vi "UI Main.vi"() -> ()   [LabVIEW 2018]
uses:
  controls/Raw Values.ctl
  controls/VENT SYSTEM.ctl
  controls/DECOUPLERS.ctl
  controls/LNG PUGE.ctl
  controls/Control 2.ctl
  controls/LNG PURGE INDICATORS.ctl
  controls/LOX PURGE.ctl
  controls/LOX PURGE INDICATORS.ctl
  controls/DECOUPLERS INDICATORS.ctl
  Shared Variables/Control 1.ctl
  controls/In Tank Raw Voltage Measure.ctl
  Labview Training/Project/FPGA Bitfiles/Control 3.ctl
  controls/SYSTEM MEASUREMENTS.ctl
  Shared Variables/He Flow indicator.ctl
  controls/FM Indicators.ctl
  controls/Pipeline T&P.ctl
  controls/In Tank T&P.ctl
  controls/UI Data.ctl
  controls/UI Data WVFM.ctl
  controls/All FPGA Configuration Values.ctl
  controls/FPGA State.ctl
  controls/Fill Valves.ctl
  support/Logging Configuration.ctl
  support/Message Queue/Message Cluster.ctl
  controls/PID Inputs.ctl
  Globals/Global - All UI Loop Stop.vi
  Globals/Global - UI Stream and Variable Connections.vi
  COMET  Extra Programs/Globals/Global - Configuration Options WVFM.vi
  Globals/Global - Configuration Options.vi
  support/User Event - Stop/User Event - Stop.lvlib
  support/Message Queue/Message Queue.lvlib
  support/Logging.lvlib
panel:
  in  "Expansion Chassis?":bool
  out "System Measurements":T1 {"LN2 [GPM]" scale=0.004..0.02; "LN2_Temp_Coil" scale=0.0..1.6; "LN2_Temp_HEX" scale=0.0..1.6; "LNG_DST 2" scale=0.0..1.6; "LOX_DST 2" scale=0.0..1.6; "LOX_MSP" scale=0.0..0.03; "LOX_MST" scale=0.0..1.6; "LNG_MSP" scale=0.0..0.03; "LNG_MST" scale=0.0..1.6; "LOX_UST" scale=0.0..1.6; "LNG_UST" scale=0.0..1.6; "LOX_USP" scale=0.004..0.02; "LNG_USP" scale=0.004..0.02; "N2_PURGE [CFM]" scale=0.004..0.02; "LOX_DSP" scale=0.0..0.03; "LOX_DST" scale=0.0..1.6; "LNG_DSP" scale=0.0..0.03; "LNG_DST" scale=0.0..1.6}
  in  "ARM":bool
  in  "Fire Mode":T2
  out "data out":dbl
  out "System Status 9049":string="\n"
  out "Connected 9049?":bool
  in  "Connect to Controller 9049":bool
  in  "Controller Address 9049":string="169.254.85.111"
  out "LOX USP1 hide":bool
  out "LOX DSP1 hide":bool
  out "LNG DSP1 hide":bool
  out "LNG USP1 hide":bool
  out "LOX VCV Fill Close":bool=TRUE
  out "LNG VCV Fill Close":bool=TRUE
  out "LOX BV Fill Open":bool
  out "LNG BV Fill Open":bool
  in  "Exit":bool
  in  "Switch to Safe State":bool
  out "System Status":string="\n2/13/2019 8:44:05 AM: UI Error -1950679035 - Read Variable in UI Main.vi\n7/27/2018 6:11:27 PM: UI Error -1950678941 - Read Single Element from Stream in UI - Read Stream from RT 9049.vi->UI Main.vi\n12/4/2017 2:15:53 PM: UI Error -314004 - Create Network Stream Writer Endpoint in UI - Initiate Connection.vi->UI Main.vi\n12/4/2017 2:15:31 PM: UI Error -314004 - Create Network Stream Writer Endpoint in UI - Initiate Connection.vi->UI Main.vi"
  out "Current FPGA Control Mode":u16(ring) items=["Safe State", "Manual", "Control (PID)"]
  in  "Settings Tab":T3(tab)=enum."Raw Values"
  in  "Pressure\nControl":bool=TRUE
  in  "ABORT DCs":bool
  in  "MANUAL PURGE":bool
  out "LNG LOWER VOL":dbl
  out "LNG UPPER VOL":dbl
  out "LOX LOWER VOL":dbl
  out "LOX UPPER VOL":dbl
  in  "Save As Button":bool
  in  "Record Button":bool
  out "DECOUPLERS INDICATORS":T4
  out "LOX PURGE INDICATORS":T5
  in  "LOX PURGE":T6
  out "LNG PURGE INDICATORS":T7
  out "VENT SYSTEM INDICATORS":T8
  out "Boolean":bool
  in  "VENT SYSTEM":T9
  in  "Run Control":bool
  in  "Stop Control":bool
  out "9039 Time":timestamp
  in  "LNG PURGE":T10
  in  "DECOUPLERS":T11
  in  "FILL VALVES":T12 {"LOX_VCV_CTL" min=0 max=100 scale=0.0..100.0 scale format="%#_3g"; "LNG_VCV_CTL" min=0 max=100 scale=0.0..100.0 scale format="%#_3g"}
  out "Fill Valves INDICATORS":T13 {"LOX_VCV_POS" format="%.1f"; "LNG_VCV_POS" format="%.1f"}
  out "IN TANK MEASUREMENTS":T14={"LOX_ULEGE [psi]"=-0.625, "LOX_TANK"=0.0, "LOX 90%"=FALSE, "LOX 105%"=FALSE, "Depth [in] LOX "=0.0, "LNG_TANK"=217.78724947643977, "LNG 90%"=TRUE, "LNG 105%"=TRUE, "Depth [in] LNG"=41.59736465, "LNG_ULEGE [psi]"=-0.625} {"LNG_ULEGE [psi]" scale=0.0..100.0; "LNG_TANK" scale=0.0..110.0; "LOX_TANK" scale=0.0..110.0; "LOX_ULEGE [psi]" scale=0.0..100.0}
  out "9049 Time":timestamp
  in  "Reset  4":bool
  out "Total LNG DSN2 [sec]":dbl
  out "LNG DSN2 [sec]":dbl
  out "Total LOX DSN2 [sec]":dbl
  in  "Reset  6":bool
  out "LOX USN2 [sec]":dbl
  in  "Reset  5":bool
  out "Total LOX USN2 [sec]":dbl
  out "LOX DSN2 [sec]":dbl
  out "Total LNG USN2 [sec]":dbl
  out "LNG USN2 [sec]":dbl
  in  "Reset  3":bool
  out "Fill height in manual?":bool
  out "LNG Mole Unbalanced?":bool
  out "Actual Mass Ratio":dbl
  out "LNG Mass [lbs]":dbl
  out "LOX Mass [lbs]":dbl
  out "Target Mass Ratio":dbl
  out "Tank Size":T15(ring)=enum."20000lbs"
  out "Target LNG Depth [in]":dbl
  out "Target LOX Depth [in]":dbl
  out "He Flow Indicator":T16 {"LNG_HE_MFC" scale=0.0..10.0; "LOX_HE_MFC" scale=0.0..10.0}
  out "FM Meausrements":T17 {"LNG_FMF [GPM]" scale=0.0..200.0; "LOX_FMF [GPM]" scale=0.0..200.0; "LNG_FMP [psi]" scale=0.0..100.0; "LOX_FMP [psi]" scale=0.0..100.0; "LOX_FMT [F]" scale=-300.0..100.0; "LNG_FMT [F]" scale=-300.0..100.0}
  out "Pipeline T&P":T18 {"LOX UST" scale=0.0..100.0; "LOX MST" scale=0.0..100.0; "LOX DST" scale=0.0..100.0; "LNG UST" scale=0.0..100.0; "LNG MST" scale=0.0..100.0; "LNG DST" scale=0.0..100.0; "LOX USP" scale=0.0..10.0; "LOX MSP" scale=0.0..10.0; "LOX DST" scale=0.0..10.0; "LNG USP" scale=0.0..10.0; "LNG MSP" scale=0.0..10.0; "LNG DSP" scale=0.0..10.0}
  out "In Tank T&P":T19 {"LOX Tank Temp.[F]" scale=0.0..100.0; "LOX Tank Press. [psi]" scale=0.0..10.0; "LNG Tank Temp. [F]" scale=0.0..100.0; "LNG Tank Press. [psi]" scale=0.0..10.0}
  in  "NGV_N2":bool
  in  "Pessure PID":T20
  out "9237 Live Data 9049":waveform(dbl)(graph)
  in  "9237 Live Data Channel 9049":u32 max=7 step=1
  in  "9222 Live Data Channel 9049":u32 max=27 step=1
  in  "Acquire Live Data 9222 9049":bool
  in  "Acquire Live Data 9237 9049":bool
  out "9222 Live Data 9049":waveform(dbl)(graph)
  out "Most recent manually-triggered log file 9222 9049":path
  in  "Acquire Live Data 9222":bool
  in  "Force Trigger":bool
  out "Most recent manually-triggered log file 9237":path
  in  "Stop Live Data 9039":bool
  in  "Acquire Live Data 9237":bool
  in  "9237 Live Data Channel 9039":u32 max=7 step=1
  out "9237 Live Data 9039":waveform(dbl)(graph)
  out "Current Logging State 9039":u16(ring) items=["Logging", "Idle (Safe State)"]
  out "9039 Time":timestamp
  out "9222 Live Data 9039":waveform(dbl)(graph)
  in  "9222 Live Data Channel 9039":u32 max=27 step=1
  out "Most recent manually-triggered log file 9222":path
  out "9049 Time":timestamp
  out "Most recent manually-triggered log file 9237 9049":path
  in  "Stop Live Data 9049":bool
  out "Current Logging State 9049":u16(ring) items=["Logging", "Idle (Safe State)"]
  out "Actual Loop Period (ticks)":u32
  out "Largest Contiguous Memory (bytes) 9039":dbl(graph)
  out "Resource Utilization (%) 9039":cluster{dbl, "Double":dbl, "Double":dbl}(graph)
  out "Number of FIles 9039":i16
  out "Resource Utilization (%) 9049":cluster{dbl, "Double":dbl, "Double":dbl}(graph)
  out "Largest Contiguous Memory (bytes) 9049":dbl(graph)
  out "Number of FIles 9049":i16
  out "LOX":T21(graph)
  out "LNG":T22(graph)
  in  "LOX DSP Voltage Offset":dbl
  in  "LNG DSP Voltage Offset":dbl=-0.0002
  in  "N2 Voltage Offset":dbl=-0.06
  out "IN TANK MEASUREMENTS DEPTH INCHES":T23={"LNG_TANK"=41.59736465, "LOX_TANK"=0.0, "LNG_TANK 2"=10.366875, "LOX_TANK 2"=0.0} {"LOX_TANK 2" format="%_6f"; "LNG_TANK 2" format="%_6f"; "LOX_TANK" format="%_6f"; "LNG_TANK" format="%_6f"}
  in  "TTL Signals":T24
  in  "Raw Values":T25 {"LOX_VCV_POS" scale=0.0..10.0; "LNG_VCV_POS" scale=0.0..10.0}
  in  "Run Manual":bool
  in  "Stop Manual":bool
  out "SYSTEM MEASUREMENTS RAW VOLTAGE and CURRENT":T26 {"LOX_MST" format="%.4f"; "LOX_UST" format="%.4f"; "LOX_DST 2" format="%.4f"; "LOX_MSP" format="%.6f"; "LOX_USP" format="%.6f"; "LNG_MSP" format="%.6f"; "LNG_DST 2" format="%.4f"; "LNG_USP" format="%.4f"; "LNG_MST" format="%.4f"; "LNG_UST" format="%.4f"; "N2_fLOW" format="%.4f"; "LOX_FLOW" format="%.4f"; "LNG_FLOW" format="%.4f"; "LOX_DSP" format="%.6f"; "LOX_DST" format="%.4f"; "LNG_DSP" format="%.6f"; "LNG_DST" format="%.4f"; "LOX_FMP" format="%.4f"; "LNG_FMP" format="%.4f"; "LOX_FMT" format="%.4f"; "LNG_FMT" format="%.4f"}
  out "IN TANK MEASUREMENTS RAW VOLTAGE 2":T27 {"LNG_TANK_ULEGE 2" format="%_6f"; "LNG_TANK_ULEGE" format="%_6f"; "LOX_TANK_ULEGE 2" format="%_6f"; "LNG_TANK 2" format="%_6f"; "LOX_TANK 2" format="%_6f"; "LOX_DIFF" format="%_6f"; "LNG_DIFF" format="%_6f"; "LOX_TANK_ULEGE" format="%_6f"}
  in  "Manual Temp Input?":bool
  in  "Backup Sensors":T28
  in  "Tank Type":T29(ring)
  in  "Tank Size 2":T15(ring)=enum."20000lbs"
  in  "LNG Fraction":T30
  in  "Tank Sensor Adjustment":T31={"LNG THP Slope"=1.1743, "LNG THP int"=-6262.0, "LOX THP Slope"=1.1733, "LOX THP int"=-0.609, "LOX UP Slope"=1.18, "LOX UP int"=-0.6428, "LOX THP int 2"=-1.2215, "LOX THP Slope 2"=1.2498, "LNG THP int 2"=-1.2262, "LNG THP Slope 2"=1.2456, "LOX UP int 2"=-1.2057, "LOX UP Slope 2"=1.2434, "LNG UP Slope"=1.1733, "LNG UP int"=-0.6223, "LNG UP int 2"=-1.2295, "LNG UP Slope 2"=1.2441} {"LNG UP Slope 2" format="%#_13g"; "LNG UP int 2" format="%#_13g"; "LNG UP int" format="%#_13g"; "LNG UP Slope" format="%#_13g"; "LOX UP Slope 2" format="%#_13g"; "LOX UP int 2" format="%#_13g"; "LNG THP Slope 2" format="%#_13g"; "LNG THP int 2" format="%#_13g"; "LOX THP Slope 2" format="%#_13g"; "LOX THP int 2" format="%#_13g"; "LOX UP int" format="%#_13g"; "LOX UP Slope" format="%#_13g"; "LOX THP int" format="%#_13g"; "LOX THP Slope" format="%#_13g"; "LNG THP int" format="%#_13g"; "LNG THP Slope" format="%#_13g"}
  out "Connected 9039?":bool
  in  "Connect to Controller 9039":bool
  in  "Controller Address 9039":string="169.254.16.244"
  # "Not rellevant, keep hidden"
  # "COMET CONTROLS AND DAQ"
  # "Connection Settings"
  # "Offset typ 2.1V"
  # "Offset typ .0001V"
  # "Offset typ 0V"
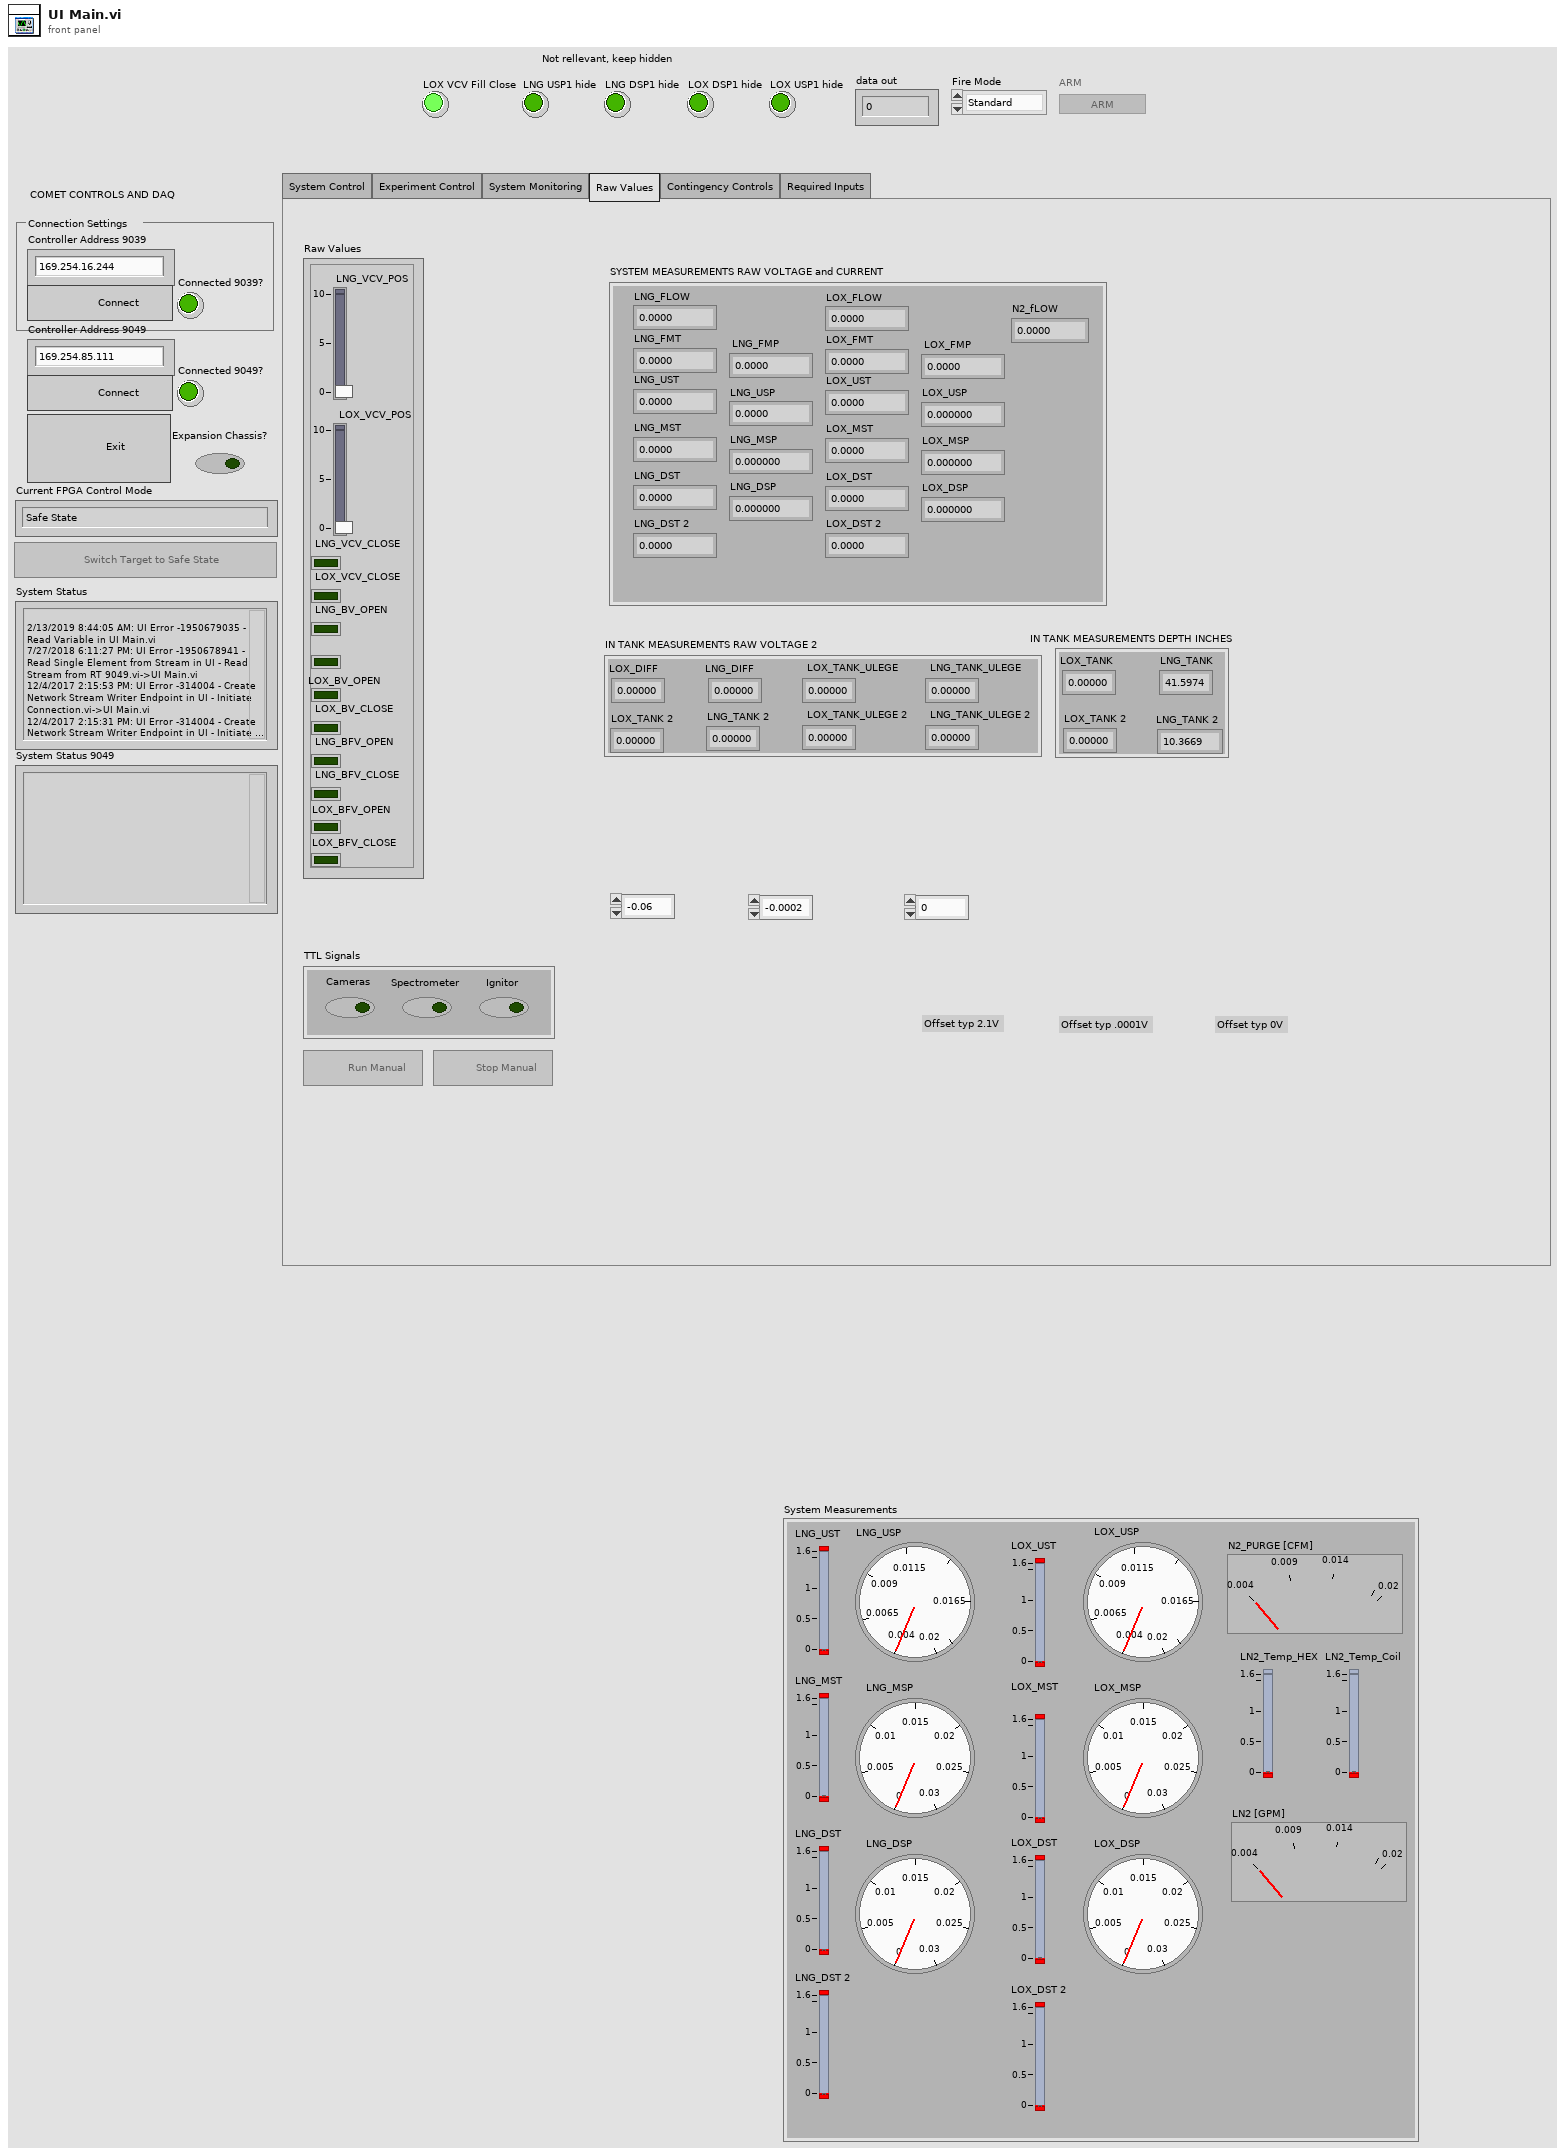
[diagram p1: front panel]
types:
  T1 = typedef "SYSTEM MEASUREMENTS.ctl" = cluster{"LNG_DST":sgl, "LNG_DSP":sgl, "LOX_DST":sgl, "LOX_DSP":sgl, "N2_PURGE [CFM]":sgl, "LNG_USP":sgl, "LOX_USP ":sgl, "LNG_UST":sgl, "LOX_UST":sgl, "LNG_MST":sgl, "LNG_MSP":sgl, "LOX_MST\n":sgl, "LOX_MSP":sgl, "LOX_DST 2":sgl, "LNG_DST 2":sgl, "LN2_Temp_HEX":sgl, "LN2_Temp_Coil":sgl, "LN2 [GPM]":sgl}
  T2 = typedef "Control 2.ctl" = enum16{"Standard", "Grill", "ROFI"}
  T3 = enum32{"System Control", "Experiment Control", "System Monitoring", "Raw Values", "Contingency Controls", "Required Inputs"}
  T4 = typedef "DECOUPLERS INDICATORS.ctl" = cluster{"LNG_DC_ENGAGED":bool, "LOX_DC_ENGAGED":bool, "LNG_DC_PROX":bool, "LOX_DC_PROX":bool}
  T5 = typedef "LOX PURGE INDICATORS.ctl" = cluster{"LOX_USP1":bool, "LOX_DSP1":bool}
  T6 = typedef "LOX PURGE.ctl" = cluster{"LOX_USP":bool, "LOX_DSP":bool}
  T7 = typedef "LNG PURGE INDICATORS.ctl" = cluster{"LNG_USP1":bool, "LNG_DSP1":bool}
  T8 = cluster{"LNG_BFV_CLOSE":bool, "LOX_BFV_CLOSE":bool, "LNG_BFV_OPEN":bool, "LOX_BFV_OPEN":bool}
  T9 = typedef "VENT SYSTEM.ctl" = cluster{"LNG_BFV":bool, "LOX_BFV":bool, "NGV_GV":bool}
  T10 = typedef "LNG PUGE.ctl" = cluster{"LNG_USP":bool, "LNG_DSP":bool}
  T11 = typedef "DECOUPLERS.ctl" = cluster{"LNG_DC":bool, "LOX_DC":bool, "NGV_DC":bool}
  T12 = cluster{"LOX_BV":bool, "LNG_BV":bool, "LNG_VCV_CTL":sgl, "LOX_VCV_CTL":sgl}
  T13 = cluster{"LNG_BV_CLOSE":bool, "LOX_BV_CLOSE":bool, "LNG_VCV_CLOSE":bool, "LNG_VCV_POS":sgl, "LOX_VCV_POS":sgl, "LNG_BV_OPEN":bool, "LOX_BV_OPEN":bool, "LOX_VCV_CLOSE":bool}
  T14 = typedef "Control 1.ctl" = cluster{"LOX_ULEGE [psi]":dbl, "LOX_TANK":dbl, "LOX 90%":bool, "LOX 105%":bool, "Depth [in] LOX ":dbl, "LNG_TANK":dbl, "LNG 90%":bool, "LNG 105%":bool, "Depth [in] LNG":dbl, "LNG_ULEGE [psi]":dbl}
  T15 = enum16{"", "150000lbs", "500lbs", "20000lbs", "9000lbs", "8000lbs", "4000lbs", "3000lbs", "2000lbs", "1000lbs"}
  T16 = typedef "He Flow indicator.ctl" = cluster{"LOX_HE_MFC":i16, "LNG_HE_MFC":i16}
  T17 = typedef "FM Indicators.ctl" = cluster{"LNG_FMT [F]":sgl, "LOX_FMT [F]":sgl, "LOX_FMP [psi]":sgl, "LNG_FMP [psi]":sgl, "LOX_FMF [GPM]":sgl, "LNG_FMF [GPM]":sgl}
  T18 = typedef "Pipeline T&P.ctl" = cluster{"LOX UST":sgl, "LOX MST":sgl, "LOX DST":sgl, "LNG UST":sgl, "LNG MST":sgl, "LNG DST":sgl, "LOX USP":sgl, "LOX MSP":sgl, "LOX DST":sgl, "LNG USP":sgl, "LNG MSP":sgl, "LNG DSP":sgl}
  T19 = typedef "In Tank T&P.ctl" = cluster{"LOX Tank Temp.[F]":sgl, "LOX Tank Press. [psi]":sgl, "LNG Tank Temp. [F]":sgl, "LNG Tank Press. [psi]":sgl}
  T20 = typedef "Control 3.ctl" = cluster{"Set Point [psi]":dbl, "Proportional (K)":dbl, "Integral (I)":dbl, "Derivative (D)":dbl}
  T21 = cluster{"LOX_VCV_POS":sgl, "LOX_FMF [GPM]":sgl, "LOX_FMT [F]":sgl, "LOX_FMP [psi]":sgl, "LOX_DST 2":sgl, "LOX_DSP":sgl, "LOX_UST":sgl, "LOX_USP ":sgl, "LOX_MST\n":sgl, "LOX_MSP":sgl}
  T22 = cluster{"LNG_VCV_POS":sgl, "LNG_FMF [GPM]":sgl, "LNG_FMT [F]":sgl, "LNG_FMP [psi]":sgl, "LNG_DST 2":sgl, "LNG_DSP":sgl, "LNG_UST":sgl, "LNG_USP":sgl, "LNG_MST":sgl, "LNG_MSP":sgl}
  T23 = cluster{"LNG_TANK":dbl, "LOX_TANK":dbl, "LNG_TANK 2":dbl, "LOX_TANK 2":dbl}
  T24 = cluster{"Cameras":bool, "Spectrometer":bool, "Ignitor":bool}
  T25 = typedef "Raw Values.ctl" = cluster{"LNG_VCV_POS":i16, " LOX_VCV_POS":i16, "LNG_VCV_CLOSE":bool, "LOX_VCV_CLOSE":bool, "LNG_BV_OPEN":bool, "LNG_BV_CLOSE":bool, "LOX_BV_OPEN":bool, "LOX_BV_CLOSE":bool, "LNG_BFV_OPEN":bool, "LNG_BFV_CLOSE":bool, "LOX_BFV_OPEN":bool, "LOX_BFV_CLOSE":bool}
  T26 = cluster{"LNG_FMT":sgl, "LOX_FMT":sgl, "LNG_FMP":sgl, "LOX_FMP":sgl, "LNG_DST":sgl, "LNG_DSP":sgl, "LOX_DST":sgl, "LOX_DSP":sgl, "LNG_FLOW [GPM]":sgl, "LOX_FLOW [GPM]":sgl, "N2_PURGE [CFM]":sgl, "LNG_UST":sgl, "LNG_MST":sgl, "LNG_USP":sgl, "LNG_DST 2":sgl, "LNG_MSP":sgl, "LOX_USP":sgl, "LOX_MSP":sgl, "LOX_DST 2":sgl, "LOX_UST":sgl, "LOX_MST":sgl}
  T27 = typedef "In Tank Raw Voltage Measure.ctl" = cluster{"LOX_TANK_ULEGE":sgl, "LNG_DIFF":sgl, "LOX_DIFF":sgl, "LOX_TANK 2":sgl, "LNG_TANK 2":sgl, "LOX_TANK_ULEGE 2":sgl, "LNG_TANK_ULEGE":sgl, "LNG_TANK_ULEGE 2":sgl}
  T28 = cluster{"LOX Tank Backup":bool, "LNG Tank Backup":bool, "LOX Ullage Backup":bool, "LNG Ullage Backup":bool}
  T29 = enum16{"Drop", "MOX", "CBM", "CBGS-New", "CBGS-Old"}
  T30 = cluster{"Methane":dbl, "Ethane":dbl, "Nitrogen":dbl, "Propane":dbl, "Isobutane":dbl}
  T31 = cluster{"LNG THP Slope":dbl, "LNG THP int":dbl, "LOX THP Slope":dbl, "LOX THP int":dbl, "LOX UP Slope":dbl, "LOX UP int":dbl, "LOX THP int 2":dbl, "LOX THP Slope 2":dbl, "LNG THP int 2":dbl, "LNG THP Slope 2":dbl, "LOX UP int 2":dbl, "LOX UP Slope 2":dbl, "LNG UP Slope":dbl, "LNG UP int":dbl, "LNG UP int 2":dbl, "LNG UP Slope 2":dbl}
  T32 = typedef "UI Data WVFM.ctl" = cluster{"Acquire Live Data 9237 9039":refnum<vi>, "Stop Live Data 9039":refnum<vi>, "Force Trigger":refnum<vi>, "Acquire Live Data 9222 9039":refnum<vi>, "Acquire Live Data 9237 9049":refnum<vi>, "Stop Live Data 9049":refnum<vi>, "Acquire Live Data 9222 9049":refnum<vi>}
  T33 = typedef "UI Data.ctl" = cluster{"Switch to Safe State Ref":refnum<vi>, "Run Manual Ref":refnum<vi>, "Stop Manual Ref":refnum<vi>, "Run Control Ref":refnum<vi>, "Stop Control Ref":refnum<vi>, "Update Control Configurations Ref":refnum<vi>, "Control Configurations Ref":refnum<vi>, "LNG_BV":refnum<vi>, "LOX_BV":refnum<vi>, "LOX DC":refnum<vi>, "LNG DC":refnum<vi>, "Record Button":refnum<vi>, "NGV DC":refnum<vi>, "LNG BFV":refnum<vi>, "LOX BFV":refnum<vi>, "Fill Valves":refnum<vi>, "VENT SYSTEM":refnum<vi>, "DECOUPLERS":refnum<vi>, "LNG Purge System":refnum<vi>, "LOX Purge System":refnum<vi>, "LOX_VCV":refnum<vi>, "LNG_VCV":refnum<vi>, "NGV N2":refnum<vi>, "MANUAL PURGE":refnum<vi>, "Turn on Pressure Control":refnum<vi>, "Pressure PID":refnum<vi>}
  T34 = typedef "Message Queue.lvlib/All Message Queues.ctl" = cluster{"UI":refnum<queue>, "UI System Record":refnum<queue>}
  T35 = cluster{"Message":string, "Message Data":variant}
  T36 = typedef "All FPGA Configuration Values.ctl" = cluster{"FPGA State":T37, "Manual Values":T25, "Fill Valves":T38, "LNG Purge System":T10, "LOX Purge System":T6, "DECOUPLERS":T11, "VENT SYSTEM":T9}
  T37 = typedef "FPGA State.ctl" = enum16{"Safe State", "Manual", "Control"}
  T38 = typedef "Fill Valves.ctl" = cluster{"LOX_BV":bool, "LNG_BV":bool, "LNG_VCV_CTL":sgl, "LOX_VCV_CTL":sgl}
  T39 = typedef "Message Queue.lvlib/Message Cluster.ctl" = cluster{"Message":string, "Message Data":variant}
  T40 = typedef "PID Inputs.ctl" = cluster{"Setpoint":dbl, "proportional gain (Kc)":dbl, "integral time (Ti, min)":dbl, "derivative time (Td, min)":dbl, "output high":dbl, "output low":dbl}
  T41 = enum8{"Enabled", "Disabled", "Disabled and Grayed Out"}
  T42 = typedef "Variable References.ctl" = cluster{"CPU Usage":refnum<k21>, "Contiguous Memory":refnum<k21>, " VALVE POSITIONS":refnum<k21>, "FPGA Mode":refnum<k21>, "Actual Loop Period":refnum<k21>, "FILL VALVES IND":refnum<k21>, "VENT SYSTEM IND":refnum<k21>, "LNG PURGE IND":refnum<k21>, "Drive Space":refnum<k21>, "Buffer Backlog":refnum<k21>, "System Time":refnum<k21>, "Number of Data Files":refnum<k21>, "LOX PURGE IND":refnum<k21>, "SYSTEM MEASURMENTS":refnum<k21>, "TEST TANK MEASURMENTS":refnum<k21>, "DECOUPLERS IND":refnum<k21>, "CPU Usage 9049":refnum<k21>, "Contiguous Memory 9049":refnum<k21>, "Drive Space 9049":refnum<k21>, "Buffer Backlog 9049":refnum<k21>, "Actual Loop Period 9049":refnum<k21>, "System Time 9049":refnum<k21>, "Number of Data Files 9049":refnum<k21>, "Number of Data Files 9050":refnum<k21>, "FM indicators":refnum<k21>, "He Flow indicator":refnum<k21>, "Pipeline T&P":refnum<k21>, "In tank T&P":refnum<k21>}
  T43 = cluster{"CPU Usage 9049":refnum<k21>, "Contiguous Memory 9049":refnum<k21>, "Drive Space 9049":refnum<k21>, "Buffer Backlog 9049":refnum<k21>, "Actual Loop Period 9049":refnum<k21>, "System Time 9049":refnum<k21>, "Number of Data Files 9049":refnum<k21>}
  T44 = typedef "Logging.lvlib/Logging Configuration.ctl" = cluster{"Log File Base Path":path, "TDMS File Reference":refnum<k34>, "Log File Path SYSTEM":path}
  T45 = enum16{"Left Button", "Center Button", "Right Button", "Window Close"}
  T46 = typedef "FILL VALVES INDICATORS.ctl" = cluster{"LNG_BV_CLOSE":bool, "LOX_BV_CLOSE":bool, "LNG_VCV_CLOSE":bool, "LNG_VCV_POS":sgl, "LOX_VCV_POS":sgl, "LNG_BV_OPEN":bool, "LOX_BV_OPEN":bool, "LOX_VCV_CLOSE":bool}
  T47 = typedef "VENT SYSTEM INDICATORS.ctl" = cluster{"LNG_BFV_CLOSE":bool, "LOX_BFV_CLOSE":bool, "LNG_BFV_OPEN":bool, "LOX_BFV_OPEN":bool}
  T48 = typedef "IN TANK MEASUREMENTS.ctl" = cluster{"LOX_TANK_ULEGE":sgl, "LNG_DIFF":sgl, "LOX_DIFF":sgl, "LOX_TANK 2":sgl, "LNG_TANK 2":sgl, "LOX_TANK_ULEGE 2":sgl, "LNG_TANK_ULEGE":sgl, "LNG_TANK_ULEGE 2":sgl}
  T49 = cluster{"Timestamp":timestamp, "Setpoint [psi]":dbl, "LOX Pressure [psi]":dbl, "LNG Pressure[psi]":dbl, "Diff. Pressure-Window [psi]":dbl, "LOX_HE_MFC":dbl, "LNG_HE_MFC":dbl}
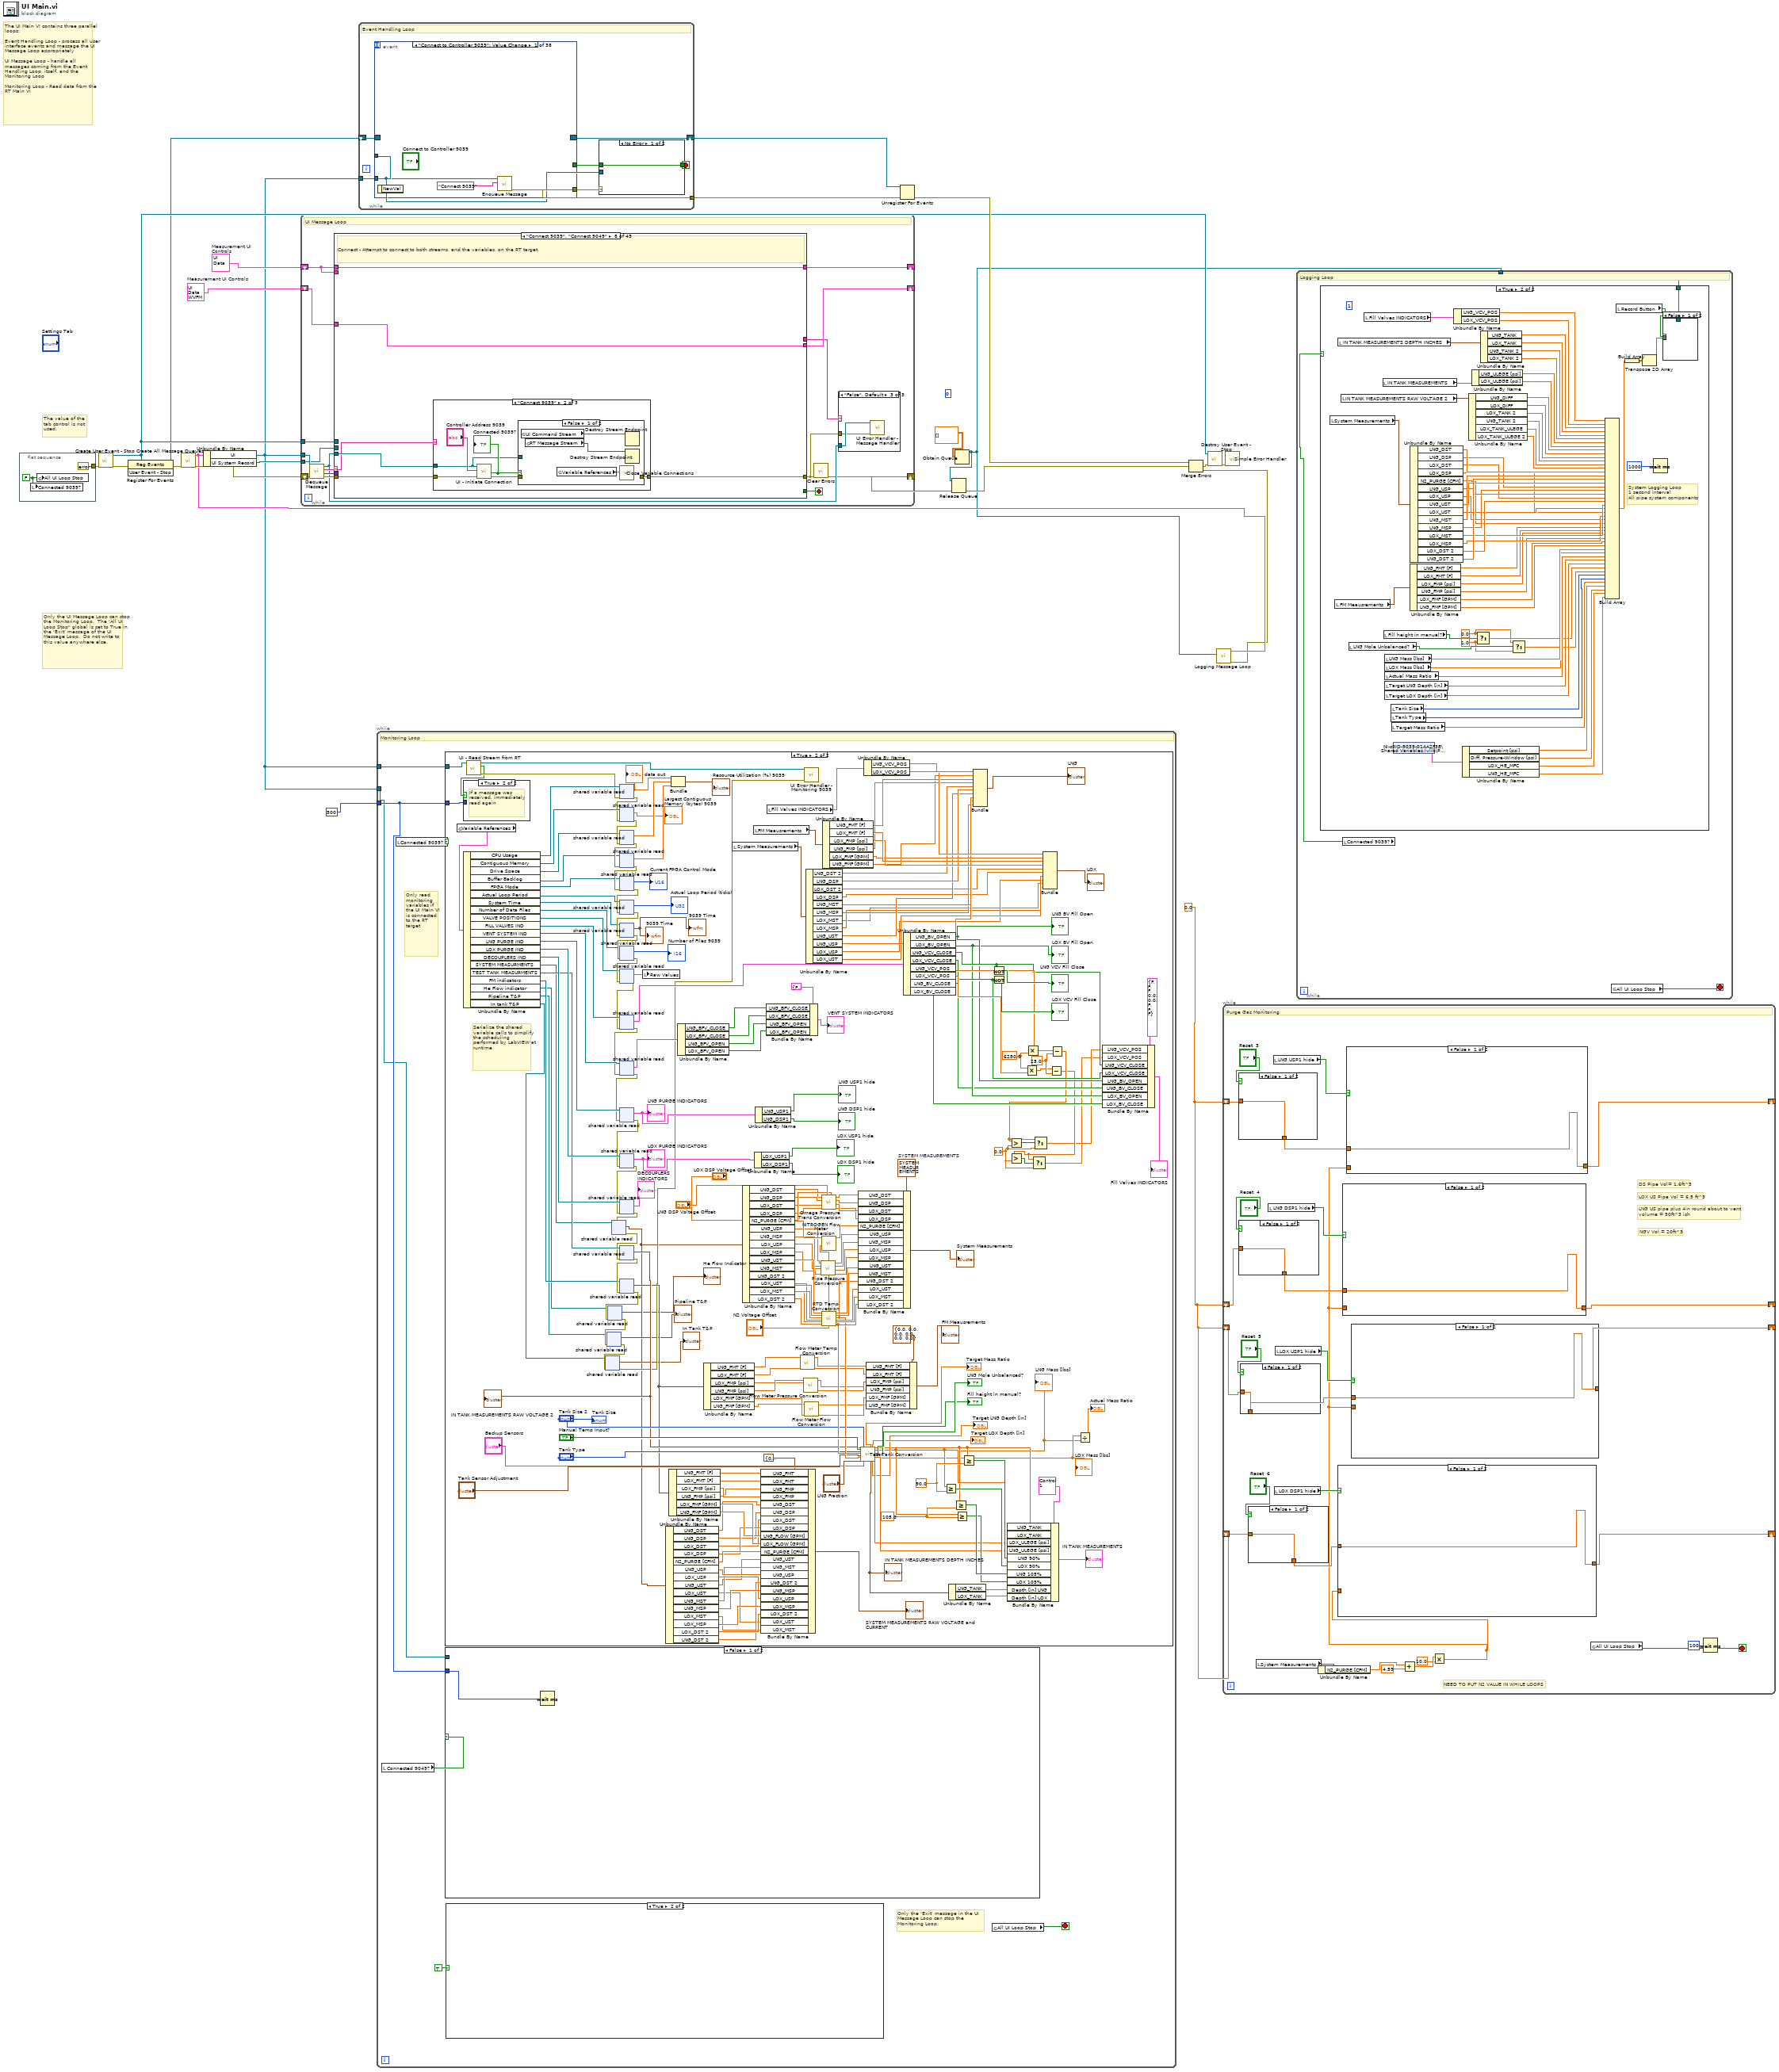
[diagram p0: block diagram]
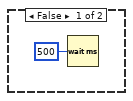
[diagram p2: hidden frame]
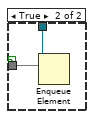
[diagram p3: hidden frame]
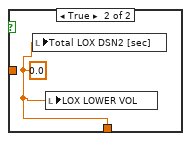
[diagram p4: hidden frame]
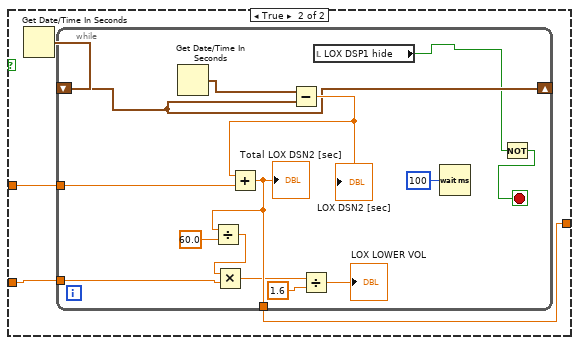
[diagram p5: hidden frame]
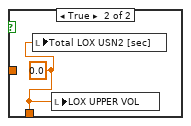
[diagram p6: hidden frame]
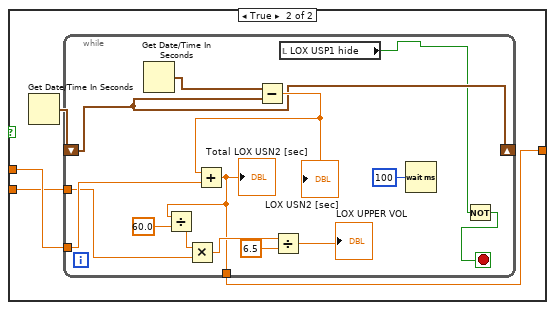
[diagram p7: hidden frame]
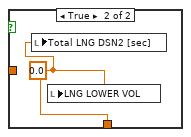
[diagram p8: hidden frame]
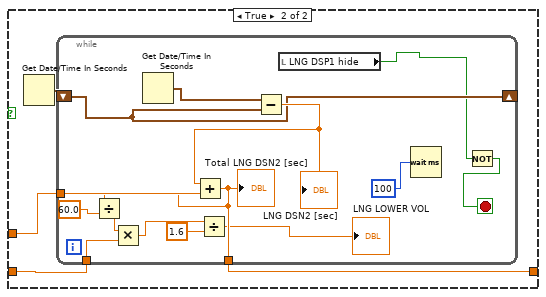
[diagram p9: hidden frame]
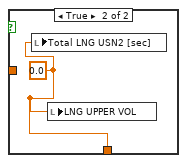
[diagram p10: hidden frame]
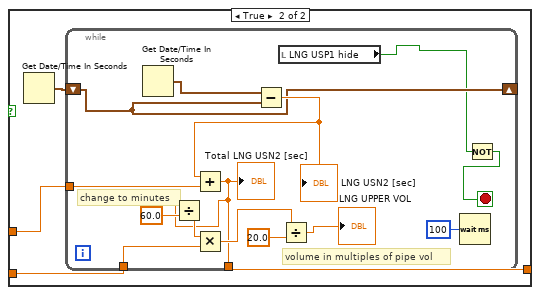
[diagram p11: hidden frame]
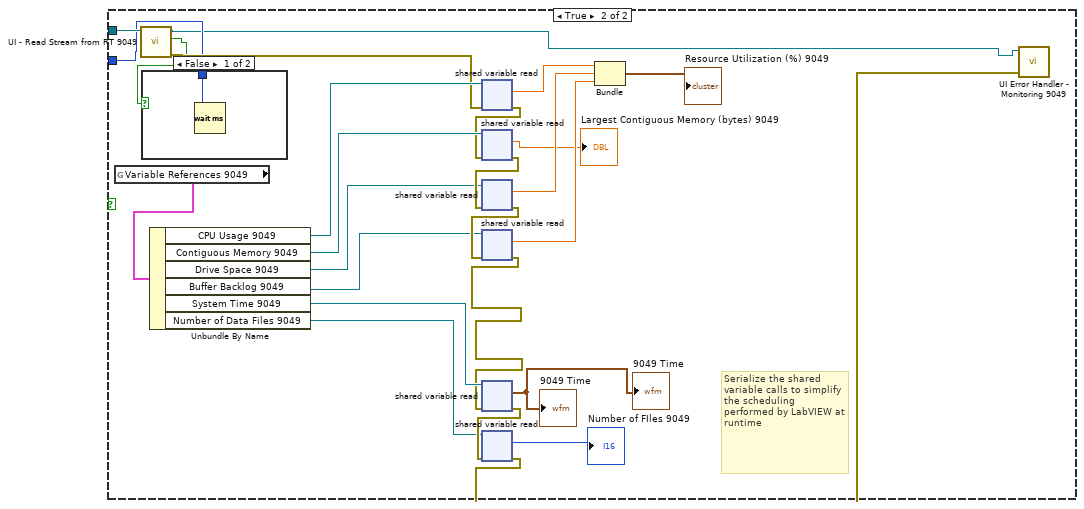
[diagram p13: hidden frame]
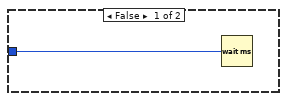
[diagram p15: hidden frame]
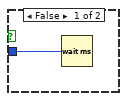
[diagram p16: hidden frame]
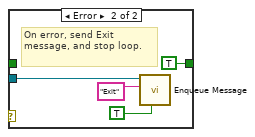
[diagram p17: hidden frame]
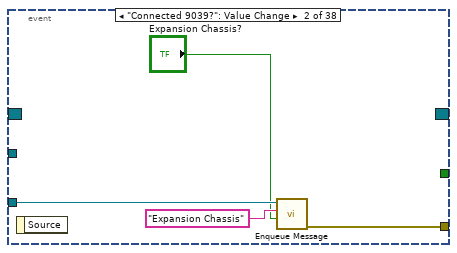
[diagram p18: hidden frame]
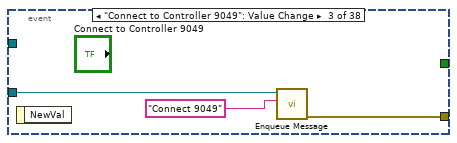
[diagram p19: hidden frame]
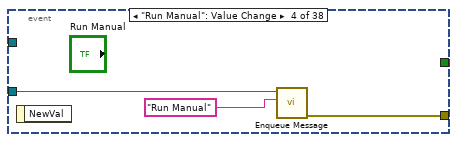
[diagram p20: hidden frame]
diagram:
  (unwired) i16 0 ("LOX_DST")
  w1 = 0.0
  w10 = T32 {"Acquire Live Data 9237 9039"=refnum, "Stop Live Data 9039"=refnum, "Force Trigger"=refnum, "Acquire Live Data 9222 9039"=refnum, "Acquire Live Data 9237 9049"=refnum, "Stop Live Data 9049"=refnum, "Acquire Live Data 9222 9049"=refnum}  # Measurement UI Controls
  w18 = T33 {"Switch to Safe State Ref"=refnum, "Run Manual Ref"=refnum, "Stop Manual Ref"=refnum, "Run Control Ref"=refnum, "Stop Control Ref"=refnum, "Update Control Configurations Ref"=refnum, "Control Configurations Ref"=refnum, "LNG_BV"=refnum, "LOX_BV"=refnum, "LOX DC"=refnum, "LNG DC"=refnum, "Record Button"=refnum, "NGV DC"=refnum, "LNG BFV"=refnum, "LOX BFV"=refnum, "Fill Valves"=refnum, "VENT SYSTEM"=refnum, "DECOUPLERS"=refnum, "LNG Purge System"=refnum, "LOX Purge System"=refnum, "LOX_VCV"=refnum, "LNG_VCV"=refnum, "NGV N2"=refnum, "MANUAL PURGE"=refnum, "Turn on Pressure Control"=refnum, "Pressure PID"=refnum}  # Measurement UI Controls
  # "The UI Main VI contains three parallel loops:\n\nEvent Handling Loop - process all user interface events and message the UI Message Loop appropriately\n\nUI Message Loop - handle all messages coming from the Event Handling Loop, itself, and the Monitoring Loop\n\nMonitoring Loop - Read data from the RT Main VI"
  # "The value of the tab control is not used."
  # "Only the UI Message Loop can stop the Monitoring Loop.  The 'All UI Loop Stop\" global is set to True in the 'Exit' message of the UI Message Loop.  Do not write to this value anywhere else."
  n1 = flat-sequence {
    tunnel: [errorcluster {"status"=FALSE, "code"=0, "source"=""} ("error in (no error)")] -> w16
    frame #0 {
      w24 = FALSE
      n2 = local write "Connected 9039?"(w24) -> ()
      n3 = global write "Global - All UI Loop Stop.vi" "All UI Loop Stop"(w24) -> ()
    }
  }
  n4 = call "Create User Event - Stop.vi"("error in (no error)"=w16) -> ("error out"=w14:errorcluster, "User Event - Stop"=w12:refnum<user-event>)  [unwired: 9 in]
  n5 = register-events(error in=w14, w12) -> (reference out=w11:refnum<event-registration>, error out=w13:errorcluster)  [unwired: 1 in]
  n6 = call "Create All Message Queues.vi"("error in (no error)"=w13) -> ("error out"=w21:errorcluster, "Message Queues out"=w8:T34)  [unwired: 9 in]
  n7 = Unbundle By Name(w8) -> ("UI"=w3:refnum<queue>, "UI System Record"=w9:refnum<queue>)
  n8 = while {
    tunnel: w3 -> [w35]
    tunnel: w12 -> [w40]
    shift-right: [w31] -> w5
    shift-left: w21 -> [w39]
    shift-right: [w34] -> _
    shift-left: w18 -> [w26]
    shift-right: [w29] -> _
    shift-left: w10 -> [w30]
    tunnel: w9 -> [w28]
    stop <- w41 stop-if-true
    # "UI Message Loop"
    n9 = call "Dequeue Message.vi"("error in (no error)"=w39, "Message Queue"=w35) -> ("error out"=w38:errorcluster, "Message Data"=w36:variant, "Message"=w37:string, "dup Message Queue"=w33:refnum<queue>)  [unwired: 6 in]
    n10 = case "Message Cases" shown="\"Connect 9039\", \"Connect 9049\"" w37 {
      selector: w37 -> [_ _ _ w101 _ _ w218 w231 w264 w284 _ _ w334 w355 w373 _ w405 w425 w450 w487 w525 w561 w588 w616 w638 w667 w681 w695 w705 w736 w747 _ _ _ _ w921 _ _ _ _ w1005 w1039 w1067]
      tunnel: w33 -> [w51 w75 w91 _ w204 w211 _ w234 _ w286 _ w322 w335 w356 _ _ _ _ _ _ _ _ _ _ _ _ _ _ _ _ _ _ _ _ w909 w925 _ _ w992 _ w1004 w1038 _]
      tunnel: w38 -> [w53 w84 w100 w104 w205 w215 w220 w236 w267 w288 w309 w331 w337 w358 w374 w388 w402 w423 w452 w489 w526 w562 w589 w617 w640 w668 w682 w696 w709 w741 w750 w769 w799 w863 w917 w934 w956 w975 w997 w1003 w1009 w1043 _]
      tunnel: [w52 w76 w92 w104 w205 w215 w217 w233 w267 w287 w308 w325 w336 w357 w375 w389 w404 w427 w447 w484 w527 w563 w590 w618 w639 w669 w683 w697 w709 w741 w750 w769 w798 w862 w911 w935 w954 w973 w998 w1002 w1008 w1042 w1065] -> w32
      tunnel: [_ _ _ _ _ _ _ _ _ _ _ _ _ _ _ _ _ _ _ _ _ _ _ _ _ _ _ _ _ _ _ _ _ _ _ _ _ _ TRUE _ _ _ _] -> w41
      tunnel: w36 -> [_ _ _ _ _ _ w219 _ _ _ _ w329 _ _ w372 w387 _ w424 w451 w488 w524 w558 w585 w613 _ w666 w680 w694 w708 w740 w749 _ w797 w861 w916 w932 w953 w972 _ _ _ _ _]
      tunnel: w40 -> [_ _ _ _ _ _ _ _ _ _ _ _ _ _ _ _ _ _ _ _ _ _ _ _ _ _ _ _ _ _ _ _ _ _ _ _ _ _ w996 _ _ _ _]
      tunnel: w26 -> [w54 w83 w99 w103 w206 w216 w223 w235 w266 w289 w310 w326 w338 w359 w376 w391 w407 w432 w453 w490 w521 w538 w583 w611 w643 w663 w677 w691 w711 w742 w751 w770 w778 w865 w915 w936 w955 w974 w994 w1001 w1007 w1041 w1063]
      tunnel: [w54 w82 w98 w103 w206 w216 w223 w235 w266 w289 w310 w326 w338 w359 w376 w391 w407 w432 w453 w490 w521 w538 w583 w611 w643 w663 w677 w691 w711 w742 w751 w770 w778 w865 w915 w936 w955 w974 w994 w1001 w1007 w1041 w1063] -> w34
      tunnel: w30 -> [w49 w73 w87 w102 w203 w213 w222 w232 w265 w285 w306 w321 w332 w353 w370 w384 w400 w430 w448 w485 w522 w559 w586 w614 w644 w664 w678 w692 w706 w739 w748 w768 w789 w864 w913 w919 w944 w964 w988 w1000 w1006 w1040 w1062]
      tunnel: [w49 w72 w87 w102 w203 w213 w222 w232 w265 w285 w306 w321 w332 w353 w370 w384 w400 w430 w448 w485 w522 w559 w586 w614 w644 w664 w678 w692 w706 w739 w748 w768 w789 w864 w913 w919 w944 w964 w988 w1000 w1006 w1040 w1062] -> w29
      tunnel: w28 -> [_ _ _ _ _ _ _ _ _ _ _ _ _ _ _ w390 w406 _ _ _ _ _ _ _ _ _ _ _ _ _ _ _ _ _ _ _ _ _ w985 _ _ _ _]
      tunnel: [_ _ _ _ _ _ _ _ _ _ _ _ _ _ _ _ _ _ _ _ _ _ _ _ _ _ _ _ _ _ _ _ _ _ _ w918 _ _ _ _ _ _ _] -> w27
      tunnel: w26 -> [_ _ _ _ _ _ _ _ _ _ _ _ _ _ _ _ _ _ _ _ _ _ _ _ _ _ _ _ _ _ _ _ _ w858 _ _ _ _ _ _ _ _ _]
      frame "Initialize" {
        # "Initialize - Send 'Initialize UI Refs' message to get the UI references bundled and initialized appropriately."
        n11 = local write "Pressure\nControl"(FALSE ("Pressurization Control")) -> ()
        n12 = call "Enqueue Message.vi"("error in (no error)"=w53, "Message"="Initialize UI Refs", "Message Queue"=w51) -> ("error out"=w52:errorcluster)  [unwired: 7 in, 1 out]
      }
      frame "Initialize UI Refs" {
        # "Send a message to disable them all, since there is no connection at the start."
        # "Initialize UI Refs - Bundle up a cluster of references of all UI elements that are programmatically manipulated."
        n13 = control-ref of="Record Button"() -> (w62:refnum<vi>)
        n14 = control-ref of="LOX PURGE"() -> (w63:refnum<vi>)
        n15 = control-ref of="FILL VALVES"() -> (w67:refnum<vi>)
        n16 = control-ref of="VENT SYSTEM"() -> (w66:refnum<vi>)
        n17 = control-ref of="DECOUPLERS"() -> (w64:refnum<vi>)
        n18 = control-ref of="PURGE SYSTEM"() -> (w65:refnum<vi>)
        n19 = control-ref of="LNG_VCV_CTL"() -> (w58:refnum<vi>)
        n20 = control-ref of="LOX_VCV_CTL"() -> (w57:refnum<vi>)
        n21 = control-ref of="Stop Live Data 9049"() -> (w60:refnum<vi>)
        n22 = control-ref of="Acquire Live Data 9222"() -> (w68:refnum<vi>)
        n23 = control-ref of="Acquire Live Data 9237 9049"() -> (w61:refnum<vi>)
        n24 = control-ref of="Force Trigger"() -> (w69:refnum<vi>)
        n25 = control-ref of="Stop Live Data 9039"() -> (w70:refnum<vi>)
        n26 = control-ref of="Acquire Live Data 9237"() -> (w71:refnum<vi>)
        n27 = control-ref of="Acquire Live Data 9222 9049"() -> (w59:refnum<vi>)
        n28 = control-ref of="Pressure\nControl"() -> (w55:refnum<vi>)
        n29 = control-ref of="Switch to Safe State"() -> (w81:refnum<vi>)
        n30 = control-ref of="Run Manual"() -> (w80:refnum<vi>)
        n31 = control-ref of="Stop Manual"() -> (w79:refnum<vi>)
        n32 = control-ref of="Run Control"() -> (w78:refnum<vi>)
        n33 = control-ref of="Stop Control"() -> (w77:refnum<vi>)
        n34 = control-ref of="Pessure PID"() -> (w56:refnum<vi>)
        n35 = call "Enqueue Message.vi"("error in (no error)"=w84, "Message"="Initialize UI Refs 2", "Message Queue"=w75) -> ("error out"=w76:errorcluster)  [unwired: 7 in, 1 out]
        n36 = Bundle By Name(cluster=w73, "Acquire Live Data 9237 9039"=w71, "Stop Live Data 9039"=w70, "Force Trigger"=w69, "Acquire Live Data 9222 9039"=w68, "Acquire Live Data 9237 9049"=w61, "Stop Live Data 9049"=w60, "Acquire Live Data 9222 9049"=w59) -> (w72:T32)
        n37 = Bundle By Name(cluster=w83, "Switch to Safe State Ref"=w81, "Run Manual Ref"=w80, "Stop Manual Ref"=w79, "Run Control Ref"=w78, "Stop Control Ref"=w77, "LOX Purge System"=w63, "Fill Valves"=w67, "VENT SYSTEM"=w66, "DECOUPLERS"=w64, "LNG Purge System"=w65, "Record Button"=w62, "LNG_VCV"=w58, "LOX_VCV"=w57, "Turn on Pressure Control"=w55, "Pressure PID"=w56) -> (w82:T33)
      }
      frame "Initialize UI Refs 2" {
        # "Send a message to disable them all, since there is no connection at the start."
        # "Initialize UI Refs - Bundle up a cluster of references of all UI elements that are programmatically manipulated."
        n38 = control-ref of="LNG_BV"() -> (w88:refnum<vi>)
        n39 = control-ref of="LOX_BV"() -> (w89:refnum<vi>)
        n40 = control-ref of="NGV_N2"() -> (w86:refnum<vi>)
        n41 = control-ref of="MANUAL PURGE"() -> (w85:refnum<vi>)
        n42 = control-ref of="LNG_DC"() -> (w97:refnum<vi>)
        n43 = control-ref of="LOX_DC"() -> (w96:refnum<vi>)
        n44 = control-ref of="NGV_DC"() -> (w95:refnum<vi>)
        n45 = control-ref of="LNG_BFV"() -> (w94:refnum<vi>)
        n46 = control-ref of="LOX_BFV"() -> (w93:refnum<vi>)
        n47 = call "Enqueue Message.vi"("error in (no error)"=w100, "Message"="Disable Controls", "Message Queue"=w91) -> ("error out"=w92:errorcluster)  [unwired: 7 in, 1 out]
        n48 = Bundle By Name(cluster=w99, "LNG DC"=w97, "LOX DC"=w96, "NGV DC"=w95, "LNG BFV"=w94, "LOX BFV"=w93, "LNG_BV"=w88, "LOX_BV"=w89, "NGV N2"=w86, "MANUAL PURGE"=w85) -> (w98:T33)
      }
      frame "Disable Controls", "Disable Controls 9039", "Disable Controls 9049" {
        # "Disable All Controls - Set all controls in the UI Refs cluster to \"Disabled and Grayed Out\"."
        n49 = case shown="\"Disable Controls\"" w101 {
          tunnel: w103 -> [_ w149 w190 _]
          tunnel: w102 -> [_ w126 w160 w195]
          frame "False", Default {
          }
          frame "Disable Controls" {
            w112 = 0
            # "Changed 1/7  LOX purge and below were not connected"
            # "With the control options disabled, the only thing the user can do is Connect. Make sure the IP address string and connect button are enabled."
            n50 = Unbundle(w149) -> ("Switch to Safe State Ref"=w148:refnum<vi>, "Run Manual Ref"=w147:refnum<vi>, "Stop Manual Ref"=w146:refnum<vi>, "Run Control Ref"=w145:refnum<vi>, "Stop Control Ref"=w144:refnum<vi>, "Update Control Configurations Ref"=w143:refnum<vi>, "Control Configurations Ref"=w142:refnum<vi>, "LNG_BV"=w141:refnum<vi>, "LOX_BV"=w140:refnum<vi>, "LOX DC"=w139:refnum<vi>, "LNG DC"=w138:refnum<vi>, "Record Button"=w137:refnum<vi>, "NGV DC"=w136:refnum<vi>, "LNG BFV"=w135:refnum<vi>, "LOX BFV"=w134:refnum<vi>, "Fill Valves"=w124:refnum<vi>, "VENT SYSTEM"=w123:refnum<vi>, "DECOUPLERS"=w122:refnum<vi>, "LNG Purge System"=w121:refnum<vi>, "LOX Purge System"=w108:refnum<vi>, "LOX_VCV"=w109:refnum<vi>, "LNG_VCV"=w110:refnum<vi>, "NGV N2"=w111:refnum<vi>, "MANUAL PURGE"=w107:refnum<vi>, "Turn on Pressure Control"=w106:refnum<vi>, "Pressure PID"=w105:refnum<vi>)
            n51 = Unbundle(w126) -> ("Acquire Live Data 9237 9039"=w130:refnum<vi>, "Stop Live Data 9039"=w129:refnum<vi>, "Force Trigger"=w128:refnum<vi>, "Acquire Live Data 9222 9039"=w125:refnum<vi>, "Acquire Live Data 9237 9049"=w115:refnum<vi>, "Stop Live Data 9049"=w114:refnum<vi>, "Acquire Live Data 9222 9049"=w113:refnum<vi>)
            n52 = control-ref of="Cameras"() -> (w120:refnum<vi>)
            n53 = control-ref of="Ignitor"() -> (w119:refnum<vi>)
            n54 = control-ref of="Spectrometer"() -> (w118:refnum<vi>)
            n55 = Build Array(w148, w147, w146, w145, w144, w143, w142, w141, w140, w139, w138, w137, w136, w135, w134, w124, w123, w122, w121, w108, w109, w110, w111, w107, w106, w105) -> (w133:refnum<vi>[])
            n56 = Build Array(w130, w129, w128, w125, w115, w114, w113) -> (w127:refnum<vi>[])
            n57 = Build Array(w120, w119, w118) -> (w116:refnum<vi>[])
            n58 = call "Set Enable State on Multiple Controls.vi"("Enable?"=FALSE, "Controls"=w127) -> ()  [unwired: 10 in]
            n59 = call "Set Enable State on Multiple Controls.vi"("Enable?"=FALSE, "Controls"=w133) -> ()  [unwired: 10 in]
            n60 = call "Set Enable State on Multiple Controls.vi"("Enable?"=TRUE, "Controls"=w116) -> ()  [unwired: 10 in]
            n61 = property on="Controller Address 9049" class="Str"("DisabledEnum"=w112) -> ()  [unwired: 2 in, 2 out]
            n62 = property on="Connect to Controller 9049" class="Bool"("DisabledEnum"=w112) -> ()  [unwired: 2 in, 2 out]
            n63 = property on="Controller Address 9039" class="Str"("DisabledEnum"=w112) -> ()  [unwired: 2 in, 2 out]
            n64 = property on="Connect to Controller 9039" class="Bool"("DisabledEnum"=w112) -> ()  [unwired: 2 in, 2 out]
          }
          frame "Disable Controls 9039" {
            w161 = 0
            # "With the control options disabled, the only thing the user can do is Connect. Make sure the IP address string and connect button are enabled."
            n65 = Unbundle By Name(w160) -> ("Acquire Live Data 9237 9039"=w159:refnum<vi>, "Stop Live Data 9039"=w158:refnum<vi>, "Acquire Live Data 9222 9039"=w157:refnum<vi>)
            n66 = Unbundle(w190) -> ("Switch to Safe State Ref"=w189:refnum<vi>, "Run Manual Ref"=w188:refnum<vi>, "Stop Manual Ref"=w187:refnum<vi>, "Run Control Ref"=w186:refnum<vi>, "Stop Control Ref"=w185:refnum<vi>, "Update Control Configurations Ref"=w184:refnum<vi>, "Control Configurations Ref"=w183:refnum<vi>, "LNG_BV"=w182:refnum<vi>, "LOX_BV"=w181:refnum<vi>, "LOX DC"=w180:refnum<vi>, "LNG DC"=w179:refnum<vi>, "Record Button"=w178:refnum<vi>, "NGV DC"=w177:refnum<vi>, "LNG BFV"=w176:refnum<vi>, "LOX BFV"=w175:refnum<vi>, "Fill Valves"=w171:refnum<vi>, "VENT SYSTEM"=w170:refnum<vi>, "DECOUPLERS"=w169:refnum<vi>, "LNG Purge System"=w168:refnum<vi>, "LOX Purge System"=w162:refnum<vi>, "LOX_VCV"=w155:refnum<vi>, "LNG_VCV"=w154:refnum<vi>, "NGV N2"=w153:refnum<vi>, "MANUAL PURGE"=w152:refnum<vi>, "Turn on Pressure Control"=w151:refnum<vi>, "Pressure PID"=w150:refnum<vi>)
            n67 = control-ref of="Cameras"() -> (w167:refnum<vi>)
            n68 = control-ref of="Ignitor"() -> (w166:refnum<vi>)
            n69 = control-ref of="Spectrometer"() -> (w165:refnum<vi>)
            n70 = Build Array(w189, w188, w187, w186, w185, w184, w183, w182, w181, w180, w179, w178, w177, w176, w175, w171, w170, w169, w168, w162, w155, w154, w153, w152, w151, w150) -> (w174:refnum<vi>[])
            n71 = Build Array(w167, w166, w165) -> (w163:refnum<vi>[])
            n72 = Build Array(w159, w158, w157) -> (w156:refnum<vi>[])
            n73 = call "Set Enable State on Multiple Controls.vi"("Enable?"=FALSE, "Controls"=w174) -> ()  [unwired: 10 in]
            n74 = call "Set Enable State on Multiple Controls.vi"("Enable?"=TRUE, "Controls"=w163) -> ()  [unwired: 10 in]
            n75 = call "Set Enable State on Multiple Controls.vi"("Enable?"=FALSE, "Controls"=w156) -> ()  [unwired: 10 in]
            n76 = property on="Controller Address 9039" class="Str"("DisabledEnum"=w161) -> ()  [unwired: 2 in, 2 out]
            n77 = property on="Connect to Controller 9039" class="Bool"("DisabledEnum"=w161) -> ()  [unwired: 2 in, 2 out]
          }
          frame "Disable Controls 9049" {
            w196 = 0
            # "With the control options disabled, the only thing the user can do is Connect. Make sure the IP address string and connect button are enabled."
            n78 = Unbundle By Name(w195) -> ("Acquire Live Data 9237 9049"=w194:refnum<vi>, "Stop Live Data 9049"=w193:refnum<vi>, "Acquire Live Data 9222 9049"=w192:refnum<vi>)
            n79 = Build Array(w194, w193, w192) -> (w191:refnum<vi>[])
            n80 = call "Set Enable State on Multiple Controls.vi"("Enable?"=FALSE, "Controls"=w191) -> ()  [unwired: 10 in]
            n81 = property on="Controller Address 9049" class="Str"("DisabledEnum"=w196) -> ()  [unwired: 2 in, 2 out]
            n82 = property on="Connect to Controller 9049" class="Bool"("DisabledEnum"=w196) -> ()  [unwired: 2 in, 2 out]
          }
        }
      }
      frame "Enable Configuration Controls" {
        w199 = 2
        # "Once connected, the user shouldn't be able to change the connection settings unless he gets disconnected."
        # "Enable Configuration Controls - After successful connection, ensure appropriate controls are enabled."
        n83 = case shown="False" TRUE {
          tunnel: w204 -> [w210 _]
          frame False {
            n84 = call "Enqueue Message.vi"("Message"="Get Status 9149", "Message Queue"=w210) -> ()  [unwired: 8 in, 2 out]
          }
          frame True {
          }
        }
        n85 = Unbundle By Name(w206) -> ("Update Control Configurations Ref"=w200:refnum<vi>, "LOX BFV"=w202:refnum<vi>, "LNG BFV"=w201:refnum<vi>)
        n86 = Build Array(w200, w202, w201) -> (w208:refnum<vi>[])
        n87 = call "Set Enable State on Multiple Controls.vi"("Enable?"=TRUE, "Controls"=w208) -> ()  [unwired: 10 in]
        n88 = property on="Controller Address 9039" class="Str"("DisabledEnum"=w199) -> ()  [unwired: 2 in, 2 out]
        n89 = property on="Connect to Controller 9039" class="Bool"("DisabledEnum"=w199) -> ()  [unwired: 2 in, 2 out]
      }
      frame "Enable Configuration Controls 9049" {
        w212 = 2
        # "Once connected, the user shouldn't be able to change the connection settings unless he gets disconnected."
        # "Enable Configuration Controls - After successful connection, ensure appropriate controls are enabled."
        n90 = call "Enqueue Message.vi"("Message"="Get Logging Status 9049", "Message Queue"=w211) -> ()  [unwired: 8 in, 2 out]
        n91 = property on="Controller Address 9049" class="Str"("DisabledEnum"=w212) -> ()  [unwired: 2 in, 2 out]
        n92 = property on="Connect to Controller 9049" class="Bool"("DisabledEnum"=w212) -> ()  [unwired: 2 in, 2 out]
      }
      frame "Manual Camera TTL", "Manual Ignitor TTL", "Manual Spectrometer TTL" {
        # "Enable Configuration Controls - After successful connection, ensure appropriate controls are enabled."
        n93 = local read "Connected 9039?"() -> (w221:bool)
        n94 = case shown="True" w221 {
          tunnel: [w224 w230] -> w217
          tunnel: w220 -> [w224 w228]
          tunnel: w218 -> [_ w227]
          tunnel: w219 -> [_ w226]
          frame False {
            # "Don't bother trying to send a message to the RT system if UI Main VI isn't even connected"
          }
          frame True {
            n95 = global read "Global - UI Stream and Variable Connections.vi" "UI Command Stream"() -> (w225:refnum<k21>)
            n96 = Bundle(w227, "Message Data"=w226) -> (w229:cluster{string, "Message Data":variant})  [unwired: 1 in]
            n97 = shared-variable-write(w225, w228, w229) -> (w230:errorcluster)  [unwired: 1 in, 2 out]
          }
        }
      }
      frame "Connect 9039", "Connect 9049" {
        # "Connect - Attempt to connect to both streams, and the variables, on the RT target."
        n98 = case shown="\"Connect 9039\"" w231 {
          tunnel: w236 -> [w237 w243 w256]
          tunnel: w234 -> [_ w239 w254]
          tunnel: [w237 w238 w257] -> w233
          frame "False", Default {
          }
          frame "Connect 9039" {
            n99 = call "UI - Initiate Connection.vi"("error in (no error)"=w243, "Controller Address"="Controller Address 9039", "Message Queue"=w239) -> ("error out"=w241:errorcluster, "Connected?"=w240:bool)  [unwired: 7 in]
            "Connected 9039?" <- w240
            n100 = case shown="False" w240 {
              tunnel: w241 -> [_ w251]
              tunnel: w239 -> [_ w250]
              tunnel: [_ w249] -> w238
              frame False {
                n101 = global read "Global - UI Stream and Variable Connections.vi" "UI Command Stream"() -> (w245:refnum<k21>)
                n102 = global read "Global - UI Stream and Variable Connections.vi" "RT Message Stream"() -> (w244:refnum<k21>)
                n103 = global read "Global - UI Stream and Variable Connections.vi" "Variable References"() -> (w246:T42)
                n104 = call "Close Variable Connections.vi"("Variable References"=w246) -> ()  [unwired: 11 in]
                n105 = Destroy Stream Endpoint(11:w245) -> ()  [unwired: 1 in, 1 out]
                n106 = Destroy Stream Endpoint(11:w244) -> ()  [unwired: 1 in, 1 out]
              }
              frame True {
                n107 = call "Enqueue Message.vi"("Priority Message? (F)"=TRUE, "error in (no error)"=w251, "Message"="Safe Start", "Message Queue"=w250) -> ("error out"=w249:errorcluster)  [unwired: 6 in, 1 out]
              }
            }
          }
          frame "Connect 9049" {
            n108 = call "UI - Initiate Connection 9049.vi"("error in (no error)"=w256, "Controller Address"="Controller Address 9049", "Message Queue"=w254) -> ("error out"=w253:errorcluster, "Connected?"=w252:bool)  [unwired: 7 in]
            "Connected 9049?" <- w252
            n109 = case shown="False" w252 {
              tunnel: w253 -> [_ w263]
              tunnel: w254 -> [_ w261]
              tunnel: [_ w263] -> w257
              frame False {
                n110 = global read "Global - UI Stream and Variable Connections.vi" "UI Command Stream 9049"() -> (w260:refnum<k21>)
                n111 = global read "Global - UI Stream and Variable Connections.vi" "RT Message Stream 9049"() -> (w259:refnum<k21>)
                n112 = global read "Global - UI Stream and Variable Connections.vi" "Variable References 9049"() -> (w258:T43)
                n113 = call "Close Variable Connections 9049.vi"("Variable References 9049"=w258) -> ()  [unwired: 11 in]
                n114 = Destroy Stream Endpoint(11:w260) -> ()  [unwired: 1 in, 1 out]
                n115 = Destroy Stream Endpoint(11:w259) -> ()  [unwired: 1 in, 1 out]
              }
              frame True {
                (unwired) TRUE ("Priority Message? (F)")
                n116 = call "Enqueue Message.vi"("Message"="Enable Configuration Controls 9049", "Message Queue"=w261) -> ()  [unwired: 8 in, 2 out]
              }
            }
          }
        }
      }
      frame "Close Connections", "Close Connections 9039", "Close Connections 9049" {
        # "Close Connections - Close the connections shared with the Monitoring Loop."
        n117 = case shown="\"Close Connections 9039\"" w264 {
          frame "False", Default {
          }
          frame "Close Connections" {
            n118 = global read "Global - UI Stream and Variable Connections.vi" "UI Command Stream"() -> (w275:refnum<k21>)
            n119 = global read "Global - UI Stream and Variable Connections.vi" "RT Message Stream"() -> (w274:refnum<k21>)
            n120 = global read "Global - UI Stream and Variable Connections.vi" "Variable References"() -> (w273:T42)
            n121 = local write "Connected 9039?"(FALSE ("Connected?")) -> ()
            n122 = Destroy Stream Endpoint(11:w275) -> ()  [unwired: 1 in, 1 out]
            n123 = Destroy Stream Endpoint(11:w274) -> ()  [unwired: 1 in, 1 out]
            n124 = call "Close Variable Connections.vi"("Variable References"=w273) -> ()  [unwired: 11 in]
            n125 = global read "Global - UI Stream and Variable Connections.vi" "Variable References 9049"() -> (w269:T43)
            n126 = global read "Global - UI Stream and Variable Connections.vi" "UI Command Stream 9049"() -> (w272:refnum<k21>)
            n127 = global read "Global - UI Stream and Variable Connections.vi" "RT Message Stream 9049"() -> (w271:refnum<k21>)
            n128 = local write "Connected 9049?"(FALSE ("Connected?")) -> ()
            n129 = Destroy Stream Endpoint(11:w272) -> ()  [unwired: 1 in, 1 out]
            n130 = Destroy Stream Endpoint(11:w271) -> ()  [unwired: 1 in, 1 out]
            n131 = call "Close Variable Connections 9049.vi"("Variable References 9049"=w269) -> ()  [unwired: 11 in]
          }
          frame "Close Connections 9039" {
            n132 = global read "Global - UI Stream and Variable Connections.vi" "UI Command Stream"() -> (w279:refnum<k21>)
            n133 = global read "Global - UI Stream and Variable Connections.vi" "RT Message Stream"() -> (w278:refnum<k21>)
            n134 = global read "Global - UI Stream and Variable Connections.vi" "Variable References"() -> (w277:T42)
            n135 = local write "Connected 9039?"(FALSE ("Connected?")) -> ()
            n136 = Destroy Stream Endpoint(11:w279) -> ()  [unwired: 1 in, 1 out]
            n137 = Destroy Stream Endpoint(11:w278) -> ()  [unwired: 1 in, 1 out]
            n138 = call "Close Variable Connections.vi"("Variable References"=w277) -> ()  [unwired: 11 in]
          }
          frame "Close Connections 9049" {
            n139 = global read "Global - UI Stream and Variable Connections.vi" "Variable References 9049"() -> (w281:T43)
            n140 = global read "Global - UI Stream and Variable Connections.vi" "UI Command Stream 9049"() -> (w283:refnum<k21>)
            n141 = global read "Global - UI Stream and Variable Connections.vi" "RT Message Stream 9049"() -> (w282:refnum<k21>)
            n142 = local write "Connected 9049?"(FALSE ("Connected?")) -> ()
            n143 = Destroy Stream Endpoint(11:w283) -> ()  [unwired: 1 in, 1 out]
            n144 = Destroy Stream Endpoint(11:w282) -> ()  [unwired: 1 in, 1 out]
            n145 = call "Close Variable Connections 9049.vi"("Variable References 9049"=w281) -> ()  [unwired: 11 in]
          }
        }
      }
      frame "Disconnect UI", "Disconnect UI 9039", "Disconnect UI 9049" {
        # "Disconnect UI - Something has gone wrong with the connection. Reinitialize the UI to its disconnected state."
        n146 = case shown="\"Disconnect UI 9049\"" w284 {
          tunnel: w288 -> [w290 w294 w299 w304]
          tunnel: [w290 w293 w298 w303] -> w287
          tunnel: w286 -> [_ w292 w297 w302]
          frame "False", Default {
          }
          frame "Disconnect UI" {
            w291 = FALSE ("Connected?")
            n147 = call "Enqueue Message.vi"("error in (no error)"=w294, "Message"="Disable Controls", "Message Queue"=w292) -> ("error out"=w293:errorcluster)  [unwired: 7 in, 1 out]
            n148 = local write "Connected 9039?"(w291) -> ()
            n149 = local write "Connected 9049?"(w291) -> ()
          }
          frame "Disconnect UI 9039" {
            n150 = call "Enqueue Message.vi"("error in (no error)"=w299, "Message"="Disable Controls 9039", "Message Queue"=w297) -> ("error out"=w298:errorcluster)  [unwired: 7 in, 1 out]
            n151 = local write "Connected 9039?"(FALSE ("Connected?")) -> ()
          }
          frame "Disconnect UI 9049" {
            n152 = local write "Connected 9049?"(FALSE ("Connected?")) -> ()
            n153 = call "Enqueue Message.vi"("error in (no error)"=w304, "Message"="Disable Controls 9049", "Message Queue"=w302) -> ("error out"=w303:errorcluster)  [unwired: 7 in, 1 out]
          }
        }
      }
      frame "Get Settings from FPGA" {
        # "Get Settings from FPGA - Send a command to the RT to retrieve all current FPGA Main VI parameter values and send them back to the UI."
        n154 = local read "Connected 9039?"() -> (w307:bool)
        n155 = case shown="True" w307 {
          tunnel: w309 -> [w311 w315]
          tunnel: [w311 w314] -> w308
          frame False {
            # "Don't bother trying to send a message to the RT system if UI Main VI isn't even connected"
          }
          frame True {
            n156 = global read "Global - UI Stream and Variable Connections.vi" "UI Command Stream"() -> (w312:refnum<k21>)
            n157 = shared-variable-write(w312, w315, T35 {"Message"="Send FPGA Configuration to UI", "Message Data"=variant} ("data in")) -> (w314:errorcluster)  [unwired: 1 in, 2 out]
          }
        }
      }
      frame "Initial UI Values" {
        # "Initial UI Values - These are the current values of the FPGA Main VI's R/W controls. They are used to initialize the panel of UI Main VI upon successful connection to the RT target."
        n158 = Variant To Data(error in=w331, type=T36 {"FPGA State"=enum."Safe State", "Manual Values"={"LNG_VCV_POS"=0, " LOX_VCV_POS"=0, "LNG_VCV_CLOSE"=FALSE, "LOX_VCV_CLOSE"=FALSE, "LNG_BV_OPEN"=FALSE, "LNG_BV_CLOSE"=FALSE, "LOX_BV_OPEN"=FALSE, "LOX_BV_CLOSE"=FALSE, "LNG_BFV_OPEN"=FALSE, "LNG_BFV_CLOSE"=FALSE, "LOX_BFV_OPEN"=FALSE, "LOX_BFV_CLOSE"=FALSE}, "Fill Valves"={"LOX_BV"=FALSE, "LNG_BV"=FALSE, "LNG_VCV_CTL"=0.0, "LOX_VCV_CTL"=0.0}, "LNG Purge System"={"LNG_USP"=FALSE, "LNG_DSP"=FALSE}, "LOX Purge System"={"LOX_USP"=FALSE, "LOX_DSP"=FALSE}, "DECOUPLERS"={"LNG_DC"=FALSE, "LOX_DC"=FALSE, "NGV_DC"=FALSE}, "VENT SYSTEM"={"LNG_BFV"=FALSE, "LOX_BFV"=FALSE, "NGV_GV"=FALSE}} ("All FPGA Configuration Values"), Variant=w329) -> (data=w327:T36, error out=w330:errorcluster)
        n159 = Unbundle By Name(w327) -> ("DECOUPLERS"=w320:T11, "Fill Valves"=w319:T38, "LNG Purge System"=w318:T10, "LOX Purge System"=w317:T6, "VENT SYSTEM"=w316:T9, "FPGA State"=w323:T37)
        n160 = local write "Current FPGA Control Mode"(w323) -> ()
        n161 = local write "VENT SYSTEM"(w316) -> ()
        n162 = local write "FILL VALVES"(w319) -> ()
        n163 = local write "DECOUPLERS"(w320) -> ()
        n164 = local write "LNG PURGE"(w318) -> ()
        n165 = local write "LOX PURGE"(w317) -> ()
        n166 = call "Enqueue Message.vi"("error in (no error)"=w330, "Message Data"=w323, "Message"="Update Display Mode", "Message Queue"=w322) -> ("error out"=w325:errorcluster)  [unwired: 6 in, 1 out]
      }
      frame "Run Control", "Run Manual", "Run Safe State", "Stop Control", "Stop Manual" {
        # "Run/Stop buttons - Send a command to switch the FPGA into the appropriate state. Send a message to update this UI to reflect the new state."
        n167 = local read "Connected 9039?"() -> (w333:bool)
        n168 = case shown="True" w333 {
          tunnel: w337 -> [w339 w349]
          tunnel: [w339 w345] -> w336
          tunnel: w335 -> [_ w344]
          tunnel: w334 -> [_ w343]
          frame False {
            # "Don't bother trying to send a message to the RT system if UI Main VI isn't even connected"
          }
          frame True {
            # "Run Manual and Run Control switch into their respective states. Anything else switches to Safe State."
            n169 = case shown="\"Run Control\"" w343 {
              tunnel: [FPGA_State."Safe State" ("FPGA State") FPGA_State."Control" ("FPGA State") FPGA_State."Manual" ("FPGA State")] -> w340
              frame "Safe State", "Stop Control", "Stop Manual", Default {
              }
              frame "Run Control" {
              }
              frame "Run Manual" {
              }
            }
            n170 = global read "Global - UI Stream and Variable Connections.vi" "UI Command Stream"() -> (w341:refnum<k21>)
            n171 = Bundle("Update FPGA State", "FPGA State"=w340) -> (w346:cluster{string, "FPGA State":T37})  [unwired: 1 in]
            n172 = shared-variable-write(w341, w349, w346) -> (w348:errorcluster)  [unwired: 1 in, 2 out]
            n173 = call "Enqueue Message.vi"("error in (no error)"=w348, "Message Data"=w340, "Message"="Update Display Mode", "Message Queue"=w344) -> ("error out"=w345:errorcluster)  [unwired: 6 in, 1 out]
          }
        }
      }
      frame "Safe Start" {
        # "Run/Stop buttons - Send a command to switch the FPGA into the appropriate state. Send a message to update this UI to reflect the new state."
        n174 = local read "Connected 9039?"() -> (w354:bool)
        n175 = case shown="True" w354 {
          tunnel: w358 -> [w360 w369]
          tunnel: [w360 w365] -> w357
          tunnel: w356 -> [_ w364]
          tunnel: w355 -> [_ _]
          frame False {
            # "Don't bother trying to send a message to the RT system if UI Main VI isn't even connected"
          }
          frame True {
            w361 = FPGA_State."Safe State" ("FPGA State")
            # "Run Manual and Run Control switch into their respective states. Anything else switches to Safe State."
            n176 = global read "Global - UI Stream and Variable Connections.vi" "UI Command Stream"() -> (w362:refnum<k21>)
            n177 = Bundle("Update FPGA State", "FPGA State"=w361) -> (w366:cluster{string, "FPGA State":T37})  [unwired: 1 in]
            n178 = shared-variable-write(w362, w369, w366) -> (w368:errorcluster)  [unwired: 1 in, 2 out]
            n179 = call "Enqueue Message.vi"("error in (no error)"=w368, "Message Data"=w361, "Message"="Update Display Mode Start", "Message Queue"=w364) -> ("error out"=w365:errorcluster)  [unwired: 6 in, 1 out]
          }
        }
      }
      frame "Update Manual Values", "Update Setpoints" {
        # "Update Manual Values/Setpoints - Send all manual values/setpoints to RT to be sent down to the FPGA."
        n180 = local read "Connected 9039?"() -> (w371:bool)
        n181 = case shown="True" w371 {
          tunnel: [w377 w383] -> w375
          tunnel: w374 -> [w377 w381]
          tunnel: w373 -> [_ w380]
          tunnel: w372 -> [_ w379]
          frame False {
            # "Don't bother trying to send a message to the RT system if UI Main VI isn't even connected"
          }
          frame True {
            n182 = global read "Global - UI Stream and Variable Connections.vi" "UI Command Stream"() -> (w378:refnum<k21>)
            n183 = Bundle(w380, "Message Data"=w379) -> (w382:cluster{string, "Message Data":variant})  [unwired: 1 in]
            n184 = shared-variable-write(w378, w381, w382) -> (w383:errorcluster)  [unwired: 1 in, 2 out]
          }
        }
      }
      frame "Record System" {
        # "Record Command for UI Monitoring"
        n185 = Variant To Data(type=TRUE, Variant=w387) -> (data=w385:bool)  [unwired: 1 in, 1 out]
        n186 = case shown="False" w385 {
          tunnel: w390 -> [w394 w399]
          tunnel: [w392 w398] -> w389
          tunnel: w388 -> [w393 w397]
          frame False {
            n187 = call "Enqueue Message.vi"("error in (no error)"=w393, "Message"="Stop", "Message Queue"=w394) -> ("error out"=w392:errorcluster)  [unwired: 7 in, 1 out]
          }
          frame True {
            n188 = call "Enqueue Message.vi"("error in (no error)"=w397, "Message"="Start", "Message Queue"=w399) -> ("error out"=w398:errorcluster)  [unwired: 7 in, 1 out]
          }
        }
      }
      frame "Set FIle Path" {
        # "Set file path for UI system monitoring log file"
        n189 = flat-sequence {
          tunnel: [w410] -> w403
          tunnel: w402 -> [w409]
          tunnel: [w408] -> w401
          tunnel: w406 -> [w422]
          tunnel: w405 -> [w421]
          tunnel: [w418] -> w404
          tunnel: w403 -> [w417]
          tunnel: w401 -> [w416]
          frame #0 {
            w411 = "*.tdms"  # pattern (all files)
            w413 = "Specify filepath to log TDMS data"  # prompt
            # "File Dialog:\nLimit selection to single item\nNew or Existing File"
            n190 = call <vilib>:"Application Directory.vi"() -> ("Application Directory"=w412:path)
            n191 = call "File Dialog2"("start path"=w412, "prompt"=w413, "error in"=w409, "pattern (all files)"=w411) -> ("selected path"=w408:path, "error out"=w410:errorcluster)  [unwired: 8 in, 2 out]
          }
          frame #1 {
            w414 = T44 {"Log File Base Path"=path "", "TDMS File Reference"=refnum, "Log File Path SYSTEM"=path "C:/Users/J.Schwartz/Documents/COMET LabVIEW/COMET Control and Acquisition VI/System Log Data/System Monitoring.tdms"} ("Logging Configuration")
            n192 = Bundle By Name(cluster=w414, "Log File Path SYSTEM"=w416) -> (w415:T44)
            n193 = Variant To Data(error in=w417, type=w414, Variant=w415) -> (data=w420:T44, error out=w419:errorcluster)
            n194 = call "Enqueue Message.vi"("error in (no error)"=w419, "Message Data"=w420, "Message"=w421, "Message Queue"=w422) -> ("error out"=w418:errorcluster)  [unwired: 6 in, 1 out]
          }
        }
      }
      frame "Force Trigger" {
        # "Update Manual Values/Setpoints - Send all manual values/setpoints to RT to be sent down to the FPGA."
        n195 = local read "Connected 9049?"() -> (w426:bool)
        n196 = local read "Connected 9039?"() -> (w431:bool)
        n197 = case shown="True" w431 {
          tunnel: [w440 w446] -> w428
          tunnel: w423 -> [w440 w444]
          tunnel: w425 -> [_ w443]
          tunnel: w424 -> [_ w442]
          frame False {
            # "Don't bother trying to send a message to the RT system if UI Main VI isn't even connected"
          }
          frame True {
            n198 = global read "Global - UI Stream and Variable Connections.vi" "UI Command Stream"() -> (w441:refnum<k21>)
            n199 = Bundle(w443, "Message Data"=w442) -> (w445:cluster{string, "Message Data":variant})  [unwired: 1 in]
            n200 = shared-variable-write(w441, w444, w445) -> (w446:errorcluster)  [unwired: 1 in, 2 out]
          }
        }
        n201 = case shown="True" w426 {
          tunnel: [w433 w439] -> w429
          tunnel: w423 -> [w433 w437]
          tunnel: w425 -> [_ w436]
          tunnel: w424 -> [_ w435]
          frame False {
            # "Don't bother trying to send a message to the RT system if UI Main VI isn't even connected"
          }
          frame True {
            n202 = global read "Global - UI Stream and Variable Connections.vi" "UI Command Stream 9049"() -> (w434:refnum<k21>)
            n203 = Bundle(w436, "Message Data"=w435) -> (w438:cluster{string, "Message Data":variant})  [unwired: 1 in]
            n204 = shared-variable-write(w434, w437, w438) -> (w439:errorcluster)  [unwired: 1 in, 2 out]
          }
        }
        n205 = Merge Errors(w429, w428) -> (w427:errorcluster)
      }
      frame "Acquire Live Data 9222 9039", "Acquire Live Data 9237 9039", "Get Logging Status 9039", "Live Channel Change 9222", "Live Channel Change 9237", "Stop Live Data 9039", "Time Domain" {
        # "Update Manual Values/Setpoints - Send all manual values/setpoints to RT to be sent down to the FPGA."
        n206 = local read "Connected 9039?"() -> (w449:bool)
        n207 = case shown="True" w449 {
          tunnel: w452 -> [w454 w463]
          tunnel: [w454 w462] -> w447
          tunnel: w451 -> [_ w457]
          tunnel: w450 -> [_ w455]
          tunnel: w448 -> [_ w456]
          frame False {
            # "Don't bother trying to send a message to the RT system if UI Main VI isn't even connected"
          }
          frame True {
            # "For live data commands, enable/disable buttons on UI appropriately."
            n208 = Bundle By Name(cluster=T39 {"Message"="", "Message Data"=variant} ("Message Cluster"), "Message"=w455, "Message Data"=w457) -> (w458:T39)
            n209 = case shown="Default" w455 {
              tunnel: w456 -> [_ w470 w477 w483]
              frame Default {
              }
              frame "Acquire Live Data 9237 9039" {
                n210 = Unbundle By Name(w470) -> ("Acquire Live Data 9237 9039"=w469:refnum<vi>, "Stop Live Data 9039"=w468:refnum<vi>, "Acquire Live Data 9222 9039"=w465:refnum<vi>)
                n211 = property class="Bool"(reference=w469, "DisabledEnum"=u8 2) -> ()  [unwired: 1 in, 2 out]
                n212 = property class="Bool"(reference=w468, "DisabledEnum"=u8 0) -> ()  [unwired: 1 in, 2 out]
                n213 = property class="Bool"(reference=w465, "DisabledEnum"=u8 2) -> ()  [unwired: 1 in, 2 out]
              }
              frame "Acquire Live Data 9222 9039" {
                n214 = Unbundle By Name(w477) -> ("Acquire Live Data 9222 9039"=w476:refnum<vi>, "Stop Live Data 9039"=w475:refnum<vi>, "Acquire Live Data 9237 9039"=w471:refnum<vi>)
                n215 = property class="Bool"(reference=w471, "DisabledEnum"=u8 2) -> ()  [unwired: 1 in, 2 out]
                n216 = property class="Bool"(reference=w476, "DisabledEnum"=u8 2) -> ()  [unwired: 1 in, 2 out]
                n217 = property class="Bool"(reference=w475, "DisabledEnum"=u8 0) -> ()  [unwired: 1 in, 2 out]
              }
              frame "Stop Live Data 9039" {
                w478 = u8 0
                n218 = Unbundle By Name(w483) -> ("Acquire Live Data 9237 9039"=w482:refnum<vi>, "Stop Live Data 9039"=w481:refnum<vi>, "Acquire Live Data 9222 9039"=w479:refnum<vi>)
                n219 = property class="Bool"(reference=w482, "DisabledEnum"=w478) -> ()  [unwired: 1 in, 2 out]
                n220 = property class="Bool"(reference=w481, "DisabledEnum"=u8 2) -> ()  [unwired: 1 in, 2 out]
                n221 = property class="Bool"(reference=w479, "DisabledEnum"=w478) -> ()  [unwired: 1 in, 2 out]
              }
            }
            n222 = global read "Global - Configuration Options WVFM.vi" "Network Stream Polling Timeout (ms)"() -> (w460:i32)
            n223 = global read "Global - UI Stream and Variable Connections.vi" "UI Command Stream"() -> (w461:refnum<k21>)
            n224 = shared-variable-write(w461, w463, w458, w460) -> (w462:errorcluster)  [unwired: 2 out]
          }
        }
      }
      frame "Acquire Live Data 9222 9049", "Acquire Live Data 9237 9049", "Get Logging Status 9049", "Live Channel Change 9222 9049", "Live Channel Change 9237 9049", "Stop Live Data 9049" {
        # "Update Manual Values/Setpoints - Send all manual values/setpoints to RT to be sent down to the FPGA."
        n225 = local read "Connected 9049?"() -> (w486:bool)
        n226 = case shown="True" w486 {
          tunnel: w489 -> [w491 w500]
          tunnel: [w491 w499] -> w484
          tunnel: w488 -> [_ w494]
          tunnel: w487 -> [_ w492]
          tunnel: w485 -> [_ w493]
          frame False {
            # "Don't bother trying to send a message to the RT system if UI Main VI isn't even connected"
          }
          frame True {
            # "For live data commands, enable/disable buttons on UI appropriately."
            n227 = Bundle By Name(cluster=T39 {"Message"="", "Message Data"=variant} ("Message Cluster"), "Message"=w492, "Message Data"=w494) -> (w495:T39)
            n228 = case shown="\"Stop Live Data 9049\"" w492 {
              tunnel: w493 -> [_ w507 w514 w520]
              frame Default {
              }
              frame "Acquire Live Data 9237 9049" {
                n229 = Unbundle By Name(w507) -> ("Acquire Live Data 9237 9049"=w506:refnum<vi>, "Stop Live Data 9049"=w505:refnum<vi>, "Acquire Live Data 9222 9049"=w502:refnum<vi>)
                n230 = property class="Bool"(reference=w506, "DisabledEnum"=u8 2) -> ()  [unwired: 1 in, 2 out]
                n231 = property class="Bool"(reference=w505, "DisabledEnum"=u8 0) -> ()  [unwired: 1 in, 2 out]
                n232 = property class="Bool"(reference=w502, "DisabledEnum"=u8 2) -> ()  [unwired: 1 in, 2 out]
              }
              frame "Acquire Live Data 9222 9049" {
                n233 = Unbundle By Name(w514) -> ("Acquire Live Data 9222 9049"=w513:refnum<vi>, "Stop Live Data 9049"=w512:refnum<vi>, "Acquire Live Data 9237 9049"=w508:refnum<vi>)
                n234 = property class="Bool"(reference=w508, "DisabledEnum"=u8 2) -> ()  [unwired: 1 in, 2 out]
                n235 = property class="Bool"(reference=w513, "DisabledEnum"=u8 2) -> ()  [unwired: 1 in, 2 out]
                n236 = property class="Bool"(reference=w512, "DisabledEnum"=u8 0) -> ()  [unwired: 1 in, 2 out]
              }
              frame "Stop Live Data 9049" {
                w515 = u8 0
                n237 = Unbundle By Name(w520) -> ("Acquire Live Data 9237 9049"=w519:refnum<vi>, "Stop Live Data 9049"=w518:refnum<vi>, "Acquire Live Data 9222 9049"=w516:refnum<vi>)
                n238 = property class="Bool"(reference=w519, "DisabledEnum"=w515) -> ()  [unwired: 1 in, 2 out]
                n239 = property class="Bool"(reference=w518, "DisabledEnum"=u8 2) -> ()  [unwired: 1 in, 2 out]
                n240 = property class="Bool"(reference=w516, "DisabledEnum"=w515) -> ()  [unwired: 1 in, 2 out]
              }
            }
            n241 = global read "Global - Configuration Options WVFM.vi" "Network Stream Polling Timeout (ms)"() -> (w497:i32)
            n242 = global read "Global - UI Stream and Variable Connections.vi" "UI Command Stream 9049"() -> (w498:refnum<k21>)
            n243 = shared-variable-write(w498, w500, w495, w497) -> (w499:errorcluster)  [unwired: 2 out]
          }
        }
      }
      frame "Abort", "Arm", "Update LNG Purge System", "Update LOX Purge System", "Update NG_PVC_BV", "Update Recirc System", "Update Vent System" {
        # "Update Manual Values/Setpoints - Send all manual values/setpoints to RT to be sent down to the FPGA."
        n244 = local read "Connected 9039?"() -> (w523:bool)
        n245 = case shown="True" w523 {
          tunnel: [w528 w534] -> w527
          tunnel: w526 -> [w528 w532]
          tunnel: w525 -> [_ w531]
          tunnel: w524 -> [_ w530]
          frame False {
            # "Don't bother trying to send a message to the RT system if UI Main VI isn't even connected"
          }
          frame True {
            n246 = global read "Global - UI Stream and Variable Connections.vi" "UI Command Stream"() -> (w529:refnum<k21>)
            n247 = Bundle(w531, "Message Data"=w530) -> (w533:cluster{string, "Message Data":variant})  [unwired: 1 in]
            n248 = shared-variable-write(w529, w532, w533) -> (w534:errorcluster)  [unwired: 1 in, 2 out]
          }
        }
      }
      frame "Update Fill Valves" {
        w553 = 0
        w554 = 2
        # "Update Manual Values/Setpoints - Send all manual values/setpoints to RT to be sent down to the FPGA."
        n249 = Variant To Data(type=T12 {"LOX_BV"=FALSE, "LNG_BV"=FALSE, "LNG_VCV_CTL"=32.0, "LOX_VCV_CTL"=25.0} ("FILL VALVES"), Variant=w558) -> (data=w552:T12)  [unwired: 1 in, 1 out]
        n250 = local read "Connected 9039?"() -> (w560:bool)
        n251 = Unbundle By Name(w552) -> ("LOX_VCV_CTL"=w550:sgl, "LOX_BV"=w536:bool, "LNG_BV"=w535:bool, "LNG_VCV_CTL"=w542:sgl)
        n252 = case shown="False" FALSE {
          tunnel: w538 -> [_ w570]
          tunnel: w536 -> [_ w565]
          tunnel: w535 -> [_ w564]
          frame False {
          }
          frame True {
            n253 = Unbundle By Name(w570) -> ("LOX_VCV"=w569:refnum<vi>, "LNG_VCV"=w567:refnum<vi>)
            n254 = Build Array(w567) -> (w566:refnum<vi>[])
            n255 = Build Array(w569) -> (w568:refnum<vi>[])
            n256 = call "Set Enable State on Multiple Controls.vi"("Enable?"=w564, "Controls"=w566) -> ()  [unwired: 10 in]
            n257 = call "Set Enable State on Multiple Controls.vi"("Enable?"=w565, "Controls"=w568) -> ()  [unwired: 10 in]
          }
        }
        n258 = Multiply(x=sgl 0.00016, y=w550) -> (x*y=w548:sgl)
        n259 = Select(t=w553, s=w536, f=w554) -> (s? t:f=w556:i32)
        n260 = Select(t=w553, s=w535, f=w554) -> (s? t:f=w555:i32)
        n261 = Multiply(x=sgl 0.00016, y=w542) -> (x*y=w544:sgl)
        n262 = Add(x=sgl 0.004 ("LNG_VCV_CTL"), y=w548) -> (x+y=w546:sgl)
        n263 = property on="LOX_VCV_CTL" class="Slide (strict)"("DisabledEnum"=w556) -> ()  [unwired: 2 in, 2 out]
        n264 = property on="LNG_VCV_CTL" class="Slide (strict)"("DisabledEnum"=w555) -> ()  [unwired: 2 in, 2 out]
        n265 = Add(x=sgl 0.004 ("LNG_VCV_CTL"), y=w544) -> (x+y=w541:sgl)
        n266 = Bundle By Name(cluster=T38 {"LOX_BV"=FALSE, "LNG_BV"=FALSE, "LNG_VCV_CTL"=0.0, "LOX_VCV_CTL"=0.0} ("Fill Valves"), "LOX_VCV_CTL"=w546, "LOX_BV"=w536, "LNG_BV"=w535, "LNG_VCV_CTL"=w541) -> (w540:T38)
        n267 = To Variant(anything=w540) -> (Variant=w539:variant)
        n268 = case shown="True" w560 {
          tunnel: [w571 w577] -> w563
          tunnel: w562 -> [w571 w575]
          tunnel: w561 -> [_ w574]
          tunnel: w539 -> [_ w573]
          frame False {
            # "Don't bother trying to send a message to the RT system if UI Main VI isn't even connected"
          }
          frame True {
            n269 = global read "Global - UI Stream and Variable Connections.vi" "UI Command Stream"() -> (w572:refnum<k21>)
            n270 = Bundle(w574, "Variant"=w573) -> (w576:cluster{string, "Variant":variant})  [unwired: 1 in]
            n271 = shared-variable-write(w572, w575, w576) -> (w577:errorcluster)  [unwired: 1 in, 2 out]
          }
        }
      }
      frame "Update Tank Pressure" {
        # "Update Manual Values/Setpoints - Send all manual values/setpoints to RT to be sent down to the FPGA."
        n272 = case shown="False" FALSE {
          tunnel: w583 -> [_ w600]
          frame False {
          }
          frame True {
            n273 = Unbundle By Name(w600) -> ("Pressure PID"=w599:refnum<vi>)
            n274 = Build Array(w599) -> (w598:refnum<vi>[])
            n275 = call "Set Enable State on Multiple Controls.vi"("Enable?"=TRUE, "Controls"=w598) -> ()  [unwired: 10 in]
          }
        }
        n276 = Variant To Data(type=T40 {"Setpoint"=0.0, "proportional gain (Kc)"=0.0, "integral time (Ti, min)"=0.0, "derivative time (Td, min)"=0.0, "output high"=0.0, "output low"=0.0} ("input cluster"), Variant=w585) -> (data=w580:T40)  [unwired: 1 in, 1 out]
        n277 = local read "Connected 9039?"() -> (w587:bool)
        n278 = local read "Pressure\nControl"() -> (w581:bool)
        n279 = case shown="True" w581 {
          tunnel: w580 -> [_ w596]
          tunnel: [w592 w596] -> w578
          frame False {
            w591 = 0.0
            n280 = Bundle(0.0, 0.0, 0.0, w591, w591, w591) -> (w592:cluster{dbl, dbl, dbl, dbl, dbl, dbl})  [unwired: 1 in]
          }
          frame True {
          }
        }
        n281 = shared-variable "NI-cRIO-9039-01AA2F3E\\Shared Variables.lvlib\\PID Control"(w578) -> ()  [unwired: 1 in, 1 out]
        n282 = To Variant(anything=w578) -> (Variant=w584:variant)
        n283 = case shown="True" w587 {
          tunnel: [w601 w607] -> w590
          tunnel: w589 -> [w601 w605]
          tunnel: w588 -> [_ w604]
          tunnel: w584 -> [_ w603]
          frame False {
            # "Don't bother trying to send a message to the RT system if UI Main VI isn't even connected"
          }
          frame True {
            n284 = global read "Global - UI Stream and Variable Connections.vi" "UI Command Stream"() -> (w602:refnum<k21>)
            n285 = Bundle(w604, "Variant"=w603) -> (w606:cluster{string, "Variant":variant})  [unwired: 1 in]
            n286 = shared-variable-write(w602, w605, w606) -> (w607:errorcluster)  [unwired: 1 in, 2 out]
          }
        }
      }
      frame "Expansion Chassis" {
        # "Update Manual Values/Setpoints - Send all manual values/setpoints to RT to be sent down to the FPGA."
        n287 = case shown="False" FALSE {
          tunnel: w611 -> [_ w622]
          frame False {
          }
          frame True {
            n288 = Unbundle By Name(w622) -> ("Pressure PID"=w621:refnum<vi>)
            n289 = Build Array(w621) -> (w620:refnum<vi>[])
            n290 = call "Set Enable State on Multiple Controls.vi"("Enable?"=TRUE, "Controls"=w620) -> ()  [unwired: 10 in]
          }
        }
        n291 = local read "Expansion Chassis?"() -> (w609:bool)
        n292 = Variant To Data(type=w609, Variant=w613) -> (data=w608:bool)  [unwired: 1 in, 1 out]
        n293 = local read "Connected 9039?"() -> (w615:bool)
        n294 = To Variant(anything=w608) -> (Variant=w612:variant)
        n295 = case shown="True" w615 {
          tunnel: [w623 w629] -> w618
          tunnel: w617 -> [w623 w627]
          tunnel: w616 -> [_ w626]
          tunnel: w612 -> [_ w625]
          frame False {
            # "Don't bother trying to send a message to the RT system if UI Main VI isn't even connected"
          }
          frame True {
            n296 = global read "Global - UI Stream and Variable Connections.vi" "UI Command Stream"() -> (w624:refnum<k21>)
            n297 = Bundle(w626, "Variant"=w625) -> (w628:cluster{string, "Variant":variant})  [unwired: 1 in]
            n298 = shared-variable-write(w624, w627, w628) -> (w629:errorcluster)  [unwired: 1 in, 2 out]
          }
        }
      }
      frame "Enable Tank Pressure" {
        # "Update Manual Values/Setpoints - Send all manual values/setpoints to RT to be sent down to the FPGA."
        n299 = case shown="True" FALSE {
          tunnel: w643 -> [_ w655]
          frame False {
          }
          frame True {
            n300 = Unbundle By Name(w655) -> ("Pressure PID"=w654:refnum<vi>)
            n301 = Build Array(w654) -> (w653:refnum<vi>[])
            n302 = call "Set Enable State on Multiple Controls.vi"("Enable?"=TRUE, "Controls"=w653) -> ()  [unwired: 10 in]
          }
        }
        n303 = property on="Pessure PID" class="Clust (strict)"("DisabledEnum"=T41."Enabled" ("Disabled")) -> ()  [unwired: 2 in, 2 out]
        n304 = local read "Connected 9039?"() -> (w641:bool)
        n305 = Bundle By Name(cluster=T20 {"Set Point [psi]"=0.0, "Proportional (K)"=0.0, "Integral (I)"=0.0, "Derivative (D)"=0.0} ("Pessure PID"), "Set Point [psi]"=0.0, "Proportional (K)"=0.0, "Integral (I)"=0.0, "Derivative (D)"=0.0) -> (w632:T20)
        n306 = To Variant(anything=w632) -> (Variant=w631:variant)
        n307 = case shown="True" w641 {
          tunnel: w640 -> [w645 w648]
          tunnel: [w645 w647] -> w639
          tunnel: w638 -> [_ w651]
          tunnel: w631 -> [_ w650]
          frame False {
          }
          frame True {
            n308 = global read "Global - UI Stream and Variable Connections.vi" "UI Command Stream"() -> (w646:refnum<k21>)
            n309 = Bundle(w651, "Variant"=w650) -> (w649:cluster{string, "Variant":variant})  [unwired: 1 in]
            n310 = shared-variable-write(w646, w648, w649) -> (w647:errorcluster)  [unwired: 1 in, 2 out]
          }
        }
      }
      frame "Start Auto P&D" {
        # "Update Manual Values/Setpoints - Send all manual values/setpoints to RT ."
        n311 = Unbundle By Name(w663) -> ("Fill Valves"=w662:refnum<vi>, "VENT SYSTEM"=w661:refnum<vi>, "LNG Purge System"=w660:refnum<vi>, "LNG Purge System"=w659:refnum<vi>, "DECOUPLERS"=w658:refnum<vi>)
        n312 = local read "Connected 9039?"() -> (w665:bool)
        n313 = case shown="True" w665 {
          tunnel: [w670 w676] -> w669
          tunnel: w668 -> [w670 w674]
          tunnel: w667 -> [_ w673]
          tunnel: w666 -> [_ w672]
          frame False {
            # "Don't bother trying to send a message to the RT system if UI Main VI isn't even connected"
          }
          frame True {
            n314 = global read "Global - UI Stream and Variable Connections.vi" "UI Command Stream"() -> (w671:refnum<k21>)
            n315 = Bundle(w673, "Message Data"=w672) -> (w675:cluster{string, "Message Data":variant})  [unwired: 1 in]
            n316 = shared-variable-write(w671, w674, w675) -> (w676:errorcluster)  [unwired: 1 in, 2 out]
          }
        }
        n317 = Build Array(w662, w661, w660, w659, w658) -> (w657:refnum<vi>[])
        n318 = call "Set Enable State on Multiple Controls.vi"("Enable?"=FALSE, "Controls"=w657) -> ()  [unwired: 10 in]
      }
      frame "Auto Disconnect LNG", "Auto Disconnect LOX", "Auto Disconnect NGV", "Disconnect LNG", "Disconnect LOX", "Disconnect NGV" {
        # "Update Manual Values/Setpoints - Send all manual values/setpoints to RT to be sent down to the FPGA."
        n319 = local read "Connected 9039?"() -> (w679:bool)
        n320 = case shown="True" w679 {
          tunnel: [w684 w690] -> w683
          tunnel: w682 -> [w684 w688]
          tunnel: w681 -> [_ w687]
          tunnel: w680 -> [_ w686]
          frame False {
            # "Don't bother trying to send a message to the RT system if UI Main VI isn't even connected"
          }
          frame True {
            n321 = global read "Global - UI Stream and Variable Connections.vi" "UI Command Stream"() -> (w685:refnum<k21>)
            n322 = Bundle(w687, "Message Data"=w686) -> (w689:cluster{string, "Message Data":variant})  [unwired: 1 in]
            n323 = shared-variable-write(w685, w688, w689) -> (w690:errorcluster)  [unwired: 1 in, 2 out]
          }
        }
      }
      frame "LNG Partial Purge", "LOX Partial Purge", "Upstream Purge" {
        # "Update Manual Values/Setpoints - Send all manual values/setpoints to RT to be sent down to the FPGA."
        n324 = local read "Connected 9039?"() -> (w693:bool)
        n325 = case shown="True" w693 {
          tunnel: [w698 w704] -> w697
          tunnel: w696 -> [w698 w702]
          tunnel: w695 -> [_ w701]
          tunnel: w694 -> [_ w700]
          frame False {
            # "Don't bother trying to send a message to the RT system if UI Main VI isn't even connected"
          }
          frame True {
            n326 = global read "Global - UI Stream and Variable Connections.vi" "UI Command Stream"() -> (w699:refnum<k21>)
            n327 = Bundle(w701, "Message Data"=w700) -> (w703:cluster{string, "Message Data":variant})  [unwired: 1 in]
            n328 = shared-variable-write(w699, w702, w703) -> (w704:errorcluster)  [unwired: 1 in, 2 out]
          }
        }
      }
      frame "Send Logging Status 9222 9039", "Send Logging Status 9222 9049", "Send Logging Status 9237 9039", "Send Logging Status 9237 9049" {
        # "TRUE: Logging Normally\nFALSE: Idle (Safe State)"
        n329 = Variant To Data(error in=w709, type=FALSE, Variant=w708) -> (data=w707:bool)  [unwired: 1 out]
        n330 = case shown="\"Send Logging Status 9222 9039\", \"Send Logging Status 9237 9039\"" w705 {
          tunnel: w707 -> [_ w715 w727]
          tunnel: w706 -> [_ w714 w726]
          frame "False", Default {
          }
          frame "Send Logging Status 9222 9039", "Send Logging Status 9237 9039" {
            n331 = Unbundle By Name(w714) -> ("Acquire Live Data 9237 9039"=w718:refnum<vi>, "Force Trigger"=w719:refnum<vi>, "Stop Live Data 9039"=w722:refnum<vi>, "Acquire Live Data 9222 9039"=w713:refnum<vi>)
            n332 = Build Array(w718, w719, w713) -> (w720:refnum<vi>[])
            n333 = Build Array(w722) -> (w721:refnum<vi>[])
            n334 = call "Set Enable State on Multiple Controls.vi"("Enable?"=w715, "Controls"=w720) -> ()  [unwired: 10 in]
            n335 = call "Set Enable State on Multiple Controls.vi"("Enable?"=FALSE, "Controls"=w721) -> ()  [unwired: 10 in]
            n336 = Select(t=u16 0, s=w715, f=u16 1) -> (s? t:f=→"Current Logging State 9039":u16)
          }
          frame "Send Logging Status 9222 9049", "Send Logging Status 9237 9049" {
            n337 = Unbundle By Name(w726) -> ("Acquire Live Data 9237 9049"=w730:refnum<vi>, "Force Trigger"=w731:refnum<vi>, "Stop Live Data 9049"=w734:refnum<vi>, "Acquire Live Data 9222 9049"=w725:refnum<vi>)
            n338 = Build Array(w730, w731, w725) -> (w732:refnum<vi>[])
            n339 = Build Array(w734) -> (w733:refnum<vi>[])
            n340 = call "Set Enable State on Multiple Controls.vi"("Enable?"=w727, "Controls"=w732) -> ()  [unwired: 10 in]
            n341 = call "Set Enable State on Multiple Controls.vi"("Enable?"=FALSE, "Controls"=w733) -> ()  [unwired: 10 in]
            n342 = Select(t=u16 0, s=w727, f=u16 1) -> (s? t:f=→"Current Logging State 9049":u16)
          }
        }
      }
      frame "Send Path to UI 9222 9039", "Send Path to UI 9222 9049", "Send Path to UI 9237 9039", "Send Path to UI 9237 9049" {
        n343 = Variant To Data(error in=w741, type=path "", Variant=w740) -> (data=w737:path)  [unwired: 1 out]
        n344 = case shown="\"Send Path to UI 9237 9049\"" w736 {
          tunnel: w737 -> [_ w743 w744 w745 w746]
          frame Default {
          }
          frame "Send Path to UI 9237 9039" {
            "Most recent manually-triggered log file 9237" <- w743
          }
          frame "Send Path to UI 9222 9039" {
            "Most recent manually-triggered log file 9222" <- w744
          }
          frame "Send Path to UI 9222 9049" {
            "Most recent manually-triggered log file 9222 9049" <- w745
          }
          frame "Send Path to UI 9237 9049" {
            "Most recent manually-triggered log file 9237 9049" <- w746
          }
        }
      }
      frame "Send Live Data to UI 9222 9039", "Send Live Data to UI 9222 9049", "Send Live Data to UI 9237 9039", "Send Live Data to UI 9237 9049" {
        n345 = case shown="\"Send Live Data to UI 9222 9049\"" w747 {
          tunnel: w750 -> [_ w755 w759 w763 w767]
          tunnel: w749 -> [_ w754 w758 w762 w766]
          frame "False", Default {
          }
          frame "Send Live Data to UI 9237 9039" {
            n346 = Variant To Data(error in=w755, type=waveform(dbl) {"t0"=timestamp(0 s since 1904-01-01), "dt"=1.0, "Y"=[]}, Variant=w754) -> (data=→"9237 Live Data 9039":waveform(dbl))  [unwired: 1 out]
          }
          frame "Send Live Data to UI 9237 9049" {
            n347 = Variant To Data(error in=w759, type=waveform(dbl) {"t0"=timestamp(0 s since 1904-01-01), "dt"=1.0, "Y"=[]}, Variant=w758) -> (data=→"9237 Live Data 9049":waveform(dbl))  [unwired: 1 out]
          }
          frame "Send Live Data to UI 9222 9039" {
            n348 = Variant To Data(error in=w763, type=waveform(dbl) {"t0"=timestamp(0 s since 1904-01-01), "dt"=1.0, "Y"=[]}, Variant=w762) -> (data=→"9222 Live Data 9039":waveform(dbl))  [unwired: 1 out]
          }
          frame "Send Live Data to UI 9222 9049" {
            n349 = Variant To Data(error in=w767, type=waveform(dbl) {"t0"=timestamp(0 s since 1904-01-01), "dt"=1.0, "Y"=[]}, Variant=w766) -> (data=→"9222 Live Data 9049":waveform(dbl))  [unwired: 1 out]
          }
        }
      }
      frame "9049" {
      }
      frame "Update Display Mode" {
        # "Update Display Mode - Enable/Disable Controls appropriately for the new display mode."
        n350 = control-ref of="LOX_DC"() -> (w780:refnum<vi>)
        n351 = Variant To Data(error in=w799, type=FPGA_State."Safe State" ("FPGA State"), Variant=w797) -> (data=w796:T37, error out=w798:errorcluster)
        n352 = Unbundle By Name(w778) -> ("Switch to Safe State Ref"=w795:refnum<vi>, "Run Manual Ref"=w794:refnum<vi>, "Stop Manual Ref"=w793:refnum<vi>, "Run Control Ref"=w792:refnum<vi>, "Stop Control Ref"=w791:refnum<vi>, "LNG_BV"=w788:refnum<vi>, "LOX_BV"=w787:refnum<vi>, "LOX DC"=w786:refnum<vi>, "LNG DC"=w785:refnum<vi>, "Record Button"=w784:refnum<vi>, "NGV DC"=w783:refnum<vi>, "LNG BFV"=w782:refnum<vi>, "LOX Purge System"=w777:refnum<vi>, "Fill Valves"=w781:refnum<vi>, "LNG Purge System"=w776:refnum<vi>, "VENT SYSTEM"=w779:refnum<vi>, "DECOUPLERS"=w775:refnum<vi>, "NGV N2"=w772:refnum<vi>, "Turn on Pressure Control"=w771:refnum<vi>)
        n353 = control-ref of="MANUAL PURGE"() -> (w774:refnum<vi>)
        n354 = control-ref of="ABORT DCs"() -> (w773:refnum<vi>)
        n355 = case shown="\"Safe State\"" w796 {
          tunnel: w795 -> [w817 w826 w851]
          tunnel: w794 -> [w813 w825 w853]
          tunnel: w793 -> [w816 w824 w850]
          tunnel: w792 -> [w815 w822 w852]
          tunnel: w791 -> [w814 w823 w849]
          tunnel: w788 -> [w808 _ w848]
          tunnel: w787 -> [w812 _ w847]
          tunnel: w786 -> [w811 _ w846]
          tunnel: w785 -> [w807 _ w845]
          tunnel: w784 -> [w810 _ w844]
          tunnel: w783 -> [w809 _ w843]
          tunnel: w782 -> [w806 _ w842]
          tunnel: w781 -> [w805 _ w841]
          tunnel: w780 -> [w804 _ w839]
          tunnel: w779 -> [w803 _ w840]
          tunnel: w777 -> [_ _ w838]
          tunnel: w776 -> [_ _ w837]
          tunnel: w775 -> [_ _ w836]
          tunnel: w774 -> [w802 _ w834]
          tunnel: w773 -> [w801 _ w835]
          tunnel: w772 -> [_ _ w833]
          tunnel: w771 -> [w800 _ w831]
          frame "Control" {
            n356 = Build Array "Controls to Enable"(w817, w814, w813, w812, w811, w810, w809, w808, w807, w806, w805, w804, w803, w802, w801, w800) -> (w821:refnum<vi>[])
            n357 = Build Array "Controls to Disable"(w816, w815) -> (w819:refnum<vi>[])
            n358 = call "Set Enable State on Multiple Controls.vi"("Enable?"=TRUE, "Controls"=w821) -> ()  [unwired: 10 in]
            n359 = call "Set Enable State on Multiple Controls.vi"("Enable?"=FALSE, "Controls"=w819) -> ()  [unwired: 10 in]
          }
          frame "Manual" {
            n360 = Build Array "Controls to Enable"(w826, w824, w822) -> (w830:refnum<vi>[])
            n361 = Build Array "Controls to Disable"(w825, w823) -> (w828:refnum<vi>[])
            n362 = call "Set Enable State on Multiple Controls.vi"("Enable?"=FALSE, "Controls"=w828) -> ()  [unwired: 10 in]
            n363 = call "Set Enable State on Multiple Controls.vi"("Enable?"=TRUE, "Controls"=w830) -> ()  [unwired: 10 in]
          }
          frame "Safe State" {
            # "This frame runs when FPGA is in Safe State. Only enable the two run buttons."
            n364 = Build Array "Controls to Enable"(w853, w852) -> (w857:refnum<vi>[])
            n365 = Build Array "Controls to Disable"(w851, w850, w849, w848, w847, w846, w845, w844, w843, w842, w838, w841, w840, w837, w836, w839, w834, w835, w833, w831) -> (w855:refnum<vi>[])
            n366 = property on="MANUAL PURGE" class="Bool (strict)"("Value"=FALSE ("MANUAL PURGE")) -> ()  [unwired: 2 in, 2 out]
            n367 = call "Set Enable State on Multiple Controls.vi"("Enable?"=FALSE, "Controls"=w855) -> ()  [unwired: 10 in]
            n368 = call "Set Enable State on Multiple Controls.vi"("Enable?"=TRUE, "Controls"=w857) -> ()  [unwired: 10 in]
          }
        }
      }
      frame "MANUAL PURGE" {
        # "Update Display Mode - Enable/Disable Controls appropriately for the new display mode."
        n369 = Variant To Data(error in=w863, type=TRUE, Variant=w861) -> (data=w859:bool, error out=w862:errorcluster)
        n370 = case shown="False" w859 {
          tunnel: w858 -> [w867 w875]
          frame False {
            n371 = Unbundle By Name(w867) -> ("LNG Purge System"=w870:refnum<vi>, "LOX Purge System"=w871:refnum<vi>, "DECOUPLERS"=w872:refnum<vi>, "NGV N2"=w866:refnum<vi>)
            n372 = Build Array "Controls to Enable"(w870, w871, w872, w866) -> (w869:refnum<vi>[])
            n373 = call "Set Enable State on Multiple Controls.vi"("Enable?"=FALSE, "Controls"=w869) -> ()  [unwired: 10 in]
          }
          frame True {
            n374 = Unbundle By Name(w875) -> ("LNG Purge System"=w877:refnum<vi>, "LOX Purge System"=w878:refnum<vi>, "DECOUPLERS"=w879:refnum<vi>, "NGV N2"=w873:refnum<vi>)
            n375 = Build Array "Controls to Enable"(w877, w878, w879, w873) -> (w876:refnum<vi>[])
            n376 = call "Set Enable State on Multiple Controls.vi"("Enable?"=TRUE, "Controls"=w876) -> ()  [unwired: 10 in]
          }
        }
      }
      frame "Update Display Mode Start" {
        # "This frame runs when FPGA is in Safe State. Only enable the two run buttons."
        # "Update Display Mode - Enable/Disable Controls appropriately for the new display mode."
        n377 = Unbundle By Name(w915) -> ("Switch to Safe State Ref"=w908:refnum<vi>, "Run Manual Ref"=w907:refnum<vi>, "Stop Manual Ref"=w906:refnum<vi>, "Run Control Ref"=w905:refnum<vi>, "Stop Control Ref"=w904:refnum<vi>, "LNG_BV"=w903:refnum<vi>, "LOX_BV"=w902:refnum<vi>, "LOX DC"=w901:refnum<vi>, "LNG DC"=w900:refnum<vi>, "Record Button"=w899:refnum<vi>, "NGV DC"=w898:refnum<vi>, "LNG BFV"=w897:refnum<vi>, "LOX BFV"=w896:refnum<vi>, "Fill Valves"=w895:refnum<vi>, "VENT SYSTEM"=w894:refnum<vi>, "DECOUPLERS"=w893:refnum<vi>, "LNG Purge System"=w892:refnum<vi>, "Turn on Pressure Control"=w881:refnum<vi>, "Pressure PID"=w880:refnum<vi>)
        n378 = control-ref of="Stop Live Data 9039"() -> (w886:refnum<vi>)
        n379 = Variant To Data(error in=w917, type=FPGA_State."Safe State" ("FPGA State"), Variant=w916) -> (error out=w912:errorcluster)  [unwired: 1 out]
        n380 = control-ref of="Force Trigger"() -> (w887:refnum<vi>)
        n381 = control-ref of="Acquire Live Data 9237"() -> (w885:refnum<vi>)
        n382 = control-ref of="Acquire Live Data 9222"() -> (w884:refnum<vi>)
        n383 = Build Array "Controls to Enable"(w907, w905, w887, w885, w884) -> (w891:refnum<vi>[])
        n384 = call "Set Enable State on Multiple Controls.vi"("Enable?"=TRUE, "Controls"=w891) -> ()  [unwired: 10 in]
        n385 = control-ref of="ABORT DCs"() -> (w883:refnum<vi>)
        n386 = control-ref of="MANUAL PURGE"() -> (w882:refnum<vi>)
        n387 = Build Array "Controls to Disable"(w908, w906, w904, w903, w902, w901, w900, w899, w898, w897, w896, w895, w894, w893, w892, w886, w883, w882, w881, w880) -> (w889:refnum<vi>[])
        n388 = call "Set Enable State on Multiple Controls.vi"("Enable?"=FALSE, "Controls"=w889) -> ()  [unwired: 10 in]
        n389 = call "Enqueue Message.vi"("error in (no error)"=w912, "Message"="Enable Configuration Controls", "Message Queue"=w909) -> ("error out"=w911:errorcluster)  [unwired: 7 in, 1 out]
      }
      frame "Critical Error", "Log-Only Error", "Non-Critical Error", "RT Error", "Send Error to UI" {
        # "Error - Display message in status indicator on panel.  If it's a critical error, shut down this VI with an 'Exit' message."
        n390 = case shown="Default" w921 {
          selector: w921 -> [_ w938]
          tunnel: ["UI Error" w938] -> w920
          frame Default {
          }
          frame "RT Error" {
          }
        }
        n391 = Variant To Data(error in=w934, type=errorcluster {"status"=FALSE, "code"=0, "source"=""} ("error constant"), Variant=w932) -> (data=w928:errorcluster, error out=w933:errorcluster)
        n392 = Unbundle By Name(w928) -> ("code"=w927:i32, "source"=w918:string)
        n393 = Format Date/Time String() -> (date/time string=w930:string)  [unwired: 3 in]
        n394 = Format Into String(format string="\n%s: %s %d - %s", w930, w920, w927, w918) -> (resulting string=w922:string)  [unwired: 2 in, 1 out]
        n395 = call "Enqueue Message.vi"("error in (no error)"=w933, "Message Data"=w922, "Message"="Update System Status", "Message Queue"=w925) -> ("error out"=w926:errorcluster, "dup Message Queue"=w924:refnum<queue>)  [unwired: 6 in]
        n396 = case shown="Default" w921 {
          tunnel: w926 -> [w939 w943]
          tunnel: w924 -> [_ w941]
          tunnel: [w939 w942] -> w935
          frame Default {
          }
          frame "Critical Error" {
            n397 = call "Enqueue Message.vi"("error in (no error)"=w943, "Message"="Exit", "Message Queue"=w941) -> ("error out"=w942:errorcluster)  [unwired: 7 in, 1 out]
          }
        }
      }
      frame "Update System Status" {
        # "#CodeRecommended - The code below ensures that the System Status string value does not become too large.  It uses the same maximum size as the RT error log to determine whether or not to remove the last half of the log string. Change this logic if you wish to maintain more/less of the information in the System Status string."
        # "Update System Status - Add a new string to the beginning of the System Status string on the UI."
        n398 = Variant To Data(error in=w956, type="", Variant=w953) -> (data=w950:string, error out=w954:errorcluster)
        n399 = local read "System Status"() -> (w948:string)
        n400 = global read "Global - Configuration Options.vi" "Error Log Max Size (bytes)"() -> (w946:i64)
        n401 = String Length(string=w948) -> (length=w949:i32)
        n402 = Greater?(x=w949, y=w946) -> (0:w947:bool)
        n403 = case shown="True" w947 {
          tunnel: w948 -> [w957 w961]
          tunnel: w946 -> [_ w960]
          tunnel: [w957 w962] -> w945
          frame False {
          }
          frame True {
            n404 = Divide(x=w960, y=i64 2) -> (x/y=w959:dbl)
            n405 = String Subset(string=w961, length (rest)=w959) -> (substring=w962:string)  [unwired: 1 in]
          }
        }
        n406 = Concatenate Strings(w950, w945) -> (→"System Status":string)
      }
      frame "Update System Status 9049" {
        # "#CodeRecommended - The code below ensures that the System Status string value does not become too large.  It uses the same maximum size as the RT error log to determine whether or not to remove the last half of the log string. Change this logic if you wish to maintain more/less of the information in the System Status string."
        # "Update System Status - Add a new string to the beginning of the System Status string on the UI."
        n407 = Variant To Data(error in=w975, type="", Variant=w972) -> (data=w970:string, error out=w973:errorcluster)
        n408 = local read "System Status 9049"() -> (w968:string)
        n409 = global read "Global - Configuration Options.vi" "Error Log Max Size (bytes)"() -> (w966:i64)
        n410 = String Length(string=w968) -> (length=w969:i32)
        n411 = Greater?(x=w969, y=w966) -> (0:w967:bool)
        n412 = case shown="True" w967 {
          tunnel: w968 -> [w976 w980]
          tunnel: w966 -> [_ w979]
          tunnel: [w976 w981] -> w965
          frame False {
          }
          frame True {
            n413 = Divide(x=w979, y=i64 2) -> (x/y=w978:dbl)
            n414 = String Subset(string=w980, length (rest)=w978) -> (substring=w981:string)  [unwired: 1 in]
          }
        }
        n415 = Concatenate Strings(w970, w965) -> (→"System Status 9049":string)
      }
      frame "Exit" {
        w987 = TRUE ("Stop Monitoring Loop")
        # "Close all connections"
        # "Close all connections"
        # "Stop Monitoring Loop"
        # "Stop Event Handling Loop"
        # "Release the UI Message queue reference"
        # "Stop UI Message Loop"
        # "Exit - Fire the User Event to stop the Event Handling Loop, and toggle the local variable to stop the Monitoring Loop.  This message alone causes all three loops to stop."
        n416 = global write "Global - All UI Loop Stop.vi" "All UI Loop Stop"(w987) -> ()
        n417 = call "Fire User Event - Stop.vi"("User Event - Stop"=w996) -> ("error out"=w995:errorcluster)  [unwired: 10 in]
        n418 = Release Queue(queue=w992, error in (no error)=w997) -> (error out=w993:errorcluster)  [unwired: 1 in, 2 out]
        n419 = global read "Global - UI Stream and Variable Connections.vi" "UI Command Stream"() -> (w991:refnum<k21>)
        n420 = global read "Global - UI Stream and Variable Connections.vi" "RT Message Stream"() -> (w990:refnum<k21>)
        n421 = global read "Global - UI Stream and Variable Connections.vi" "Variable References"() -> (w989:T42)
        n422 = call "Enqueue Message.vi"("Priority Message? (F)"=w987, "Message"="Exit", "Message Queue"=w985) -> ()  [unwired: 7 in, 2 out]
        n423 = Destroy Stream Endpoint(11:w991) -> ()  [unwired: 1 in, 1 out]
        n424 = Destroy Stream Endpoint(11:w990) -> ()  [unwired: 1 in, 1 out]
        n425 = call "Close Variable Connections.vi"("Variable References"=w989) -> ()  [unwired: 11 in]
        n426 = global read "Global - UI Stream and Variable Connections.vi" "Variable References 9049"() -> (w982:T43)
        n427 = global read "Global - UI Stream and Variable Connections.vi" "UI Command Stream 9049"() -> (w983:refnum<k21>)
        n428 = global read "Global - UI Stream and Variable Connections.vi" "RT Message Stream 9049"() -> (w984:refnum<k21>)
        n429 = call "Close Variable Connections 9049.vi"("Variable References 9049"=w982) -> ()  [unwired: 11 in]
        n430 = Destroy Stream Endpoint(11:w983) -> ()  [unwired: 1 in, 1 out]
        n431 = Destroy Stream Endpoint(11:w984) -> ()  [unwired: 1 in, 1 out]
        n432 = Merge Errors(w995, w993) -> (w998:errorcluster)
      }
      frame "---Copy This Frame---" {
        # "Duplicate this frame when creating new messages.  Change this comment in the duplicated frame to describe this message."
        n433 = Merge Errors(w1003) -> (w1002:errorcluster)
      }
      frame "Auto P&D No Start", "Request UI to DC LNG", "Request UI to DC LOX" {
        # "POP up windows during AUTO P&D"
        n434 = case shown="\"Request UI to DC LOX\"" w1005 {
          tunnel: w1004 -> [_ _ w1012 w1025]
          frame "False", Default {
          }
          frame "Auto P&D No Start" {
            n435 = One Button Dialog(message="Auto P&D did not start. Must have VCVs in CLOSED position and Closed prox must register on. Must Have BVs in OPEN position and open prox must register on. ", button name ("OK")="WHOOPS") -> ()  [unwired: 1 out]
          }
          frame "Request UI to DC LNG" {
            n436 = call <vilib>:"Three Button Dialog.vi"("Window Title (\"\")"="DECOUPLE LNG?" ("Window Title (\"\")"), "Right Button Text (\"Cancel\")"="ABORT PROCESS" ("Right Button Text (\"Cancel\")"), "Center Button Text (\"No\")"="Repeat Purge" ("Center Button Text (\"No\")"), "Left Button Text (\"Yes\")"="Decouple" ("Left Button Text (\"Yes\")"), "message"="LNG downstream purge complete. Decouple LNG fill line?") -> ("Which Button?"=w1013:T45)  [unwired: 6 in]
            n437 = case shown="\"Left Button\", Default" w1013 {
              tunnel: w1012 -> [w1020 w1021 w1023 _]
              frame "Left Button", Default {
                n438 = call "Enqueue Message.vi"("Message"="Auto Disconnect LNG", "Message Queue"=w1020) -> ()  [unwired: 8 in, 2 out]
              }
              frame "Center Button" {
                n439 = call "Enqueue Message.vi"("Message"="LNG DS Purge", "Message Queue"=w1021) -> ()  [unwired: 8 in, 2 out]
              }
              frame "Right Button" {
                n440 = call "Enqueue Message.vi"("Message"="Abort", "Message Queue"=w1023) -> ()  [unwired: 8 in, 2 out]
              }
              frame "Window Close" {
              }
            }
          }
          frame "Request UI to DC LOX" {
            n441 = call <vilib>:"Three Button Dialog.vi"("Window Title (\"\")"="DECOUPLE LOX?" ("Window Title (\"\")"), "Right Button Text (\"Cancel\")"="ABORT PROCESS" ("Right Button Text (\"Cancel\")"), "Center Button Text (\"No\")"="Repeat Purge" ("Center Button Text (\"No\")"), "Left Button Text (\"Yes\")"="Decouple" ("Left Button Text (\"Yes\")"), "message"="LOX downstream purge complete. Decouple LOX fill line?") -> ("Which Button?"=w1026:T45)  [unwired: 6 in]
            n442 = case shown="\"Left Button\", Default" w1026 {
              tunnel: w1025 -> [w1033 w1034 w1036 _]
              frame "Left Button", Default {
                n443 = call "Enqueue Message.vi"("Message"="Auto Disconnect LOX", "Message Queue"=w1033) -> ()  [unwired: 8 in, 2 out]
              }
              frame "Center Button" {
                n444 = call "Enqueue Message.vi"("Message"="LOX DS Purge", "Message Queue"=w1034) -> ()  [unwired: 8 in, 2 out]
              }
              frame "Right Button" {
                n445 = call "Enqueue Message.vi"("Message"="Abort ", "Message Queue"=w1036) -> ()  [unwired: 8 in, 2 out]
              }
              frame "Window Close" {
              }
            }
          }
        }
        n446 = Merge Errors(w1009) -> (w1008:errorcluster)
      }
      frame "LNG DC Complete", "LOX DC Complete", "Manual LNG DC Complete", "Manual LOX DC Complete", "Manual NGV DC Complete", "System Lockup Complete" {
        # "POP up windows during AUTO P&D"
        n447 = case shown="\"Manual NGV DC Complete\"" w1039 {
          tunnel: w1038 -> [_ _ _ _ _ w1050 w1057]
          frame "False", Default {
          }
          frame "System Lockup Complete" {
            n448 = One Button Dialog(message="Auto P&D Complete.\nSystem pressurized and locked up.") -> ()  [unwired: 1 in, 1 out]
          }
          frame "Manual LNG DC Complete" {
            n449 = One Button Dialog(message="Manual LNG Decoupling Complete") -> ()  [unwired: 1 in, 1 out]
          }
          frame "Manual LOX DC Complete" {
            n450 = One Button Dialog(message="Manual LOX Decoupling Complete") -> ()  [unwired: 1 in, 1 out]
          }
          frame "Manual NGV DC Complete" {
            n451 = One Button Dialog(message="Manual NGV Decoupling Complete") -> ()  [unwired: 1 in, 1 out]
          }
          frame "LNG DC Complete" {
            n452 = Two Button Dialog(message="LNG Decouple Complete. Continue to LOX purge and DC?" ("Window Title (\"\")")) -> (T button?=w1049:bool)  [unwired: 2 in]
            n453 = case shown="True" w1049 {
              tunnel: w1050 -> [w1052 w1053]
              frame True {
                n454 = call "Enqueue Message.vi"("Message"="LOX Partial Purge", "Message Queue"=w1052) -> ()  [unwired: 8 in, 2 out]
              }
              frame False {
                n455 = call "Enqueue Message.vi"("Message"="Abort", "Message Queue"=w1053) -> ()  [unwired: 8 in, 2 out]
              }
            }
          }
          frame "LOX DC Complete" {
            n456 = Two Button Dialog(message="LOX Decouple Complete. Purge remaining lines and decouple NGV?" ("Window Title (\"\")")) -> (T button?=w1055:bool)  [unwired: 2 in]
            n457 = case shown="True" w1055 {
              tunnel: w1057 -> [w1058 w1061]
              frame False {
                n458 = call "Enqueue Message.vi"("Message"="Abort ", "Message Queue"=w1058) -> ()  [unwired: 8 in, 2 out]
              }
              frame True {
                n459 = call "Enqueue Message.vi"("Message"="Upstream Purge", "Message Queue"=w1061) -> ()  [unwired: 8 in, 2 out]
              }
            }
          }
        }
        n460 = Merge Errors(w1043) -> (w1042:errorcluster)
      }
      frame Default {
        # "'Default' case only runs if there is a message that isn't defined in any of the other cases.  Output a programming error."
        n461 = Format Into String(format string="The invalid message string \"%s\" was received in the Message Handling Loop." ("Invalid Message Loop Message"), w1067) -> (resulting string=w1064:string)  [unwired: 2 in, 1 out]
        n462 = call <vilib>:"Error Cluster From Error Code.vi"("error message (\"\")"=w1064, "error code (0)"=1) -> ("error out"=w1065:errorcluster)  [unwired: 7 in]
      }
    }
    n463 = call <vilib>:"Clear Errors.vi"("error in (no error)"=w32) -> ("error out"=w31:errorcluster)  [unwired: 5 in, 1 out]
    n464 = case shown="\"False\", Default" w27 {
      tunnel: w33 -> [w43 w45 w47]
      tunnel: w32 -> [w42 w44 w46]
      frame "Read Single Element from Stream in UI - Read Stream from RT 9049.vi->UI Main.vi" {
        n465 = call "UI Error Handler 9049 CC- Message Handler.vi"("error in (no error)"=w42, "Message Queue"=w43) -> ()  [unwired: 9 in, 1 out]
      }
      frame "Read Single Element from Stream in UI - Read Stream from RT.vi->UI Main.vi" {
        n466 = call "UI Error Handler 9039 CC- Message Handler.vi"("error in (no error)"=w44, "Message Queue"=w45) -> ()  [unwired: 9 in, 1 out]
      }
      frame "False", Default {
        n467 = call "UI Error Handler - Message Handler.vi"("error in (no error)"=w46, "Message Queue"=w47) -> ()  [unwired: 9 in, 1 out]
      }
    }
  }
  n468 = while {
    tunnel: w3 -> [w1069]
    tunnel: [w1072] -> w23
    shift-right: [w1070] -> w19
    shift-left: w11 -> [w1071]
    stop <- w1073 stop-if-true
    # "Event Handling Loop"
    n469 = event shown="[0] \"Connect to Controller 9039\": Value Change" {
      selector: w1071 -> [_ _ _ _ _ _ _ _ _ _ _ _ _ _ _ _ _ _ _ _ _ _ _ _ _ _ _ _ _ _ _ _ _ _ _ _ _ _]
      dyn-events: [_ _ _ _ _ _ _ _ _ _ _ _ _ _ _ _ _ _ _ _ _ _ _ _ _ _ _ _ _ _ _ _ _ _ _ _ _ _] -> w1070
      timeout: _ -> [_ _ _ _ _ _ _ _ _ _ _ _ _ _ _ _ _ _ _ _ _ _ _ _ _ _ _ _ _ _ _ _ _ _ _ _ _ _]
      tunnel: [_ _ _ _ _ _ _ _ _ _ _ _ _ _ _ _ _ _ _ _ _ _ _ _ _ _ _ _ _ _ _ _ _ _ _ _ _ TRUE ("Discard?")] -> w1074
      tunnel: w1069 -> [w1080 w1084 w1087 w1090 w1093 w1097 w1102 w1105 w1110 w1114 w1118 w1122 w1126 w1130 _ _ _ w1161 w1165 w1170 w1172 w1193 w1196 w1200 w1204 w1208 w1212 w1216 w1220 w1223 w1227 w1230 w1233 w1236 w1239 w1242 w1248 _]
      tunnel: [w1082 w1086 w1089 w1092 w1095 w1099 w1104 w1107 w1109 w1113 w1117 w1121 w1125 w1129 w1132 w1142 w1151 w1160 w1164 w1169 w1171 w1191 w1194 w1199 w1203 w1207 w1211 w1215 w1219 w1226 w1229 w1232 w1235 w1238 w1241 w1244 w1249 _] -> w1072
      tunnel: w1069 -> [_ _ _ _ _ _ _ _ _ _ _ _ _ _ w1133 w1143 w1152 _ _ _ _ _ _ _ _ _ _ _ _ _ _ _ _ _ _ _ _ _]
      event "Connect to Controller 9039": Value Change {
        n470 = event-data() -> ()  [unwired: 1 in, 1 out]
        n471 = call "Enqueue Message.vi"("Message"="Connect 9039", "Message Queue"=w1080) -> ("error out"=w1082:errorcluster)  [unwired: 8 in, 1 out]
      }
      event "Connected 9039?": Value Change {
        n472 = event-data() -> ()  [unwired: 1 in, 1 out]
        n473 = call "Enqueue Message.vi"("Message Data"="Expansion Chassis?", "Message"="Expansion Chassis", "Message Queue"=w1084) -> ("error out"=w1086:errorcluster)  [unwired: 7 in, 1 out]
      }
      event "Connect to Controller 9049": Value Change {
        n474 = event-data() -> ()  [unwired: 1 in, 1 out]
        n475 = call "Enqueue Message.vi"("Message"="Connect 9049", "Message Queue"=w1087) -> ("error out"=w1089:errorcluster)  [unwired: 8 in, 1 out]
      }
      event "Run Manual": Value Change {
        n476 = event-data() -> ()  [unwired: 1 in, 1 out]
        n477 = call "Enqueue Message.vi"("Message"="Run Manual", "Message Queue"=w1090) -> ("error out"=w1092:errorcluster)  [unwired: 8 in, 1 out]
      }
      event "Stop Manual": Value Change {
        n478 = event-data() -> ()  [unwired: 1 in, 1 out]
        n479 = call "Enqueue Message.vi"("Message"="Stop Manual", "Message Queue"=w1093) -> ("error out"=w1095:errorcluster)  [unwired: 8 in, 1 out]
      }
      event "Run Control": Value Change {
        n480 = event-data() -> ()  [unwired: 1 in, 1 out]
        n481 = call "Enqueue Message.vi"("Message"="Run Control", "Message Queue"=w1097) -> ("error out"=w1099:errorcluster)  [unwired: 8 in, 1 out]
        "Boolean" <- "Run Control"
      }
      event "Stop Control": Value Change {
        n482 = event-data() -> ()  [unwired: 1 in, 1 out]
        n483 = Not(x="Stop Control") -> (.not. x?=w1100:bool)
        n484 = local write "Boolean"(w1100) -> ()
        n485 = call "Enqueue Message.vi"("Message"="Stop Control", "Message Queue"=w1102) -> ("error out"=w1104:errorcluster)  [unwired: 8 in, 1 out]
      }
      event "Switch to Safe State": Value Change {
        n486 = event-data() -> ()  [unwired: 1 in, 1 out]
        n487 = call "Enqueue Message.vi"("Message"="Run Safe State", "Message Queue"=w1105) -> ("error out"=w1107:errorcluster)  [unwired: 8 in, 1 out]
      }
      event "FILL VALVES": Value Change {
        n488 = event-data() -> ()  [unwired: 1 in, 1 out]
        n489 = call "Enqueue Message.vi"("Message Data"="FILL VALVES", "Message"="Update Fill Valves", "Message Queue"=w1110) -> ("error out"=w1109:errorcluster)  [unwired: 7 in, 1 out]
      }
      event "MANUAL PURGE": Value Change {
        n490 = event-data() -> ()  [unwired: 1 in, 1 out]
        n491 = call "Enqueue Message.vi"("Message Data"="MANUAL PURGE", "Message"="MANUAL PURGE", "Message Queue"=w1114) -> ("error out"=w1113:errorcluster)  [unwired: 7 in, 1 out]
      }
      event "ARM": Value Change {
        n492 = event-data() -> ()  [unwired: 1 in, 1 out]
        n493 = call "Enqueue Message.vi"("Message Data"="ARM", "Message"="Arm", "Message Queue"=w1118) -> ("error out"=w1117:errorcluster)  [unwired: 7 in, 1 out]
      }
      event "ABORT DCs": Value Change {
        n494 = event-data() -> ()  [unwired: 1 in, 1 out]
        n495 = call "Enqueue Message.vi"("Message Data"="ABORT DCs", "Message"="abort", "Message Queue"=w1122) -> ("error out"=w1121:errorcluster)  [unwired: 7 in, 1 out]
      }
      event Value Change {
        n496 = event-data() -> ()  [unwired: 1 in, 1 out]
        n497 = call "Enqueue Message.vi"("Message Data"="VENT SYSTEM", "Message"="Update Vent System", "Message Queue"=w1126) -> ("error out"=w1125:errorcluster)  [unwired: 7 in, 1 out]
      }
      event "NGV_N2": Value Change {
        n498 = event-data() -> ()  [unwired: 1 in, 1 out]
        n499 = call "Enqueue Message.vi"("Message Data"="NGV_N2", "Message"="Update NG_PVC_BV", "Message Queue"=w1130) -> ("error out"=w1129:errorcluster)  [unwired: 7 in, 1 out]
      }
      event Value Change {
        n500 = event-data() -> ()  [unwired: 1 in, 1 out]
        n501 = Unbundle By Name("DECOUPLERS") -> ("LNG_DC"=w1136:bool)
        n502 = case shown="True" w1136 {
          tunnel: "DECOUPLERS" -> [_ w1140]
          tunnel: "Disconnect LNG" ("Message") -> [_ w1139]
          tunnel: w1133 -> [_ w1138]
          tunnel: [_ w1137] -> w1132
          frame False {
          }
          frame True {
            n503 = call "Enqueue Message.vi"("Message Data"=w1140, "Message"=w1139, "Message Queue"=w1138) -> ("error out"=w1137:errorcluster)  [unwired: 7 in, 1 out]
          }
        }
      }
      event Value Change {
        n504 = event-data() -> ()  [unwired: 1 in, 1 out]
        n505 = local read "DECOUPLERS"() -> (w1141:T11)
        n506 = Unbundle By Name(w1141) -> ("LOX_DC"=w1145:bool)
        n507 = case shown="True" w1145 {
          tunnel: w1141 -> [_ w1149]
          tunnel: "Disconnect LOX" ("Message") -> [_ w1148]
          tunnel: w1143 -> [_ w1147]
          tunnel: [_ w1146] -> w1142
          frame False {
          }
          frame True {
            n508 = call "Enqueue Message.vi"("Message Data"=w1149, "Message"=w1148, "Message Queue"=w1147) -> ("error out"=w1146:errorcluster)  [unwired: 7 in, 1 out]
          }
        }
      }
      event Value Change {
        n509 = event-data() -> ()  [unwired: 1 in, 1 out]
        n510 = local read "DECOUPLERS"() -> (w1150:T11)
        n511 = Unbundle By Name(w1150) -> ("NGV_DC"=w1154:bool)
        n512 = case shown="True" w1154 {
          tunnel: w1150 -> [_ w1158]
          tunnel: "Disconnect NGV" ("Message") -> [_ w1157]
          tunnel: w1152 -> [_ w1156]
          tunnel: [_ w1155] -> w1151
          frame False {
          }
          frame True {
            n513 = call "Enqueue Message.vi"("Message Data"=w1158, "Message"=w1157, "Message Queue"=w1156) -> ("error out"=w1155:errorcluster)  [unwired: 7 in, 1 out]
          }
        }
      }
      event Value Change {
        n514 = event-data() -> ()  [unwired: 1 in, 1 out]
        n515 = call "Enqueue Message.vi"("Message Data"="LNG PURGE", "Message"="Update LNG Purge System", "Message Queue"=w1161) -> ("error out"=w1160:errorcluster)  [unwired: 7 in, 1 out]
      }
      event Value Change {
        n516 = event-data() -> ()  [unwired: 1 in, 1 out]
        n517 = call "Enqueue Message.vi"("Message Data"="LOX PURGE", "Message"="Update LOX Purge System", "Message Queue"=w1165) -> ("error out"=w1164:errorcluster)  [unwired: 7 in, 1 out]
      }
      event Value Change {
        n518 = event-data() -> ()  [unwired: 1 in, 1 out]
        n519 = call "Enqueue Message.vi"("Message Data"="Raw Values", "Message"="Update Manual Values", "Message Queue"=w1170) -> ("error out"=w1169:errorcluster)  [unwired: 7 in, 1 out]
      }
      event "TTL Signals": Value Change {
        n520 = event-data() -> ()  [unwired: 1 in, 1 out]
        n521 = Unbundle By Name("TTL Signals") -> ("Cameras"=w1175:bool, "Spectrometer"=w1174:bool, "Ignitor"=w1173:bool)
        n522 = case shown="True" w1174 {
          tunnel: w1172 -> [_ w1182]
          frame False {
          }
          frame True {
            n523 = call "Enqueue Message.vi"("Message"="Manual Spectrometer TTL", "Message Queue"=w1182) -> ()  [unwired: 8 in, 2 out]
          }
        }
        n524 = case shown="True" w1173 {
          tunnel: w1172 -> [_ w1180]
          frame False {
          }
          frame True {
            n525 = call "Enqueue Message.vi"("Message"="Manual Ignitor TTL", "Message Queue"=w1180) -> ()  [unwired: 8 in, 2 out]
          }
        }
        n526 = case shown="True" w1175 {
          tunnel: w1172 -> [_ w1179]
          tunnel: [_ w1177] -> w1171
          frame False {
          }
          frame True {
            n527 = call "Enqueue Message.vi"("Message"="Manual Camera TTL", "Message Queue"=w1179) -> ("error out"=w1177:errorcluster)  [unwired: 8 in, 1 out]
          }
        }
      }
      event Value Change {
        n528 = event-data() -> ()  [unwired: 1 in, 1 out]
        n529 = Unbundle By Name("Pessure PID") -> ("Set Point [psi]"=w1188:dbl, "Proportional (K)"=w1187:dbl, "Integral (I)"=w1186:dbl, "Derivative (D)"=w1185:dbl)
        n530 = Bundle By Name(cluster=T20 {"Set Point [psi]"=0.0, "Proportional (K)"=0.0, "Integral (I)"=0.0, "Derivative (D)"=0.0} ("Pessure PID"), "Set Point [psi]"=w1188, "Proportional (K)"=w1187, "Integral (I)"=w1186, "Derivative (D)"=w1185) -> (w1189:T20)
        n531 = call "Enqueue Message.vi"("Message Data"=w1189, "Message"="Update Tank Pressure", "Message Queue"=w1193) -> ("error out"=w1191:errorcluster)  [unwired: 7 in, 1 out]
      }
      event "Pressure\nControl": Value Change {
        n532 = event-data() -> ()  [unwired: 1 in, 1 out]
        n533 = call "Enqueue Message.vi"("Message"="Enable Tank Pressure", "Message Queue"=w1196) -> ("error out"=w1194:errorcluster)  [unwired: 8 in, 1 out]
      }
      event "Record Button": Value Change {
        n534 = event-data() -> ()  [unwired: 1 in, 1 out]
        n535 = call "Enqueue Message.vi"("Message Data"="Record Button", "Message"="Record System", "Message Queue"=w1200) -> ("error out"=w1199:errorcluster)  [unwired: 7 in, 1 out]
      }
      event "Save As Button": Value Change {
        n536 = event-data() -> ()  [unwired: 1 in, 1 out]
        n537 = call "Enqueue Message.vi"("Message Data"="Save As Button", "Message"="Set File Path", "Message Queue"=w1204) -> ("error out"=w1203:errorcluster)  [unwired: 7 in, 1 out]
      }
      event "9237 Live Data Channel 9039": Value Change {
        n538 = event-data() -> ()  [unwired: 1 in, 1 out]
        n539 = call "Enqueue Message.vi"("Message Data"="9237 Live Data Channel 9039", "Message"="Live Channel Change 9237", "Message Queue"=w1208) -> ("error out"=w1207:errorcluster)  [unwired: 7 in, 1 out]
      }
      event "9237 Live Data Channel 9049": Value Change {
        n540 = event-data() -> ()  [unwired: 1 in, 1 out]
        n541 = call "Enqueue Message.vi"("Message Data"="9237 Live Data Channel 9049", "Message"="Live Channel Change 9237 9049", "Message Queue"=w1212) -> ("error out"=w1211:errorcluster)  [unwired: 7 in, 1 out]
      }
      event "9222 Live Data Channel 9039": Value Change {
        n542 = event-data() -> ()  [unwired: 1 in, 1 out]
        n543 = call "Enqueue Message.vi"("Message Data"="9222 Live Data Channel 9039", "Message"="Live Channel Change 9222", "Message Queue"=w1216) -> ("error out"=w1215:errorcluster)  [unwired: 7 in, 1 out]
      }
      event "9222 Live Data Channel 9049": Value Change {
        n544 = event-data() -> ()  [unwired: 1 in, 1 out]
        n545 = call "Enqueue Message.vi"("Message Data"="9222 Live Data Channel 9049", "Message"="Live Channel Change 9222 9049", "Message Queue"=w1220) -> ("error out"=w1219:errorcluster)  [unwired: 7 in, 1 out]
      }
      event "Exit": Value Change {
        w1224 = TRUE  # Priority Message
        # "The UI Message Loop handles sending the Exit message to other loops."
        n546 = event-data() -> ()  [unwired: 1 in, 1 out]
        n547 = Not(x="Exit") -> (.not. x?=w1222:bool)
        n548 = local write "Boolean"(w1222) -> ()
        n549 = call "Enqueue Message.vi"("Priority Message? (F)"=w1224, "Message"="Exit", "Message Queue"=w1223) -> ("error out"=w1226:errorcluster)  [unwired: 7 in, 1 out]
      }
      event "Stop Live Data 9039": Value Change {
        # "The UI Message Loop handles sending the Exit message to other loops."
        n550 = event-data() -> ()  [unwired: 1 in, 1 out]
        n551 = call "Enqueue Message.vi"("Message"="Stop Live Data 9039", "Message Queue"=w1227) -> ("error out"=w1229:errorcluster)  [unwired: 8 in, 1 out]
      }
      event "Stop Live Data 9049": Value Change {
        # "The UI Message Loop handles sending the Exit message to other loops."
        n552 = event-data() -> ()  [unwired: 1 in, 1 out]
        n553 = call "Enqueue Message.vi"("Message"="Stop Live Data 9049", "Message Queue"=w1230) -> ("error out"=w1232:errorcluster)  [unwired: 8 in, 1 out]
      }
      event "Acquire Live Data 9237": Value Change {
        # "The UI Message Loop handles sending the Exit message to other loops."
        n554 = event-data() -> ()  [unwired: 1 in, 1 out]
        n555 = call "Enqueue Message.vi"("Message"="Acquire Live Data 9237 9039", "Message Queue"=w1233) -> ("error out"=w1235:errorcluster)  [unwired: 8 in, 1 out]
      }
      event "Acquire Live Data 9237 9049": Value Change {
        # "The UI Message Loop handles sending the Exit message to other loops."
        n556 = event-data() -> ()  [unwired: 1 in, 1 out]
        n557 = call "Enqueue Message.vi"("Message"="Acquire Live Data 9237 9049", "Message Queue"=w1236) -> ("error out"=w1238:errorcluster)  [unwired: 8 in, 1 out]
      }
      event "Acquire Live Data 9222": Value Change {
        # "The UI Message Loop handles sending the Exit message to other loops."
        n558 = event-data() -> ()  [unwired: 1 in, 1 out]
        n559 = call "Enqueue Message.vi"("Message"="Acquire Live Data 9222 9039", "Message Queue"=w1239) -> ("error out"=w1241:errorcluster)  [unwired: 8 in, 1 out]
      }
      event "Acquire Live Data 9222 9049": Value Change {
        # "The UI Message Loop handles sending the Exit message to other loops."
        n560 = event-data() -> ()  [unwired: 1 in, 1 out]
        n561 = call "Enqueue Message.vi"("Message"="Acquire Live Data 9222 9049", "Message Queue"=w1242) -> ("error out"=w1244:errorcluster)  [unwired: 8 in, 1 out]
      }
      event "Force Trigger": Value Change {
        w1246 = u16 0 items=["Safe State", "Manual", "Control (PID)"] ("Current FPGA Control Mode 2")
        n562 = event-data() -> ()  [unwired: 1 in, 1 out]
        n563 = local read "Current FPGA Control Mode"() -> (w1247:u16)
        n564 = Equal?(x=w1246, y=w1247) -> (x = y?=w1245:bool)
        n565 = case shown="True" w1245 {
          tunnel: [w1250 w1257] -> w1249
          tunnel: w1248 -> [w1252 w1255]
          frame False {
            n566 = call "Enqueue Message.vi"("Message Data"="Cannot Start Test- Not in Safe State" ("Message"), "Message"="Update System Status", "Message Queue"=w1252) -> ("error out"=w1250:errorcluster)  [unwired: 7 in, 1 out]
          }
          frame True {
            n567 = call "Enqueue Message.vi"("Message Data"="Fire Mode", "Message"="Force Trigger", "Message Queue"=w1255) -> ("error out"=w1257:errorcluster)  [unwired: 7 in, 1 out]
          }
        }
      }
      event User Event {
        # "The Message Handling Loop processed an \"Exit\" message, which fired this event to stop the Event Handling Loop."
        n568 = event-data() -> ()  [unwired: 1 in, 1 out]
      }
    }
    n569 = case shown="No Error" w1072 {
      tunnel: [w1075 TRUE ("Discard?")] -> w1073
      tunnel: w1074 -> [w1075 _]
      tunnel: w1069 -> [_ w1076]
      frame No Error {
      }
      frame Error {
        # "On error, send Exit message, and stop loop."
        n570 = call "Enqueue Message.vi"("Priority Message? (F)"=TRUE ("Discard?"), "Message"="Exit", "Message Queue"=w1076) -> ()  [unwired: 7 in, 2 out]
      }
    }
  }
  n571 = while {
    tunnel: w3 -> [w1264]
    tunnel: u32 500 ("milliseconds to wait") -> [w1261]
    tunnel: w3 -> [w1260]
    stop <- w1265 stop-if-true
    # "Only read monitoring variables if the UI Main VI is connected to the RT target"
    # "Only the 'Exit' message in the UI Message Loop can stop the Monitoring Loop."
    # "Monitoring Loop"
    n572 = local read "Connected 9049?"() -> (w1262:bool)
    n573 = local read "Connected 9039?"() -> (w1263:bool)
    n574 = case shown="True" w1263 {
      tunnel: w1264 -> [_ w1515]
      tunnel: w1261 -> [w1293 w1512]
      frame False {
        n575 = Wait (ms)(milliseconds to wait=w1293) -> ()  [unwired: 1 out]
      }
      frame True {
        w1429 = sgl 0.0 ("y")
        w1438 = 105.0 ("x")
        w1443 = 90.0 ("x")
        w1440 = sgl 25.0 ("x")
        w1454 = sgl 6250.0 ("y")
        w1458 = T1 {"LNG_DST"=0.0, "LNG_DSP"=0.0, "LOX_DST"=0.0, "LOX_DSP"=0.0, "N2_PURGE [CFM]"=0.0, "LNG_USP"=0.0, "LOX_USP "=0.0, "LNG_UST"=0.0, "LOX_UST"=0.0, "LNG_MST"=0.0, "LNG_MSP"=0.0, "LOX_MST\n"=0.0, "LOX_MSP"=0.0, "LOX_DST 2"=0.0, "LNG_DST 2"=0.0, "LN2_Temp_HEX"=0.0, "LN2_Temp_Coil"=0.0, "LN2 [GPM]"=0.0}  # SYSTEM MEASUREMENTS
        # "Serialize the shared variable calls to simplify the scheduling performed by LabVIEW at runtime"
        n576 = global read "Global - UI Stream and Variable Connections.vi" "Variable References"() -> (w1514:T42)
        n577 = Unbundle By Name(w1514) -> ("CPU Usage"=w1519:refnum<k21>, "Contiguous Memory"=w1518:refnum<k21>, "Drive Space"=w1502:refnum<k21>, "Buffer Backlog"=w1501:refnum<k21>, "FPGA Mode"=w1500:refnum<k21>, "Actual Loop Period"=w1499:refnum<k21>, "System Time"=w1498:refnum<k21>, "Number of Data Files"=w1497:refnum<k21>, "VALVE POSITIONS"=w1496:refnum<k21>, "FILL VALVES IND"=w1495:refnum<k21>, "VENT SYSTEM IND"=w1494:refnum<k21>, "LNG PURGE IND"=w1493:refnum<k21>, "LOX PURGE IND"=w1492:refnum<k21>, "DECOUPLERS IND"=w1491:refnum<k21>, "SYSTEM MEASURMENTS"=w1301:refnum<k21>, "TEST TANK MEASURMENTS"=w1490:refnum<k21>, "FM indicators"=w1383:refnum<k21>, "He Flow indicator"=w1310:refnum<k21>, "Pipeline T&P"=w1305:refnum<k21>, "In tank T&P"=w1304:refnum<k21>)
        n578 = call "UI - Read Stream from RT.vi"("Message Queue"=w1515) -> ("error out"=w1517:errorcluster, "Message Received?"=w1513:bool, "dup Message Queue"=w1463:refnum<queue>)  [unwired: 8 in]
        n579 = case shown="True" w1513 {
          tunnel: w1512 -> [w1520 _]
          frame False {
            n580 = Wait (ms)(milliseconds to wait=w1520) -> ()  [unwired: 1 out]
          }
          frame True {
            # "If a message was received, immediately read again"
          }
        }
        n581 = shared-variable-read(w1519, w1517) -> (w1516:errorcluster, w1508:dbl)  [unwired: 2 out]
        "data out" <- w1508
        n582 = shared-variable-read(w1518, w1516) -> (w1507:errorcluster, →"Largest Contiguous Memory (bytes) 9039":dbl)  [unwired: 2 out]
        n583 = shared-variable-read(w1502, w1507) -> (w1506:errorcluster, w1488:dbl)  [unwired: 2 out]
        n584 = shared-variable-read(w1501, w1506) -> (w1505:errorcluster, w1489:dbl)  [unwired: 2 out]
        n585 = shared-variable-read(w1500, w1505) -> (w1504:errorcluster, →"Current FPGA Control Mode":T37)  [unwired: 2 out]
        n586 = shared-variable-read(w1499, w1504) -> (w1503:errorcluster, →"Actual Loop Period (ticks)":u32)  [unwired: 2 out]
        n587 = shared-variable-read(w1498, w1503) -> (w1511:errorcluster, →"9039 Time" →"9039 Time":timestamp)  [unwired: 2 out]
        n588 = shared-variable-read(w1497, w1511) -> (w1510:errorcluster, →"Number of FIles 9039":i32)  [unwired: 2 out]
        n589 = shared-variable-read(w1496, w1510) -> (w1481:errorcluster, w1482:T25)  [unwired: 2 out]
        n590 = shared-variable-read(w1495, w1481) -> (w1480:errorcluster, w1475:T46)  [unwired: 2 out]
        n591 = shared-variable-read(w1494, w1480) -> (w1479:errorcluster, w1462:T47)  [unwired: 2 out]
        n592 = shared-variable-read(w1493, w1479) -> (w1478:errorcluster, w1471:T7)  [unwired: 2 out]
        "LNG PURGE INDICATORS" <- w1471
        n593 = shared-variable-read(w1492, w1478) -> (w1477:errorcluster, w1472:T5)  [unwired: 2 out]
        "LOX PURGE INDICATORS" <- w1472
        n594 = shared-variable-read(w1491, w1477) -> (w1300:errorcluster, →"DECOUPLERS INDICATORS":T4)  [unwired: 2 out]
        n595 = shared-variable-read(w1301, w1300) -> (w1299:errorcluster, w1298:T1)  [unwired: 2 out]
        n596 = shared-variable-read(w1490, w1299) -> (w1384:errorcluster, w1358:T48)  [unwired: 2 out]
        "IN TANK MEASUREMENTS RAW VOLTAGE 2" <- w1358
        n597 = shared-variable-read(w1383, w1384) -> (w1311:errorcluster, w1357:T17)  [unwired: 2 out]
        n598 = shared-variable-read(w1310, w1311) -> (w1308:errorcluster, →"He Flow Indicator":T16)  [unwired: 2 out]
        n599 = shared-variable-read(w1305, w1308) -> (w1307:errorcluster, →"Pipeline T&P":T18)  [unwired: 2 out]
        n600 = shared-variable-read(w1304, w1307) -> (w1306:errorcluster, →"In Tank T&P":T19)  [unwired: 2 out]
        n601 = local write "Raw Values"(w1482) -> ()
        n602 = Unbundle By Name(w1298) -> ("LNG_DST"=w1341:sgl, "LNG_DSP"=w1342:sgl, "LOX_DST"=w1343:sgl, "LOX_DSP"=w1344:sgl, "N2_PURGE [CFM]"=w1347:sgl, "LNG_USP"=w1350:sgl, "LOX_USP"=w1353:sgl, "LNG_UST"=w1348:sgl, "LOX_UST"=w1335:sgl, "LNG_MST"=w1349:sgl, "LNG_MSP"=w1352:sgl, "LOX_MST"=w1334:sgl, "LOX_MSP"=w1354:sgl, "LOX_DST 2"=w1355:sgl, "LNG_DST 2"=w1351:sgl)
        n603 = Unbundle By Name(w1357) -> ("LNG_FMT [F]"=w1337:sgl, "LOX_FMT [F]"=w1338:sgl, "LOX_FMP [psi]"=w1340:sgl, "LNG_FMP [psi]"=w1339:sgl, "LOX_FMF [GPM]"=w1346:sgl, "LNG_FMF [GPM]"=w1345:sgl)
        n604 = Bundle(w1508, "Double"=w1488, "Double"=w1489) -> (→"Resource Utilization (%) 9039":cluster{dbl, "Double":dbl, "Double":dbl})  [unwired: 1 in]
        n605 = Unbundle By Name(w1462) -> ("LNG_BFV_CLOSE"=w1460:bool, "LOX_BFV_CLOSE"=w1459:bool, "LNG_BFV_OPEN"=w1296:bool, "LOX_BFV_OPEN"=w1295:bool)
        n606 = Unbundle By Name(w1357) -> ("LNG_FMT [F]"=w1382:sgl, "LOX_FMT [F]"=w1381:sgl, "LOX_FMP [psi]"=w1379:sgl, "LNG_FMP [psi]"=w1380:sgl, "LOX_FMF [GPM]"=w1378:sgl, "LNG_FMF [GPM]"=w1377:sgl)
        n607 = local read "System Measurements"() -> (w1324:T1)
        n608 = Unbundle By Name(w1298) -> ("LNG_DST"=w1373:sgl, "LNG_DSP"=w1374:sgl, "LOX_DST"=w1375:sgl, "LOX_DSP"=w1376:sgl, "N2_PURGE [CFM]"=w1457:sgl, "LNG_USP"=w1414:sgl, "LNG_MSP"=w1413:sgl, "LOX_USP"=w1412:sgl, "LOX_MSP"=w1411:sgl, "LNG_UST"=w1424:sgl, "LNG_MST"=w1423:sgl, "LNG_DST 2"=w1422:sgl, "LOX_UST"=w1421:sgl, "LOX_MST"=w1420:sgl, "LOX_DST 2"=w1419:sgl)
        n609 = local read "FM Meausrements"() -> (w1332:T17)
        n610 = Unbundle By Name(w1472) -> ("LOX_USP1"=→"LOX USP1 hide":bool, "LOX_DSP1"=→"LOX DSP1 hide":bool)
        n611 = Unbundle By Name(w1471) -> ("LNG_USP1"=→"LNG USP1 hide":bool, "LNG_DSP1"=→"LNG DSP1 hide":bool)
        n612 = Bundle By Name(cluster=T26 {"LNG_FMT"=0.0, "LOX_FMT"=0.0, "LNG_FMP"=0.0, "LOX_FMP"=0.0, "LNG_DST"=0.0, "LNG_DSP"=0.0, "LOX_DST"=0.0, "LOX_DSP"=0.0, "LNG_FLOW [GPM]"=0.0, "LOX_FLOW [GPM]"=0.0, "N2_PURGE [CFM]"=0.0, "LNG_UST"=0.0, "LNG_MST"=0.0, "LNG_USP"=0.0, "LNG_DST 2"=0.0, "LNG_MSP"=0.0, "LOX_USP"=0.0, "LOX_MSP"=0.0, "LOX_DST 2"=0.0, "LOX_UST"=0.0, "LOX_MST"=0.0} ("SYSTEM MEASUREMENTS RAW VOLTAGE and CURRENT 2"), "LNG_FMT"=w1337, "LOX_FMT"=w1338, "LNG_FMP"=w1339, "LOX_FMP"=w1340, "LNG_DST"=w1341, "LNG_DSP"=w1342, "LOX_DST"=w1343, "LOX_DSP"=w1344, "LNG_FLOW [GPM]"=w1345, "LOX_FLOW [GPM]"=w1346, "N2_PURGE [CFM]"=w1347, "LNG_UST"=w1348, "LNG_MST"=w1349, "LNG_USP"=w1350, "LNG_DST 2"=w1351, "LNG_MSP"=w1352, "LOX_USP"=w1353, "LOX_MSP"=w1354, "LOX_DST 2"=w1355, "LOX_UST"=w1335, "LOX_MST"=w1334) -> (→"SYSTEM MEASUREMENTS RAW VOLTAGE and CURRENT":T26)
        n613 = Bundle By Name(cluster=T8 {"LNG_BFV_CLOSE"=FALSE, "LOX_BFV_CLOSE"=FALSE, "LNG_BFV_OPEN"=FALSE, "LOX_BFV_OPEN"=FALSE} ("VENT SYSTEM INDICATORS 2"), "LNG_BFV_CLOSE"=w1460, "LOX_BFV_CLOSE"=w1459, "LNG_BFV_OPEN"=w1296, "LOX_BFV_OPEN"=w1295) -> (→"VENT SYSTEM INDICATORS":T8)
        n614 = local read "Fill Valves INDICATORS"() -> (w1466:T13)
        n615 = call "Flow Meter Temp Conversion.vi"("LOX Current In"=w1381, "LNG Current In"=w1382) -> ("LOX TEMP [F]"=w1364:dbl, "LNG  TEMP [F]"=w1365:dbl)  [unwired: 8 in]
        n616 = call "Flow Meter Pressure Conversion.vi"("LOX Current In"=w1379, "LNG Current In"=w1380) -> ("LOX Pressure [PSI]"=w1363:dbl, "LNG Pressure [PSI]"=w1362:dbl)  [unwired: 8 in]
        n617 = call "Flow Meter Flow Conversion.vi"("LOX Current In"=w1378, "LNG Current In"=w1377) -> ("LOX Flow [GPM]"=w1361:dbl, "LNG Flow [GPM]"=w1360:dbl)  [unwired: 8 in]
        n618 = call "UI Error Handler - Monitoring 9039.vi"("error in (no error)"=w1306, "Message Queue"=w1463) -> ()  [unwired: 9 in, 1 out]
        n619 = Unbundle By Name(w1324) -> ("LNG_DST 2"=w1323:sgl, "LNG_DSP"=w1322:sgl, "LOX_DST 2"=w1317:sgl, "LOX_DSP"=w1316:sgl, "LNG_MST"=w1319:sgl, "LNG_MSP"=w1318:sgl, "LOX_MST"=w1312:sgl, "LOX_MSP"=w1313:sgl, "LNG_UST"=w1321:sgl, "LNG_USP"=w1320:sgl, "LOX_USP"=w1314:sgl, "LOX_UST"=w1315:sgl)
        n620 = call "Pipe Pressure Conversion.vi"("LOX_MSP"=w1411, "LOX_USP"=w1412, "LNG_MSP"=w1413, "LNG_USP"=w1414) -> ("LOX_MSP"=w1407:dbl, "LOX_USP"=w1408:dbl, "LNG_MSP"=w1409:dbl, "LNG_USP"=w1410:dbl)  [unwired: 4 in]
        n621 = call "Omega Pressure Trans Conversion.vi"("LOX DSP V Offset"="LOX DSP Voltage Offset", "LNG DSP V Offset"="LNG DSP Voltage Offset", "LOX DSP Voltage In"=w1376, "LOX DST Voltage In"=w1375, "LNG DSP Voltage In"=w1374, "LNG DST Voltage In"=w1373) -> ("LOX DSP"=w1369:dbl, "LOX DST [F]"=w1370:dbl, "LNG  DSP"=w1371:dbl, "LNG  DST [F]"=w1372:dbl)  [unwired: 2 in]
        n622 = call "NITROGEN Flow Meter Conversion.vi"("N2 V offset"="N2 Voltage Offset", "N2 Flow Vin"=w1457) -> ("N2 Flow CFM"=w1456:dbl)  [unwired: 9 in]
        n623 = call "RTD Temp Conversion.vi"("LNG_UST"=w1424, "LNG_MST"=w1423, "LNG_DST"=w1422, "LOX_UST"=w1421, "LOX_MST"=w1420, "LOX_DST"=w1419) -> ("LNG_UST"=w1418:dbl, "LNG_MST"=w1417:dbl, "LNG_DST"=w1404:dbl, "LOX_UST"=w1416:dbl, "LOX_MST"=w1415:dbl, "LOX_DST"=w1405:dbl)  [unwired: 8 in]
        n624 = Unbundle By Name(w1332) -> ("LNG_FMT [F]"=w1331:sgl, "LOX_FMT [F]"=w1330:sgl, "LOX_FMP [psi]"=w1329:sgl, "LNG_FMP [psi]"=w1328:sgl, "LOX_FMF [GPM]"=w1327:sgl, "LNG_FMF [GPM]"=w1326:sgl)
        n625 = Bundle By Name(cluster=w1458, "LNG_DST"=w1372, "LNG_DSP"=w1371, "LOX_DST"=w1370, "LOX_DSP"=w1369, "N2_PURGE [CFM]"=w1456, "LNG_USP"=w1410, "LNG_MSP"=w1409, "LOX_USP"=w1408, "LOX_MSP"=w1407, "LNG_UST"=w1418, "LNG_MST"=w1417, "LNG_DST 2"=w1404, "LOX_UST"=w1416, "LOX_MST"=w1415, "LOX_DST 2"=w1405) -> (→"System Measurements":T1)
        n626 = call "Test Tank Conversion.vi"("IN TANK MEASUREMENTS RAW VOLTAGE"=w1358, "Manual Temp Input?"="Manual Temp Input?", "Tank Type"="Tank Type", "LOX Temp"=w1405, "Sensor Inputs"="Tank Sensor Adjustment", "LNG Temp"=w1404, "LNG Fraction"="LNG Fraction", "Tank Size"="Tank Size 2", "Backup Switch"="Backup Sensors") -> ("LNG Mass [lbs]"=w1386:dbl, "LOX Mass [lbs]"=w1387:dbl, "Target Mass Ratio"=→"Target Mass Ratio":dbl, "IN TANK MEASUREMENTS DEPTH INCHES"=w1393:T23, "Target LOX Height [in] (above port)"=→"Target LOX Depth [in]":dbl, "Target LNG Height [in] (above port)"=→"Target LNG Depth [in]":dbl, "LNG percent filled"=w1388:dbl, "LOX percent filled"=w1389:dbl, "Mole Unbalanced?"=→"LNG Mole Unbalanced?":bool, "Fill height in manual?"=→"Fill height in manual?":bool, "LNG UP pressure [psi]"=w1397:dbl, "LOX UP pressure [psi]"=w1396:dbl)  [unwired: 6 in, 1 out]
        "IN TANK MEASUREMENTS DEPTH INCHES" <- w1393
        "LNG Mass [lbs]" <- w1386
        "LOX Mass [lbs]" <- w1387
        n627 = Unbundle By Name(w1466) -> ("LNG_VCV_POS"=w1465:sgl, "LOX_VCV_POS"=w1464:sgl)
        n628 = Bundle By Name(cluster=T17 {"LNG_FMT [F]"=0.0, "LOX_FMT [F]"=0.0, "LOX_FMP [psi]"=0.0, "LNG_FMP [psi]"=0.0, "LOX_FMF [GPM]"=0.0, "LNG_FMF [GPM]"=0.0} ("FM Indicators"), "LNG_FMT [F]"=w1365, "LOX_FMT [F]"=w1364, "LOX_FMP [psi]"=w1363, "LNG_FMP [psi]"=w1362, "LOX_FMF [GPM]"=w1361, "LNG_FMF [GPM]"=w1360) -> (→"FM Meausrements":T17)
        n629 = Unbundle By Name(w1475) -> ("LNG_BV_OPEN"=w1447:bool, "LOX_BV_OPEN"=w1446:bool, "LNG_VCV_CLOSE"=w1449:bool, "LOX_VCV_CLOSE"=w1448:bool, "LNG_VCV_POS"=w1455:sgl, "LOX_VCV_POS"=w1453:sgl, "LNG_BV_CLOSE"=w1445:bool, "LOX_BV_CLOSE"=w1444:bool)
        "LNG BV Fill Open" <- w1447
        "LOX BV Fill Open" <- w1446
        n630 = Greater Or Equal?(x=w1389, y=w1443) -> (x >= y?=w1441:bool)
        n631 = Unbundle By Name(w1393) -> ("LNG_TANK"=w1392:dbl, "LOX_TANK"=w1391:dbl)
        n632 = Greater Or Equal?(x=w1388, y=w1438) -> (x >= y?=w1437:bool)
        n633 = Greater Or Equal?(x=w1389, y=w1438) -> (x >= y?=w1436:bool)
        n634 = Greater Or Equal?(x=w1388, y=w1443) -> (x >= y?=w1442:bool)
        n635 = Bundle("LNG_VCV_POS"=w1465, "LNG_FMF [GPM]"=w1326, "LNG_FMT [F]"=w1331, "LNG_FMP [psi]"=w1328, "LNG_DST 2"=w1323, "LNG_DSP"=w1322, "LNG_UST"=w1321, "LNG_USP"=w1320, "LNG_MST"=w1319, "LNG_MSP"=w1318) -> (→"LNG":T22)  [unwired: 1 in]
        n636 = Not(x=w1449) -> (.not. x?=→"LNG VCV Fill Close":bool)
        n637 = Not(x=w1448) -> (.not. x?=→"LOX VCV Fill Close":bool)
        n638 = Bundle By Name(cluster=T14 {"LOX_ULEGE [psi]"=-2.237651064682007, "LOX_TANK"=8.476709325018989, "LOX 90%"=FALSE, "LOX 105%"=FALSE, "Depth [in] LOX "=5.537410366568655, "LNG_TANK"=0.0, "LNG 90%"=FALSE, "LNG 105%"=FALSE, "Depth [in] LNG"=0.0, "LNG_ULEGE [psi]"=6.801481246948242} ("IN TANK MEASUREMENTS 2"), "LNG_TANK"=w1388, "LOX_TANK"=w1389, "LOX_ULEGE [psi]"=w1396, "LNG_ULEGE [psi]"=w1397, "LNG 90%"=w1442, "LOX 90%"=w1441, "LNG 105%"=w1437, "LOX 105%"=w1436, "Depth [in] LNG"=w1392, "Depth [in] LOX"=w1391) -> (→"IN TANK MEASUREMENTS":T14)
        n639 = Multiply(x=w1454, y=w1453) -> (x*y=w1439:sgl)
        n640 = Multiply(x=w1455, y=w1454) -> (x*y=w1452:sgl)
        n641 = Bundle("LOX_VCV_POS"=w1464, "LOX_FMF [GPM]"=w1327, "LOX_FMT [F]"=w1330, "LOX_FMP [psi]"=w1329, "LOX_DST 2"=w1317, "LOX_DSP"=w1316, "LOX_UST"=w1315, "LOX_USP"=w1314, "LOX_MST"=w1312, "LOX_MSP"=w1313) -> (→"LOX":T21)  [unwired: 1 in]
        n642 = Subtract(x=w1439, y=w1440) -> (x-y=w1428:sgl)
        n643 = Greater?(x=w1428, y=w1429) -> (0:w1432:bool)
        n644 = Select(t=w1428, s=w1432, f=w1429) -> (s? t:f=w1426:sgl)
        n645 = Subtract(x=w1452, y=w1440) -> (x-y=w1430:sgl)
        n646 = Greater?(x=w1430, y=w1429) -> (0:w1431:bool)
        n647 = Select(t=w1430, s=w1431, f=w1429) -> (s? t:f=w1427:sgl)
        n648 = Divide(x=w1387, y=w1386) -> (x/y=→"Actual Mass Ratio":dbl)
        n649 = Bundle By Name(cluster=T13 {"LNG_BV_CLOSE"=FALSE, "LOX_BV_CLOSE"=FALSE, "LNG_VCV_CLOSE"=FALSE, "LNG_VCV_POS"=0.0, "LOX_VCV_POS"=0.0, "LNG_BV_OPEN"=FALSE, "LOX_BV_OPEN"=FALSE, "LOX_VCV_CLOSE"=FALSE} ("Fill Valves INDICATORS"), "LNG_VCV_POS"=w1427, "LOX_VCV_POS"=w1426, "LNG_VCV_CLOSE"=w1449, "LOX_VCV_CLOSE"=w1448, "LNG_BV_OPEN"=w1447, "LNG_BV_CLOSE"=w1445, "LOX_BV_OPEN"=w1446, "LOX_BV_CLOSE"=w1444) -> (→"Fill Valves INDICATORS":T13)
        "Tank Size" <- "Tank Size 2"
      }
    }
    n650 = case shown="False" w1262 {
      tunnel: w1261 -> [w1266 w1270]
      tunnel: w1260 -> [_ w1271]
      frame False {
        n651 = Wait (ms)(milliseconds to wait=w1266) -> ()  [unwired: 1 out]
      }
      frame True {
        # "Serialize the shared variable calls to simplify the scheduling performed by LabVIEW at runtime"
        n652 = global read "Global - UI Stream and Variable Connections.vi" "Variable References 9049"() -> (w1288:T43)
        n653 = call "UI - Read Stream from RT 9049.vi"("Message Queue"=w1271) -> ("error out"=w1273:errorcluster, "Message Received?"=w1272:bool, "dup Message Queue"=w1268:refnum<queue>)  [unwired: 8 in]
        n654 = case shown="False" w1272 {
          tunnel: w1270 -> [w1292 _]
          frame False {
            n655 = Wait (ms)(milliseconds to wait=w1292) -> ()  [unwired: 1 out]
          }
          frame True {
            # "If a message was received, immediately read again"
          }
        }
        n656 = Unbundle By Name(w1288) -> ("CPU Usage 9049"=w1291:refnum<k21>, "Contiguous Memory 9049"=w1290:refnum<k21>, "Drive Space 9049"=w1282:refnum<k21>, "Buffer Backlog 9049"=w1281:refnum<k21>, "System Time 9049"=w1280:refnum<k21>, "Number of Data Files 9049"=w1279:refnum<k21>)
        n657 = shared-variable-read(w1291, w1273) -> (w1289:errorcluster, w1285:dbl)  [unwired: 2 out]
        n658 = shared-variable-read(w1290, w1289) -> (w1284:errorcluster, →"Largest Contiguous Memory (bytes) 9049":dbl)  [unwired: 2 out]
        n659 = shared-variable-read(w1282, w1284) -> (w1283:errorcluster, w1277:dbl)  [unwired: 2 out]
        n660 = shared-variable-read(w1281, w1283) -> (w1269:errorcluster, w1278:dbl)  [unwired: 2 out]
        n661 = shared-variable-read(w1280, w1269) -> (w1287:errorcluster, →"9049 Time" →"9049 Time":timestamp)  [unwired: 2 out]
        n662 = shared-variable-read(w1279, w1287) -> (w1267:errorcluster, →"Number of FIles 9049":i32)  [unwired: 2 out]
        n663 = Bundle(w1285, "Double"=w1277, "Double"=w1278) -> (→"Resource Utilization (%) 9049":cluster{dbl, "Double":dbl, "Double":dbl})  [unwired: 1 in]
        n664 = call "UI Error Handler - Monitoring 9049.vi"("error in (no error)"=w1267, "Message Queue"=w1268) -> ()  [unwired: 9 in, 1 out]
      }
    }
    n665 = case shown="True" TRUE {
      frame False {
      }
      frame True {
      }
    }
    n666 = global read "Global - All UI Loop Stop.vi" "All UI Loop Stop"() -> (w1265:bool)
  }
  n667 = Unregister For Events(event registration refnum=w19, error in=w23) -> (error out=w20:errorcluster)
  n668 = Obtain Queue(element data type=sgl[][] [] ("appended array")) -> (queue out=w2:refnum<queue>)  [unwired: 4 in, 2 out]
  n669 = Release Queue(queue=w2, error in (no error)=w5) -> (error out=w4:errorcluster)  [unwired: 1 in, 2 out]
  n670 = call "Logging Message Loop.vi"("queue out"=w2, "Message Queues"=w8) -> ("error out"=w7:errorcluster)  [unwired: 9 in]
  n671 = Merge Errors(w20, w4, w7) -> (w22:errorcluster)
  n672 = call "Destroy User Event - Stop.vi"("error in (no error)"=w22, "User Event - Stop"=w12) -> ("error out"=w17:errorcluster)  [unwired: 9 in]
  n673 = while {
    shift-right: [w1545] -> _
    shift-left: w1 -> [w1547]
    shift-right: [w1537] -> _
    shift-left: w1 -> [w1538]
    shift-right: [w1533] -> _
    shift-left: w1 -> [w1532]
    shift-right: [w1528] -> _
    shift-left: w1 -> [w1527]
    stop <- w1542 stop-if-true
    # "NEED TO PUT N2 VALUE IN WHILE LOOPS"
    # "NGV Vol = 20ft^3"
    # "LNG US pipe plus 4in round about to vent\nvolume = 50ft^3 ish"
    # "LOX US Pipe Vol = 6.5 ft^3"
    # "DS Pipe Vol= 1.6ft^3"
    # "Purge Gas Monitoring"
    n674 = case shown="False" "Reset  3" {
      tunnel: w1547 -> [w1612 _]
      tunnel: [w1612 w1613] -> w1546
      frame False {
      }
      frame True {
        w1613 = 0.0 ("Total Fill Time")
        n675 = local write "Total LNG USN2 [sec]"(w1613) -> ()
        n676 = local write "LNG UPPER VOL"(w1613) -> ()
      }
    }
    n677 = case shown="False" "Reset  4" {
      tunnel: w1538 -> [w1591 _]
      tunnel: [w1591 w1592] -> w1539
      frame False {
      }
      frame True {
        w1592 = 0.0 ("Total Fill Time")
        n678 = local write "Total LNG DSN2 [sec]"(w1592) -> ()
        n679 = local write "LNG LOWER VOL"(w1592) -> ()
      }
    }
    n680 = case shown="False" "Reset  5" {
      tunnel: w1532 -> [w1570 _]
      tunnel: [w1570 w1571] -> w1536
      frame False {
      }
      frame True {
        w1571 = 0.0 ("Total Fill Time")
        n681 = local write "Total LOX USN2 [sec]"(w1571) -> ()
        n682 = local write "LOX UPPER VOL"(w1571) -> ()
      }
    }
    n683 = case shown="False" "Reset  6" {
      tunnel: w1527 -> [w1549 _]
      tunnel: [w1549 w1550] -> w1529
      frame False {
      }
      frame True {
        w1550 = 0.0 ("Total Fill Time")
        n684 = local write "Total LOX DSN2 [sec]"(w1550) -> ()
        n685 = local write "LOX LOWER VOL"(w1550) -> ()
      }
    }
    n686 = local read "System Measurements"() -> (w1522:T1)
    n687 = local read "LNG DSP1 hide"() -> (w1541:bool)
    n688 = local read "LNG USP1 hide"() -> (w1543:bool)
    n689 = local read "LOX DSP1 hide"() -> (w1531:bool)
    n690 = local read "LOX USP1 hide"() -> (w1534:bool)
    n691 = Unbundle By Name(w1522) -> ("N2_PURGE [CFM]"=w1521:sgl)
    n692 = Add(x=w1521, y=4.59) -> (x+y=w1525:dbl)
    n693 = Multiply(x=w1525, y=10.0) -> (x*y=w1523:dbl)
    n694 = case shown="False" w1531 {
      tunnel: w1529 -> [w1551 w1555]
      tunnel: [w1551 w1553] -> w1528
      tunnel: w1523 -> [_ w1552]
      frame False {
      }
      frame True {
        n695 = Get Date/Time In Seconds() -> (seconds since 1Jan1904=w1554:timestamp)
        n696 = while {
          tunnel: w1555 -> [w1567]
          shift-right: [w1566] -> _
          shift-left: w1554 -> [w1566]
          tunnel: [w1562] -> w1553
          tunnel: w1552 -> [w1560]
          stop <- w1565 stop-if-true
          n697 = Get Date/Time In Seconds() -> (seconds since 1Jan1904=w1569:timestamp)
          n698 = Subtract(x=w1569, y=w1566) -> (x-y=w1568:dbl)
          "LOX DSN2 [sec]" <- w1568
          n699 = Add(x=w1568, y=w1567) -> (x+y=w1562:dbl)
          "Total LOX DSN2 [sec]" <- w1562
          n700 = Divide(x=w1562, y=60.0) -> (x/y=w1559:dbl)
          n701 = Multiply(x=w1559, y=w1560) -> (x*y=w1558:dbl)
          n702 = Divide(x=w1558, y=1.6) -> (x/y=→"LOX LOWER VOL":dbl)
          n703 = local read "LOX DSP1 hide"() -> (w1563:bool)
          n704 = Wait (ms)(milliseconds to wait=u32 100) -> ()  [unwired: 1 out]
          n705 = Not(x=w1563) -> (.not. x?=w1565:bool)
        }
      }
    }
    n706 = case shown="False" w1541 {
      tunnel: w1539 -> [w1593 w1597]
      tunnel: [w1593 w1595] -> w1537
      tunnel: w1523 -> [_ w1594]
      frame False {
      }
      frame True {
        n707 = Get Date/Time In Seconds() -> (seconds since 1Jan1904=w1596:timestamp)
        n708 = while {
          tunnel: w1597 -> [w1609]
          shift-right: [w1608] -> _
          shift-left: w1596 -> [w1608]
          tunnel: [w1599] -> w1595
          tunnel: w1594 -> [w1600]
          stop <- w1607 stop-if-true
          n709 = Get Date/Time In Seconds() -> (seconds since 1Jan1904=w1611:timestamp)
          n710 = Subtract(x=w1611, y=w1608) -> (x-y=w1610:dbl)
          "LNG DSN2 [sec]" <- w1610
          n711 = Add(x=w1610, y=w1609) -> (x+y=w1599:dbl)
          "Total LNG DSN2 [sec]" <- w1599
          n712 = Divide(x=w1599, y=60.0) -> (x/y=w1601:dbl)
          n713 = Multiply(x=w1601, y=w1600) -> (x*y=w1602:dbl)
          n714 = Divide(x=w1602, y=1.6) -> (x/y=→"LNG LOWER VOL":dbl)
          n715 = local read "LNG DSP1 hide"() -> (w1605:bool)
          n716 = Wait (ms)(milliseconds to wait=u32 100) -> ()  [unwired: 1 out]
          n717 = Not(x=w1605) -> (.not. x?=w1607:bool)
        }
      }
    }
    n718 = case shown="False" w1543 {
      tunnel: w1546 -> [w1614 w1618]
      tunnel: [w1614 w1616] -> w1545
      tunnel: w1523 -> [_ w1615]
      frame False {
      }
      frame True {
        n719 = Get Date/Time In Seconds() -> (seconds since 1Jan1904=w1617:timestamp)
        n720 = while {
          tunnel: w1618 -> [w1630]
          shift-right: [w1629] -> _
          shift-left: w1617 -> [w1629]
          tunnel: [w1621] -> w1616
          tunnel: w1615 -> [w1620]
          stop <- w1628 stop-if-true
          # "volume in multiples of pipe vol"
          # "change to minutes"
          n721 = Get Date/Time In Seconds() -> (seconds since 1Jan1904=w1632:timestamp)
          n722 = Subtract(x=w1632, y=w1629) -> (x-y=w1631:dbl)
          "LNG USN2 [sec]" <- w1631
          n723 = Add(x=w1631, y=w1630) -> (x+y=w1621:dbl)
          "Total LNG USN2 [sec]" <- w1621
          n724 = Divide(x=w1621, y=60.0) -> (x/y=w1622:dbl)
          n725 = Multiply(x=w1622, y=w1620) -> (x*y=w1623:dbl)
          n726 = local read "LNG USP1 hide"() -> (w1626:bool)
          n727 = Divide(x=w1623, y=20.0) -> (x/y=→"LNG UPPER VOL":dbl)
          n728 = Wait (ms)(milliseconds to wait=u32 100) -> ()  [unwired: 1 out]
          n729 = Not(x=w1626) -> (.not. x?=w1628:bool)
        }
      }
    }
    n730 = case shown="False" w1534 {
      tunnel: w1536 -> [w1572 w1576]
      tunnel: [w1572 w1574] -> w1533
      tunnel: w1523 -> [_ w1573]
      frame False {
      }
      frame True {
        n731 = Get Date/Time In Seconds() -> (seconds since 1Jan1904=w1575:timestamp)
        n732 = while {
          tunnel: w1576 -> [w1588]
          shift-right: [w1587] -> _
          shift-left: w1575 -> [w1587]
          tunnel: [w1580] -> w1574
          tunnel: w1573 -> [w1582]
          stop <- w1586 stop-if-true
          n733 = Get Date/Time In Seconds() -> (seconds since 1Jan1904=w1590:timestamp)
          n734 = Subtract(x=w1590, y=w1587) -> (x-y=w1589:dbl)
          "LOX USN2 [sec]" <- w1589
          n735 = Add(x=w1589, y=w1588) -> (x+y=w1580:dbl)
          "Total LOX USN2 [sec]" <- w1580
          n736 = Divide(x=w1580, y=60.0) -> (x/y=w1583:dbl)
          n737 = Multiply(x=w1583, y=w1582) -> (x*y=w1581:dbl)
          n738 = Divide(x=w1581, y=6.5) -> (x/y=→"LOX UPPER VOL":dbl)
          n739 = local read "LOX USP1 hide"() -> (w1584:bool)
          n740 = Wait (ms)(milliseconds to wait=u32 100) -> ()  [unwired: 1 out]
          n741 = Not(x=w1584) -> (.not. x?=w1586:bool)
        }
      }
    }
    n742 = global read "Global - All UI Loop Stop.vi" "All UI Loop Stop"() -> (w1542:bool)
    n743 = Wait (ms)(milliseconds to wait=u32 100) -> ()  [unwired: 1 out]
  }
  n744 = call <vilib>:"Simple Error Handler.vi"("error in (no error)"=w17) -> ()  [unwired: 4 in, 5 out]
  n745 = while {
    tunnel: w2 -> [w1634]
    stop <- w1635 stop-if-true
    # "Logging Loop"
    n746 = local read "Connected 9039?"() -> (w1633:bool)
    n747 = case shown="True" w1633 {
      tunnel: w1634 -> [_ w1702]
      frame False {
        n748 = Wait (ms)(milliseconds to wait=u32 500) -> ()  [unwired: 1 out]
      }
      frame True {
        w1669 = 1.0 ("f")
        w1670 = 0.0 ("t")
        (unwired) 1
        # "System Logging Loop\n1 second interval\nAll pipe system components"
        n749 = local read "System Measurements"() -> (w1659:T1)
        n750 = local read "FM Meausrements"() -> (w1658:T17)
        n751 = local read "IN TANK MEASUREMENTS DEPTH INCHES"() -> (w1695:T23)
        n752 = local read "IN TANK MEASUREMENTS RAW VOLTAGE 2"() -> (w1693:T27)
        n753 = local read "LNG Mole Unbalanced?"() -> (w1671:bool)
        n754 = local read "Fill Valves INDICATORS"() -> (w1697:T13)
        n755 = local read "IN TANK MEASUREMENTS"() -> (w1694:T14)
        n756 = local read "Fill height in manual?"() -> (w1673:bool)
        n757 = local read "LNG Mass [lbs]"() -> (w1678:dbl)
        n758 = local read "LOX Mass [lbs]"() -> (w1677:dbl)
        n759 = local read "Actual Mass Ratio"() -> (w1676:dbl)
        n760 = local read "Target LNG Depth [in]"() -> (w1675:dbl)
        n761 = local read "Target LOX Depth [in]"() -> (w1674:dbl)
        n762 = local read "Tank Size"() -> (w1667:T15)
        n763 = local read "Tank Type"() -> (w1666:T29)
        n764 = local read "Target Mass Ratio"() -> (w1665:dbl)
        n765 = shared-variable "NI-cRIO-9039-01AA2F3E\\Shared Variables.lvlib\\PID Data"() -> (w1664:T49)  [unwired: 1 in, 1 out]
        n766 = Unbundle By Name(w1658) -> ("LNG_FMT [F]"=w1642:sgl, "LOX_FMT [F]"=w1641:sgl, "LOX_FMP [psi]"=w1640:sgl, "LNG_FMP [psi]"=w1639:sgl, "LOX_FMF [GPM]"=w1638:sgl, "LNG_FMF [GPM]"=w1637:sgl)
        n767 = Unbundle By Name(w1659) -> ("LNG_DST"=w1657:sgl, "LNG_DSP"=w1651:sgl, "LOX_DST"=w1650:sgl, "LOX_DSP"=w1646:sgl, "N2_PURGE [CFM]"=w1643:sgl, "LNG_USP"=w1654:sgl, "LOX_USP"=w1644:sgl, "LNG_UST"=w1652:sgl, "LOX_UST"=w1647:sgl, "LNG_MST"=w1656:sgl, "LNG_MSP"=w1653:sgl, "LOX_MST"=w1648:sgl, "LOX_MSP"=w1645:sgl, "LOX_DST 2"=w1649:sgl, "LNG_DST 2"=w1655:sgl)
        n768 = Unbundle By Name(w1697) -> ("LNG_VCV_POS"=w1679:sgl, "LOX_VCV_POS"=w1680:sgl)
        n769 = Unbundle By Name(w1664) -> ("Setpoint [psi]"=w1663:dbl, "Diff. Pressure-Window [psi]"=w1662:dbl, "LOX_HE_MFC"=w1661:dbl, "LNG_HE_MFC"=w1660:dbl)
        n770 = Unbundle By Name(w1693) -> ("LNG_DIFF"=w1687:sgl, "LOX_DIFF"=w1688:sgl, "LOX_TANK 2"=w1689:sgl, "LNG_TANK 2"=w1690:sgl, "LOX_TANK_ULEGE"=w1691:sgl, "LOX_TANK_ULEGE 2"=w1692:sgl)
        n771 = Unbundle By Name(w1694) -> ("LNG_ULEGE [psi]"=w1685:dbl, "LOX_ULEGE [psi]"=w1686:dbl)
        n772 = Select(t=w1670, s=w1673, f=w1669) -> (s? t:f=w1672:dbl)
        n773 = Unbundle By Name(w1695) -> ("LNG_TANK"=w1681:dbl, "LOX_TANK"=w1682:dbl, "LNG_TANK 2"=w1683:dbl, "LOX_TANK 2"=w1684:dbl)
        n774 = Select(t=w1670, s=w1671, f=w1669) -> (s? t:f=w1668:dbl)
        n775 = Build Array(w1679, w1680, w1681, w1682, w1683, w1684, w1685, w1686, w1687, w1688, w1689, w1690, w1691, w1692, w1657, w1656, w1655, w1652, w1651, w1653, w1654, w1650, w1649, w1648, w1647, w1646, w1645, w1644, w1643, w1642, w1641, w1640, w1639, w1638, w1637, w1678, w1677, w1676, w1675, w1674, w1672, w1668, w1667, w1666, w1665, w1663, w1662, w1661, w1660) -> (w1701:dbl[])
        n776 = local read "Record Button"() -> (w1698:bool)
        n777 = Build Array(w1701) -> (w1700:dbl[][])
        n778 = Transpose 2D Array(2D array=w1700) -> (transposed array=w1699:dbl[][])
        n779 = Wait (ms)(milliseconds to wait=u32 1000) -> ()  [unwired: 1 out]
        n780 = case shown="False" w1698 {
          tunnel: w1702 -> [_ w1704]
          tunnel: w1699 -> [_ w1703]
          frame False {
          }
          frame True {
            n781 = Enqueue Element(queue=w1704, element=w1703) -> ()  [unwired: 2 in, 3 out]
          }
        }
      }
    }
    n782 = global read "Global - All UI Loop Stop.vi" "All UI Loop Stop"() -> (w1635:bool)
  }
